vi "Main_Marvin Remake.vi"() -> ()   [LabVIEW 2017]
uses:
  PCAN_Driver/ControlCAN.llb/DevType.ctl
  PCAN_Driver/ControlCAN.llb/CAN Channel.ctl
  PCAN_Driver/ControlCAN.llb/VCI_INIT_CONFIG.ctl
  PCAN_Driver/ControlCAN.llb/InitFlag.ctl
  PCAN_Driver/ControlCAN.llb/Fliter.ctl
  PCAN_Driver/ControlCAN.llb/Mode.ctl
  <vilib>/Utility/miscctls.llb/LVRowAndColumnTypeDef.ctl
  <vilib>/Utility/config.llb/Read Key (String).vi
  <vilib>/Utility/config.llb/Write Key (String).vi
  <vilib>/Utility/cursorutil.llb/Set Cursor (Icon Pict).vi
  PCAN_Driver/ControlCAN.lvlib
  <vilib>/Utility/config.llb/NI_LVConfig.lvlib
panel:
  out "UUT SN Report":string
  out "Automation":bool
  out "Test Failed":bool
  out "AuxiOFFResult":bool
  out "AuxiONResult":bool
  out "SensCalResult":bool
  out "VisualInspectionResult":bool
  out "BurnResult":bool
  out "BurnSpeed":bool
  out "BurnTemp":bool
  out "BurnDC":bool
  out "TempControlResult":bool
  out "MotorTempResult":bool
  out "StopTimeResult":bool
  out "SpeedResult":bool=TRUE
  out "VenableDirectionResult":bool
  out "VenableResult":bool
  out "ComTestResult":bool=TRUE
  out "UUT SoftwareVer":string
  out "Next SN":i32
  in  "SetSN":bool
  out "Current SN":i32
  out "Cal":dbl
  out "AO[1]Meas":dbl
  out "FullSpeed2 Speed":dbl
  out "FullSpeed2 Current":dbl
  out "FullSpeed1 Current":dbl
  out "FullSpeed1 Speed":dbl
  out "MaxBurnInTempVal":dbl
  in  "Stop Burn-in":bool
  out "VISA Tester":refnum<visa-resource-name>
  out "UUT":u8
  out "CAN Status":bool
  in  "Channel 2":T1 caption="Channel" items=["Channel 1", "Channel 2"]
  out "Config_CANAT":T7 {"DevType" items=["USB-CAN"=3, "USB-CAN2"=4]; "CanIndex" items=["通道1", "通道2"]; "VCI_INIT_CONFIG"."Fliter" items=["接收所有类型"=3, "只接收标准帧"=4, "只接收扩展帧"=7]; "VCI_INIT_CONFIG"."Mode" items=["正常工作", "自测模式（环回）", "仅侦听模式"]; "VCI_INIT_CONFIG"."InitFlag" items=["使用Flash参数", "使用界面设置参数"]}
  out "Array":u64[][](array[numeric]) format="%016x"
  out "Motor Phase Current RMS":dbl
  out "Ambient Temperature":dbl
  out "Speed error":bool
  out "Commutation err":bool
  out "Under voltage/Over voltage":bool
  out "Derated drive temp":bool
  out "Motor Over temperature":bool
  out "Motor Sensor temp Fauilre":bool
  out "Drive Over temperature":bool
  out "Drive Sensor temp Failure":bool
  out "Ambient Over temp":bool
  out "Ambient Sensor temp":bool
  out "DC Voltage":dbl
  out "DC Current":dbl
  out "Power transistor Heat sink Temp.":dbl
  out "Motor Stator Temp.":dbl
  out "Motor Speed RPM":dbl
  out "ECS State":u16
  out "UUT":string="EBAY"
  in  "Logger Path":path
  in  "Report":bool
  in  "Start":bool
  in  "ATR":string[][](table)=[["Test Communication", "-", "-", "-", "-", ""], ["Set S/N", "-", "-", "-", "-", ""], ["Set Board Number", "-", "-", "-", "-", ""], [" ", "", "", "", "", ""], ["Test Communication", "-", "-", "-", "-", ""], ["Get S/N", "-", "-", "-", "", ""], ["Get Board Number", "-", "-", "-", "", ""], ["Get FW", "-", "-", "-", "", ""], ["Enable Motor", "", "", "", "", ""], ["Small position command", "", "", "", "", ""], ["Measure delta", "", "", "", "", ""], ["Velocity command", "", "", "", "", ""]]
  in  "Settings":bool
  in  "Refresh Button":bool
  out "Status":bool
  in  "VISA Marvin":refnum<visa-resource-name>="COM6"
  in  "Serial Com":bool
  in  "Help Button":bool
  out "Pannel User Message":string
  in  "Stop Button":bool
  # "Marvin"
  # "REDLER TECHNOLOGIES LTD"
  # "ver 1.2i"
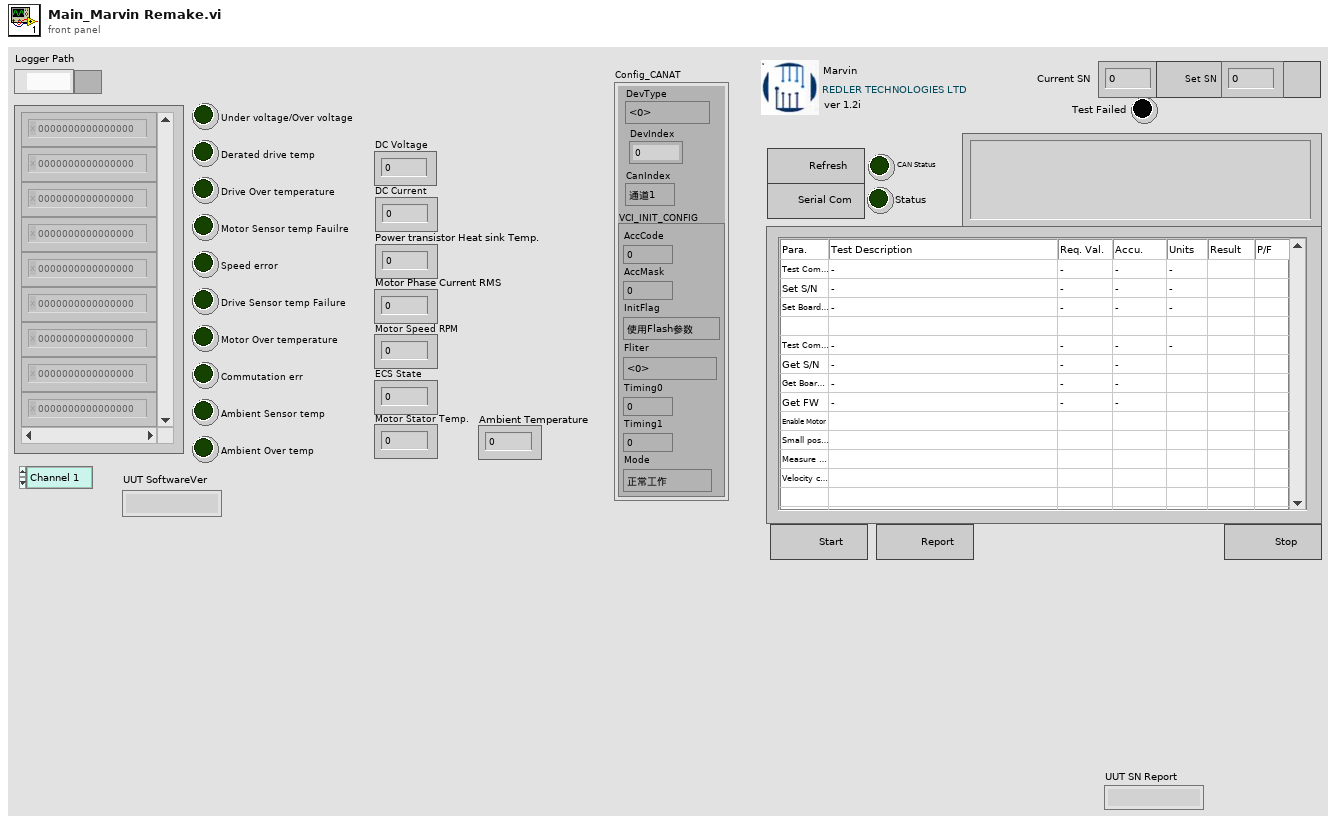
[diagram p1: front panel]
types:
  T1 = typedef "ControlCAN.lvlib/CAN Channel.ctl" = u32
  T2 = typedef "ControlCAN.lvlib/DevType.ctl" = u32
  T3 = typedef "ControlCAN.lvlib/VCI_INIT_CONFIG.ctl" = cluster{"AccCode":u32, "AccMask":u32, "InitFlag":T4, "Fliter":T5, "Timing0":u8, "Timing1":u8, "Mode":T6}
  T4 = typedef "ControlCAN.lvlib/InitFlag.ctl" = u32
  T5 = typedef "ControlCAN.lvlib/Fliter.ctl" = u8
  T6 = typedef "ControlCAN.lvlib/Mode.ctl" = u8
  T7 = cluster{"DevType":T2, "DevIndex":u32, "CanIndex":T1, "VCI_INIT_CONFIG":T3}
  T8 = cluster{"VISA":refnum<visa-resource-name>, "Array Test":enum16{"Auxiliary", "Temp Sens Cal", "Com Test", "Enable Test", "Speed Command", "Stop Time", "Temp Control", "Burn in", "Visual Inspec", "Empty"}[]}
  T9 = cluster{"ID":u32, "MSGTYPE":u8, "LEN":u8, "aDATA":u8[]}[]
  T10 = enum16{"Erase ATR Table", "Stop", "MainProgram", "Initialize"}
  T11 = enum16{"K15", "K16", "K17", "Venable", "Firmeware", "Fan", "Power", "120C", "110C", "100C", "90C", "80C", "70C", "60C", "50C", "40C", "30C", "25C", "20C", "10C", "0C"}
  T12 = enum16{"Stop", "Result", "FullSpeed2", "MD[1]=1", "FullSpeed1", "MD[1]=0"}
  T13 = enum8{"Term1", "Term2", "Current", "Fan", "TempCPU"}
  T14 = enum16{"Stop", "AO[1]=Meas.", "TA[5]", "AO[1]=0", "Start"}
  T15 = enum16{"Stop", "BurnIn", "Ambient Temp", "MotorSpeed", "DC Current Measure", "Start"}
  T16 = enum16{"Auxiliary", "Temp Sens Cal", "Com Test", "Enable Test", "Speed Command", "Stop Time", "Temp Control", "Burn in", "Visual Inspec", "Empty"}[]
  T17 = enum16{"K15", "K16", "K17", "Venable", "Firmeware", "Fan", "Power", "120C", "110C", "100C", "90C", "80C", "70C", "60C", "50C", "40C", "30C", "25C", "20C", "10C", "0C"}[]
  T18 = enum8{"Enabled", "Disabled", "Disabled and Grayed Out"}
  T19 = typedef "LVRowAndColumnTypeDef.ctl" = cluster{"Row":i32, "Column":i32}
  T20 = enum16{"Auxiliary", "Temp Sens Cal", "Com Test", "Enable Test", "Speed Command", "Stop Time", "Temp Control", "Burn in", "Visual Inspec", "Empty"}
  T21 = cluster{"ID":u32, "MSGTYPE":u8, "LEN":u8, "aDATA":u8[]}
  T22 = enum16{"open", "replace", "create", "open or create", "replace or create", "replace or create with confirmation"}
  T23 = enum32{"Invalid", "Standard", "Closed", "Hidden", "Minimized", "Maximized"}
  T24 = typedef "NI_LVConfig.lvlib/Config Data RefNum.ctl" = refnum<k1>
  T25 = typedef "ControlCAN.lvlib/VCI_CAN_OBJ.ctl" = cluster{"ID":u32, "TimeStamp":u32, "TimeFlag":u8, "SendType":u8, "RemoteFlag":u8, "ExternFlag":u8, "DataLen":u8, "Data":u8[], "Reserved":u8[]}
  T26 = cluster{"Type":enum16{"接收", "发送"}, "Channel":T1, "Time":timestamp, "VCI_CAN_OBJ":T25}[]
  T27 = cluster{"Type":enum16{"接收", "发送"}, "Channel":T1, "Time":timestamp, "VCI_CAN_OBJ":T25}
  T28 = typedef "LVPoint32TypeDef.ctl" = cluster{"Horizontal":i32, "Vertical":i32}
  T29 = enum8{"Term1", "Term2", "Current", "Fan", "TempCPU"}[]
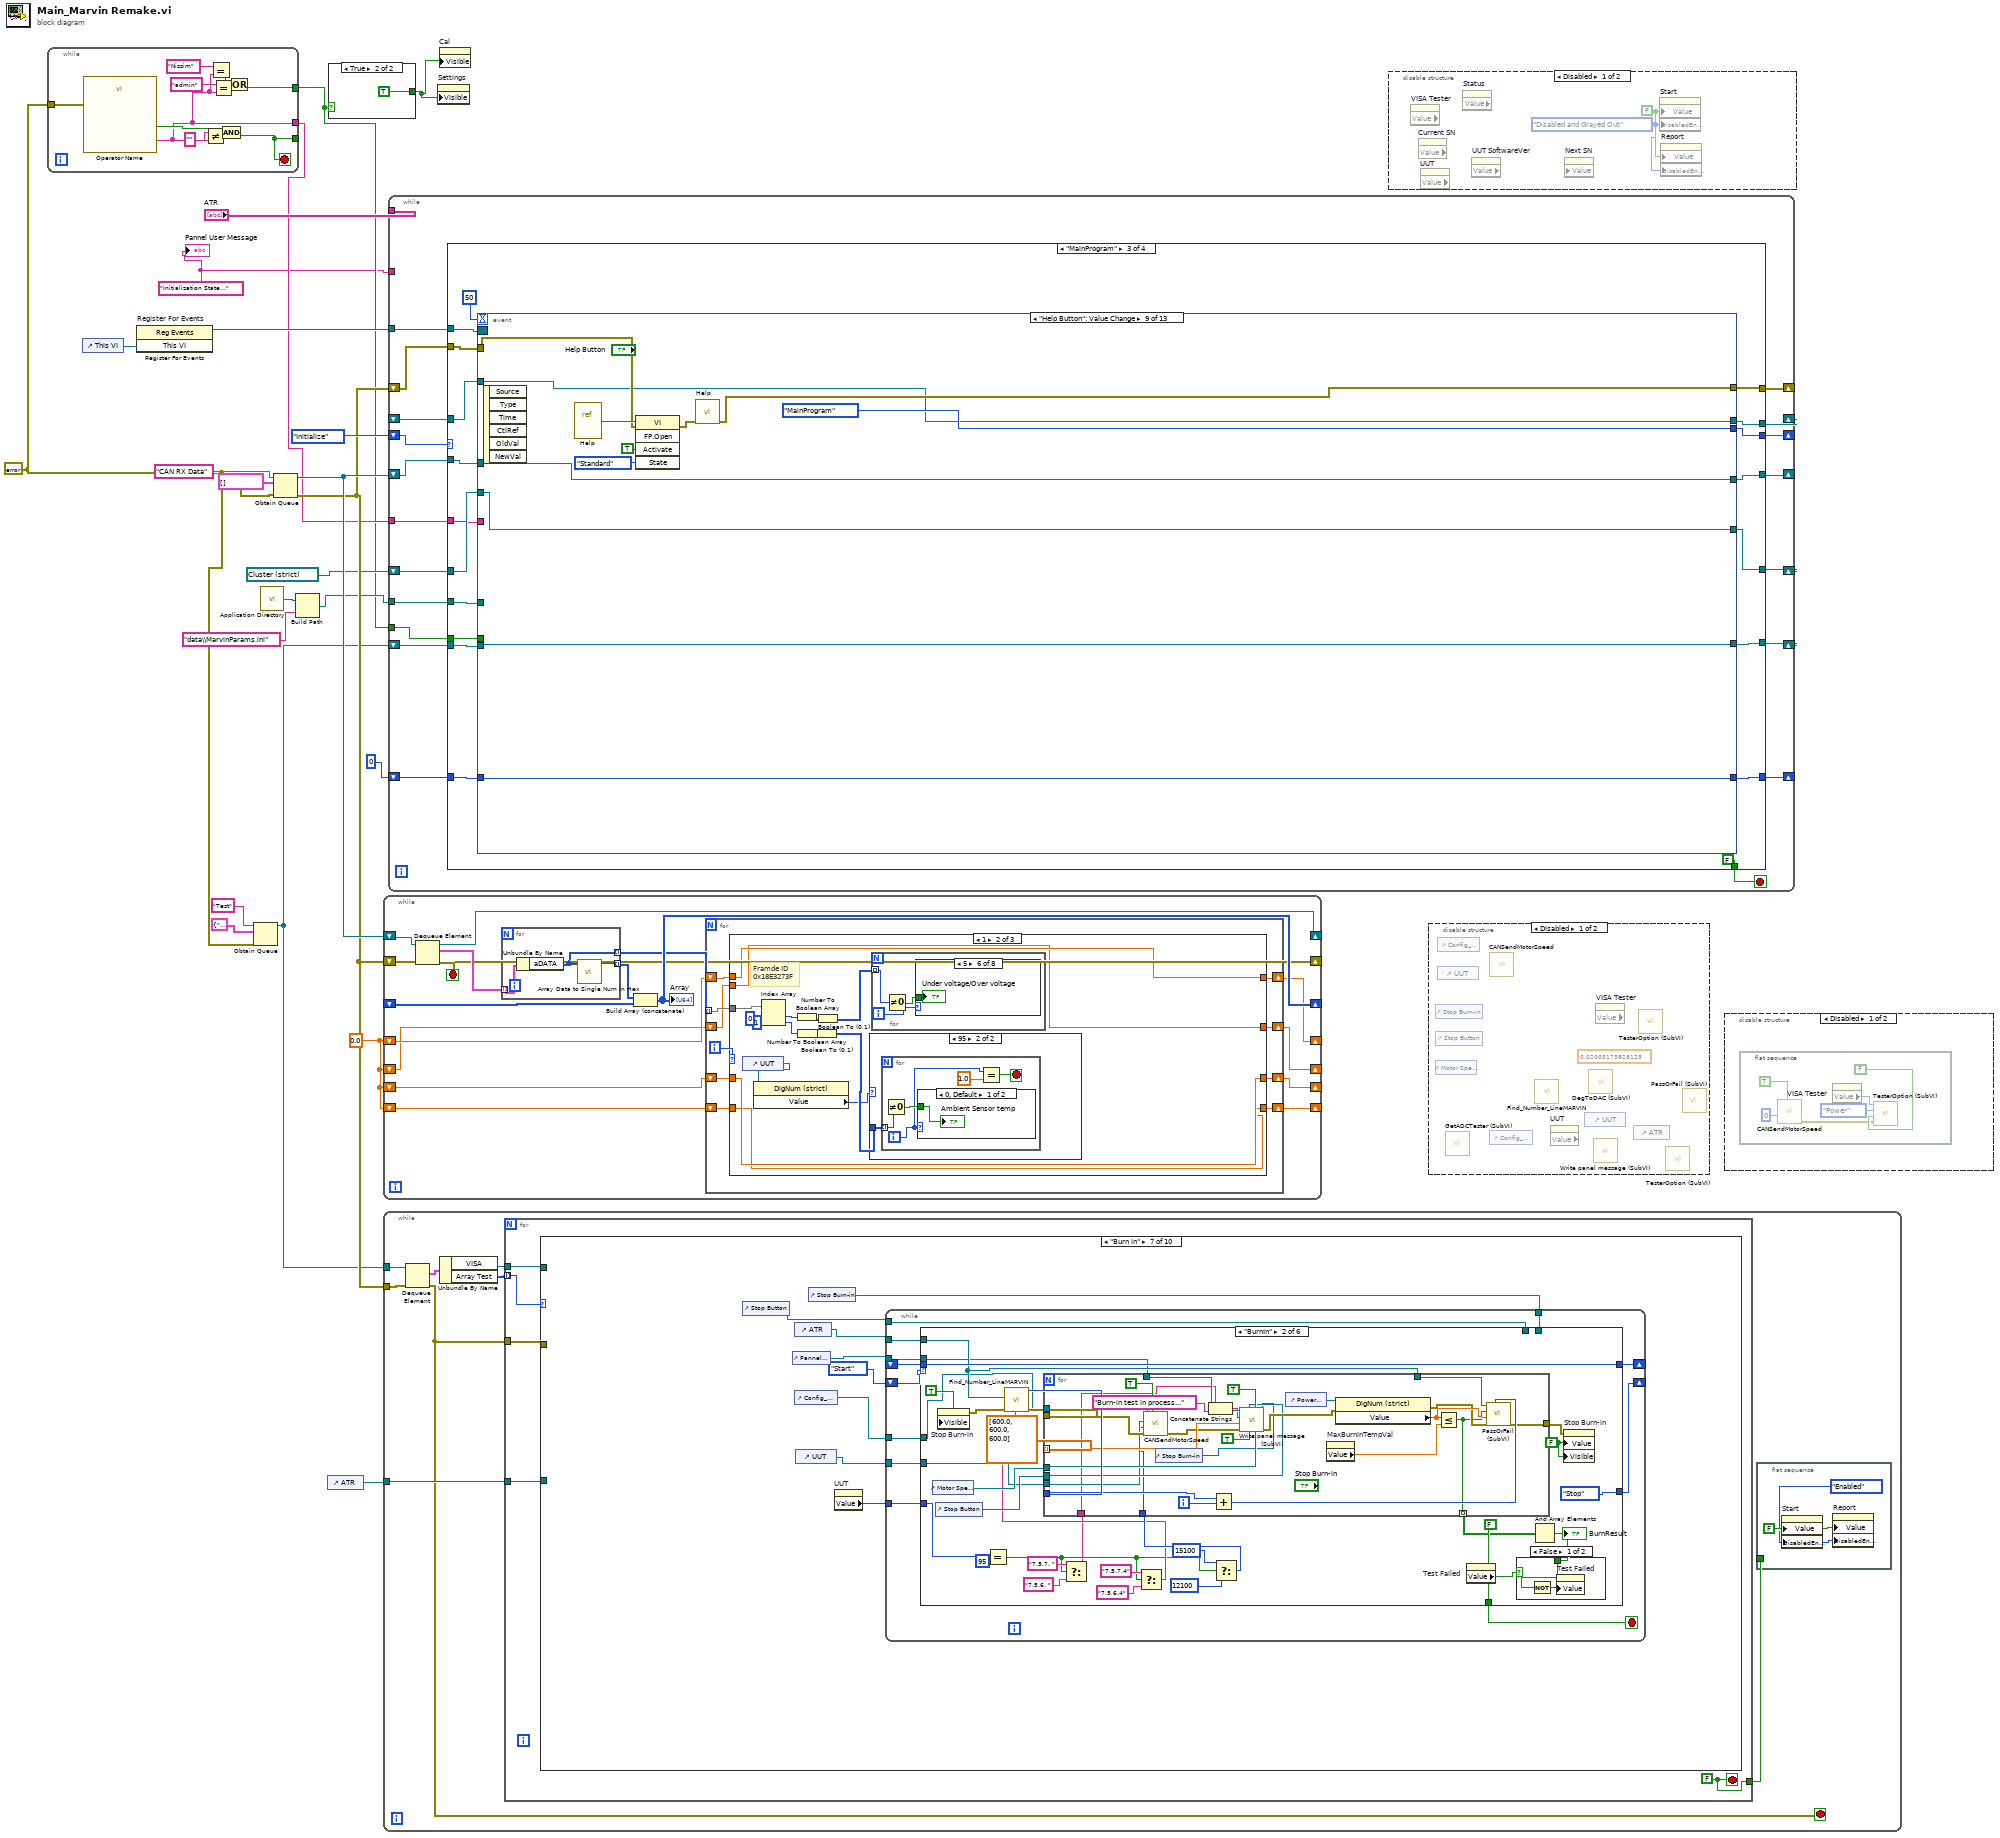
[diagram p0: block diagram]
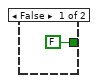
[diagram p2: hidden frame]
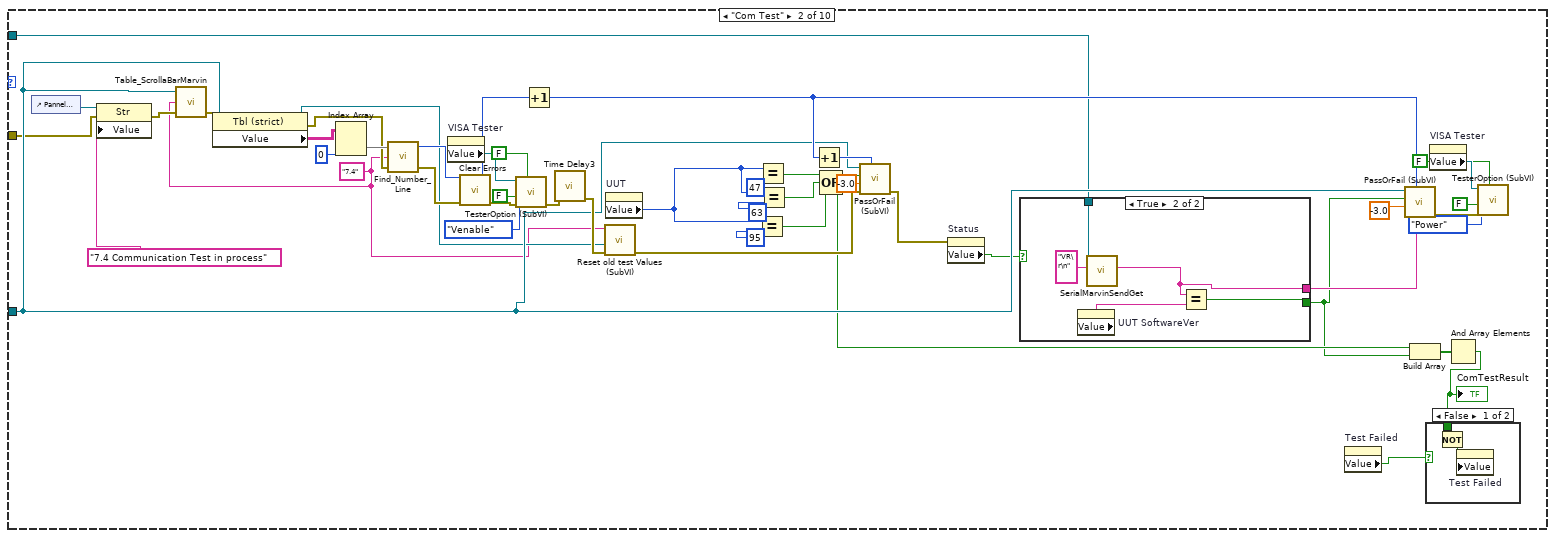
[diagram p7: hidden frame]
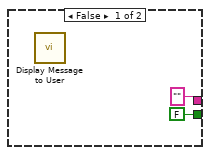
[diagram p9: hidden frame]
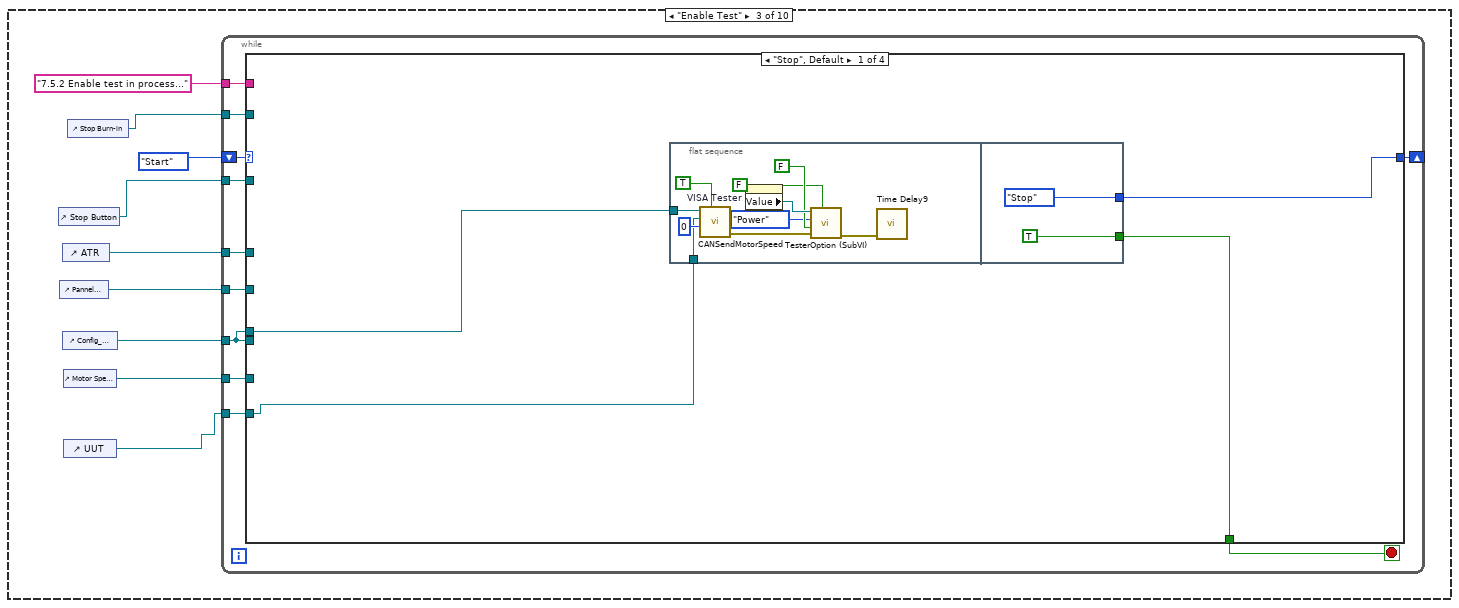
[diagram p10: hidden frame]
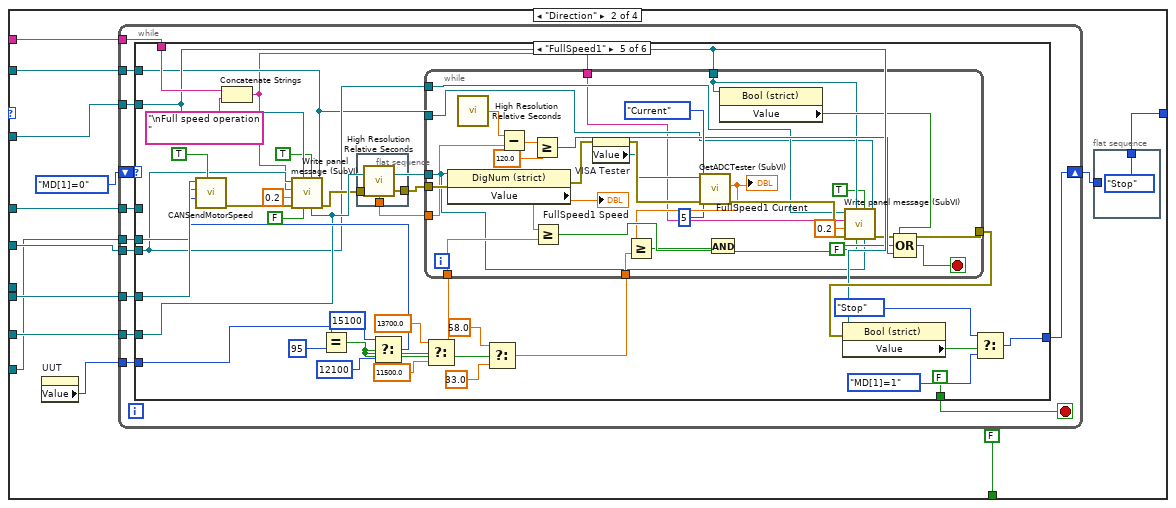
[diagram p11: hidden frame]
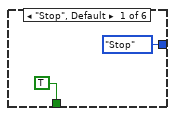
[diagram p12: hidden frame]
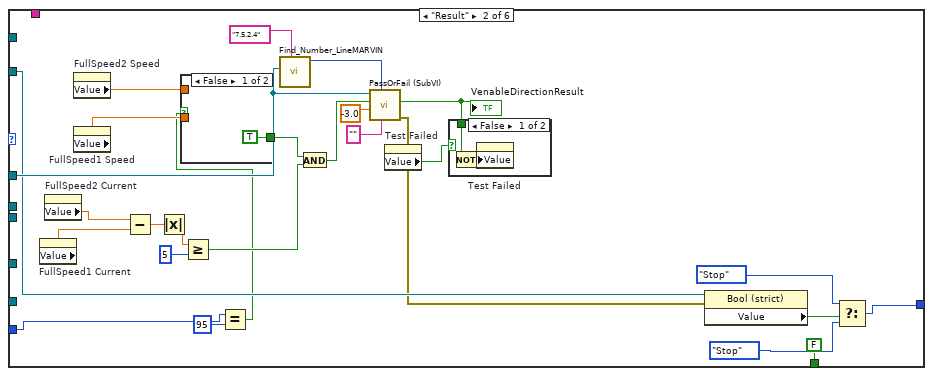
[diagram p13: hidden frame]
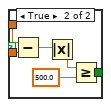
[diagram p15: hidden frame]
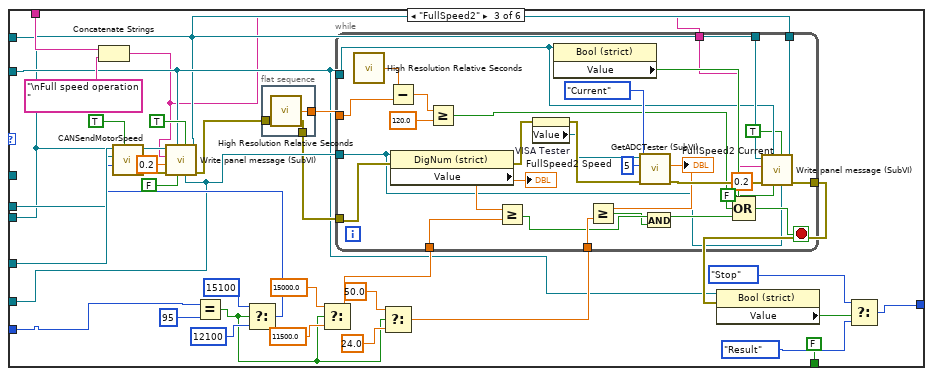
[diagram p16: hidden frame]
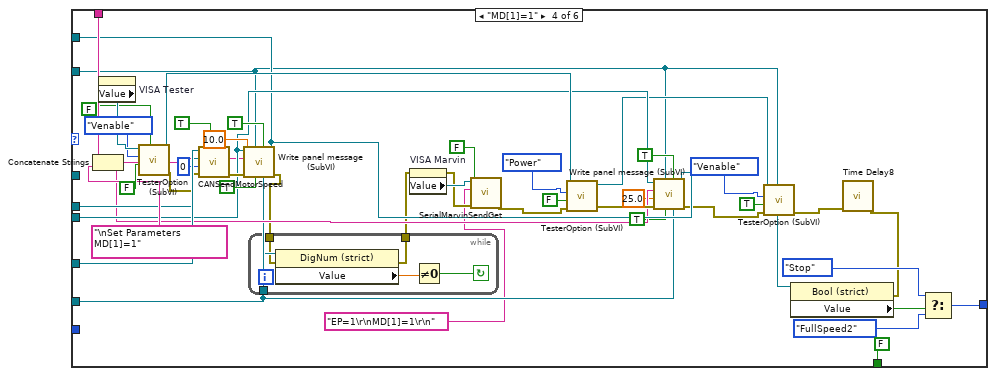
[diagram p17: hidden frame]
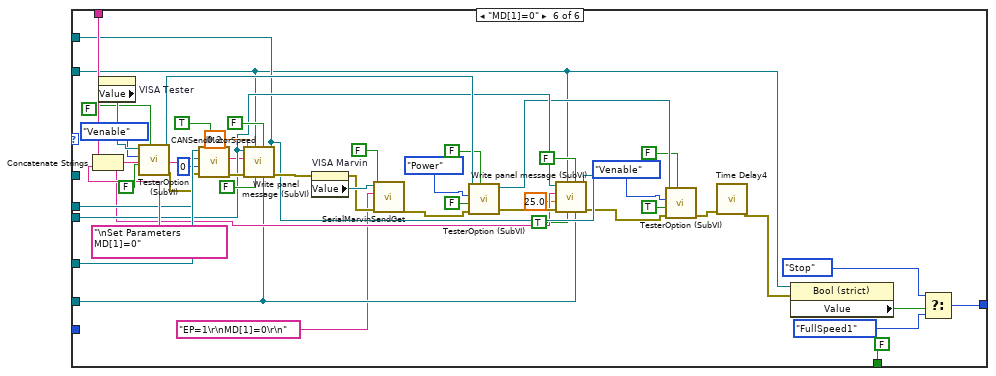
[diagram p18: hidden frame]
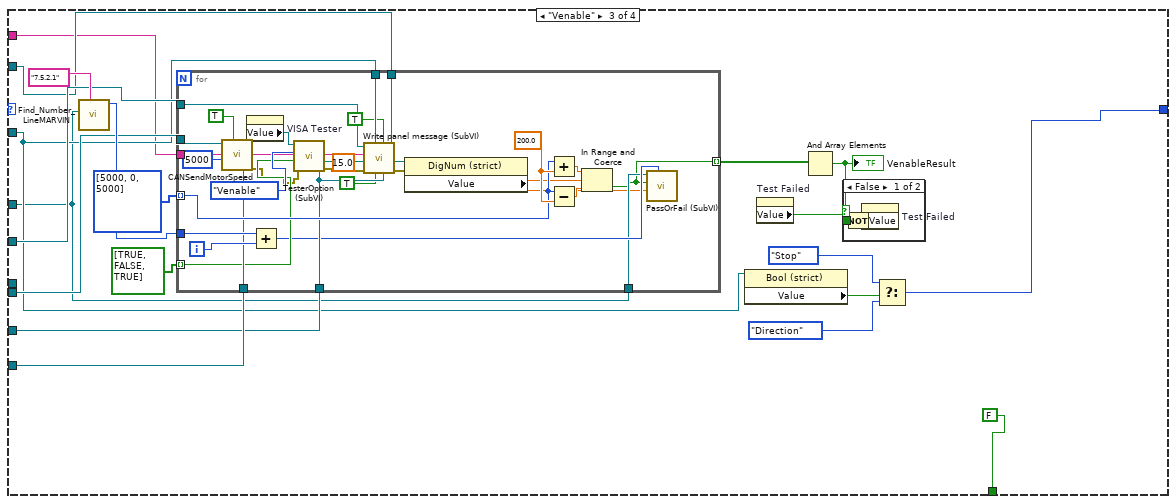
[diagram p19: hidden frame]
diagram:
  w1 = "Initialization State..."
  w12 = 0.0
  w11 = errorcluster {"status"=FALSE, "code"=0, "source"=""} ("error in (no error)")
  n1 = while {
    tunnel: [w31] -> _
    tunnel: [w27] -> w6
    tunnel: [w28] -> w2
    tunnel: w11 -> [w24]
    stop <- w31 stop-if-true
    n2 = call "Operator Name"("error in (no error)"=w24) -> ("Operator Name"=w27:string, "OK"=w32:bool)  [unwired: 16 in, 1 out]
    n3 = Not Equal?(x=w27, y="") -> (x != y?=w33:bool)
    n4 = Equal?(x="Nissim", y=w27) -> (x = y?=w25:bool)
    n5 = Equal?(x="admin", y=w27) -> (x = y?=w29:bool)
    n6 = And(x=w32, y=w33) -> (x .and. y?=w31:bool)
    n7 = Or(x=w25, y=w29) -> (x .or. y?=w28:bool)
  }
  n8 = control-ref of="This VI"() -> (w8:refnum<vi>)
  n9 = register-events "Register For Events"(w8) -> (reference out=w7:refnum<event-registration>)  [unwired: 2 in, 1 out]
  n10 = Obtain Queue(name (unnamed)="Test", element data type=T8 {"VISA"="COM1", "Array Test"=[]}, error in (no error)=w11) -> (queue out=w16:refnum<queue>)  [unwired: 2 in, 2 out]
  n11 = call <vilib>:"Application Directory.vi"() -> ("Application Directory"=w10:path)
  n12 = Obtain Queue(name (unnamed)="CAN RX Data", element data type=T9 [], error in (no error)=w11) -> (queue out=w20:refnum<queue>, error out=w17:errorcluster)  [unwired: 2 in, 1 out]
  n13 = Build Path(base path=w10, name or relative path="data\\MarvinParams.ini") -> (appended path=w4:path)
  n14 = control-ref of="ATR"() -> (w18:refnum<vi>)
  n15 = case shown="True" w2 {
    tunnel: [FALSE TRUE] -> w3
    frame False {
    }
    frame True {
    }
  }
  n16 = while {
    shift-right: [w51] -> _
    shift-left: w20 -> [w53]
    shift-right: [w49] -> _
    shift-left: _ -> [w50]
    shift-right: [w45] -> _
    shift-left: w17 -> [w45]
    shift-right: [w43] -> _
    shift-left: w12 -> [w44]
    shift-right: [w42] -> _
    shift-left: w12 -> [w41]
    shift-right: [w40] -> _
    shift-left: w12 -> [w39]
    shift-right: [w38] -> _
    shift-left: w12 -> [w37]
    stop <- w52 stop-if-true
    n17 = Dequeue Element(queue=w53, error in (no error)=w45) -> (queue out=w51:refnum<queue>, element=w46:T9, error out=w52:errorcluster)  [unwired: 1 in, 1 out]
    n18 = for {
      tunnel: [w182] -> w48 mode=indexing
      tunnel: w46 -> [w181] mode=indexing
      tunnel: [w180] -> w47 mode=indexing
      n19 = Unbundle By Name(w181) -> ("aDATA"=w180:u8[])
      n20 = call "Array Data to Single Num in Hex.vi"("aDATA"=w180) -> ("Numeric"=w182:u64)  [unwired: 10 in]
    }
    n21 = Build Array (concatenate)(w48, w50) -> (w49:u64[][])
    "Array" <- w49
    n22 = for {
      tunnel: w47 -> [w63] mode=indexing
      shift-right: [w60] -> w43
      shift-left: w44 -> [w61]
      shift-right: [w59] -> w42
      shift-left: w41 -> [w58]
      shift-right: [w57] -> w40
      shift-left: w39 -> [w56]
      shift-right: [w55] -> w38
      shift-left: w37 -> [w54]
      i -> [w62]
      n23 = case shown="1" w62 {
        tunnel: w63 -> [w103 w136 w175]
        tunnel: w61 -> [w77 w125 w164]
        tunnel: [w75 w125 w164] -> w60
        tunnel: [w72 w124 w163] -> w59
        tunnel: w58 -> [w71 w124 w163]
        tunnel: [w66 w123 w162] -> w57
        tunnel: w56 -> [w65 w123 w162]
        tunnel: [w64 w122 w157] -> w55
        tunnel: w54 -> [w64 w122 w156]
        frame 0, Default {
          # "Frame ID\n0x18E1273F"
          n24 = Index Array(array=w103, index #1=0 ("index"), index #2=1 ("index"), index #3=2 ("index"), index #4=3 ("index"), index #5=4 ("index"), index #6=5 ("index"), index #7=6 ("index"), index #8=7 ("index")) -> (element #1=w87:u8, element #2=w89:u8, element #3=w90:u8, element #4=w94:u8, element #5=w97:u8, element #6=w101:u8, element #7=w102:u8, element #8=w100:u8)
          n25 = Number To Hexadecimal String(2:w100) -> (0:w114:string)  [unwired: 1 in]
          n26 = Join Numbers(hi=w102, lo=w101) -> ((hi.lo)=w121:u16)
          n27 = Join Numbers(hi=w90, lo=w89) -> ((hi.lo)=w91:u16)
          n28 = Number To Hexadecimal String(2:w97) -> (0:w98:string)  [unwired: 1 in]
          n29 = Number To Hexadecimal String(2:w121) -> (0:w120:string)  [unwired: 1 in]
          n30 = Number To Hexadecimal String(2:w87) -> (0:w88:string)  [unwired: 1 in]
          n31 = Number To Hexadecimal String(2:w91) -> (0:w92:string)  [unwired: 1 in]
          n32 = Number To Hexadecimal String(2:w94) -> (0:w95:string)  [unwired: 1 in]
          n33 = Hexadecimal String To Number(string=w114) -> (number=w113:u32)  [unwired: 2 in, 1 out]
          n34 = To Double Precision Float(number=w113) -> (double precision float=→"DC Current":dbl)
          n35 = Hexadecimal String To Number(string=w98) -> (number=w99:u32)  [unwired: 2 in, 1 out]
          n36 = Hexadecimal String To Number(string=w120) -> (number=w119:u32)  [unwired: 2 in, 1 out]
          n37 = Hexadecimal String To Number(string=w88) -> (number=w85:u32)  [unwired: 2 in, 1 out]
          n38 = Hexadecimal String To Number(string=w92) -> (number=w93:u32)  [unwired: 2 in, 1 out]
          n39 = Hexadecimal String To Number(string=w95) -> (number=w96:u32)  [unwired: 2 in, 1 out]
          n40 = To Double Precision Float(number=u32 10 ("y")) -> (double precision float=w117:dbl)
          n41 = To Double Precision Float(number=w119) -> (double precision float=w116:dbl)
          n42 = To Double Precision Float(number=w99) -> (double precision float=w82:dbl)
          n43 = To Double Precision Float(number=w93) -> (double precision float=w78:dbl)
          n44 = To Double Precision Float(number=w96) -> (double precision float=w84:dbl)
          n45 = Divide(x=w116, y=w117) -> (x/y=→"DC Voltage":dbl)
          n46 = To Unsigned Word Integer(number=w85) -> (unsigned 16bit integer=→"ECS State":u16)
          n47 = Subtract(x=w82, y=50.0 ("x")) -> (x-y=w70:dbl)
          n48 = Subtract(x=w84, y=50.0 ("x")) -> (x-y=w73:dbl)
          n49 = call "Filter (SubVI).vi"("Delta"=5000.0, "NewVal"=w78, "OldVal"=w77) -> ("Val"=w75:dbl)  [unwired: 8 in]
          "Motor Speed RPM" <- w75
          n50 = Less Than 0?(x=w73) -> (x < 0?=w80:bool)
          n51 = Less Than 0?(x=w70) -> (x < 0?=w79:bool)
          n52 = Select(t=w71, s=w80, f=w73) -> (s? t:f=w74:dbl)
          n53 = Select(t=w65, s=w79, f=w70) -> (s? t:f=w69:dbl)
          n54 = call "Filter (SubVI).vi"("Delta"=130.0, "NewVal"=w74, "OldVal"=w71) -> ("Val"=w72:dbl)  [unwired: 8 in]
          "Motor Stator Temp." <- w72
          n55 = call "Filter (SubVI).vi"("Delta"=100.0, "NewVal"=w69, "OldVal"=w65) -> ("Val"=w66:dbl)  [unwired: 8 in]
          "Power transistor Heat sink Temp." <- w66
        }
        frame 1 {
          # "Framde ID\n0x18E3273F"
          n56 = control-ref of="UUT"() -> (w126:refnum<vi>)
          n57 = property on="Property Node" class="DigNum (strict)"(reference=w126) -> ("Value"=w127:u8)  [unwired: 1 in, 2 out]
          n58 = Index Array(array=w136, index #1=0 ("index"), index #2=1 ("index")) -> (element #1=w134:u8, element #2=w129:u8)
          n59 = Number To Boolean Array(number=w134) -> (Boolean array=w133:bool[])
          n60 = Number To Boolean Array(number=w129) -> (Boolean array=w131:bool[])
          n61 = Boolean To (0,1)(Boolean=w131) -> (0, 1=w128:i16[])
          n62 = Boolean To (0,1)(Boolean=w133) -> (0, 1=w132:i16[])
          n63 = case shown="95" w127 {
            tunnel: w128 -> [_ w137]
            frame 0, Default {
            }
            frame 95 {
              n64 = for {
                tunnel: w137 -> [w142] mode=indexing
                i -> [w138]
                stop <- w140 stop-if-true
                n65 = Not Equal To 0?(x=w142) -> (x != 0?=w141:bool)
                n66 = case shown="0, Default" w138 {
                  tunnel: w141 -> [w143 w144]
                  frame 0, Default {
                    "Ambient Sensor temp" <- w143
                  }
                  frame 1 {
                    "Ambient Over temp" <- w144
                  }
                }
                n67 = Equal?(x=w138, y=1.0) -> (x = y?=w140:bool)
              }
            }
          }
          n68 = for {
            tunnel: w132 -> [w146] mode=indexing
            i -> [w147]
            n69 = Not Equal To 0?(x=w146) -> (x != 0?=w145:bool)
            n70 = case shown="5" w147 {
              tunnel: w145 -> [w148 w149 w150 w151 w152 w153 w154 w155]
              frame 0, Default {
                "Drive Sensor temp Failure" <- w148
              }
              frame 1 {
                "Drive Over temperature" <- w149
              }
              frame 2 {
                "Motor Sensor temp Fauilre" <- w150
              }
              frame 3 {
                "Motor Over temperature" <- w151
              }
              frame 4 {
                "Derated drive temp" <- w152
              }
              frame 5 {
                "Under voltage/Over voltage" <- w153
              }
              frame 6 {
                "Commutation err" <- w154
              }
              frame 7 {
                "Speed error" <- w155
              }
            }
          }
        }
        frame 2 {
          # "Frame ID\n0x18E2273F"
          n71 = Index Array(array=w175, index #1=0 ("index"), index #2=1 ("index")) -> (element #1=w172:u8, element #2=w169:u8)
          n72 = disable-structure shown="Enabled" {
            disable-tunnel: [w178 w179] -> w173
            disable-tunnel: w172 -> [w177 w179]
            frame Disabled {
              n73 = Number To Hexadecimal String(2:w177) -> (0:w176:string)  [unwired: 1 in]
              n74 = Hexadecimal String To Number(string=w176) -> (number=w178:u32)  [unwired: 2 in, 1 out]
            }
            frame Enabled {
            }
          }
          n75 = Number To Hexadecimal String(2:w169) -> (0:w167:string)  [unwired: 1 in]
          n76 = Hexadecimal String To Number(string=w167) -> (number=w168:u32)  [unwired: 2 in, 1 out]
          n77 = To Double Precision Float(number=w168) -> (double precision float=w166:dbl)
          n78 = To Double Precision Float(number=w173) -> (double precision float=→"Motor Phase Current RMS":dbl)
          n79 = Subtract(x=w166, y=50.0) -> (x-y=w160:dbl)
          n80 = Less Than 0?(x=w160) -> (x < 0?=w161:bool)
          n81 = Select(t=w156, s=w161, f=w160) -> (s? t:f=w159:dbl)
          n82 = call "Filter (SubVI).vi"("Delta"=65.0, "NewVal"=w159, "OldVal"=w156) -> ("Val"=w157:dbl)  [unwired: 8 in]
          "Ambient Temperature" <- w157
        }
      }
    }
  }
  n83 = while {
    tunnel: w18 -> [w190]
    tunnel: w17 -> [w188]
    tunnel: w16 -> [w189]
    stop <- w184 stop-if-true
    n84 = Dequeue Element(queue=w189, error in (no error)=w188) -> (element=w187:T8, error out=w184:errorcluster)  [unwired: 1 in, 2 out]
    n85 = Unbundle By Name(w187) -> ("VISA"=w186:refnum<visa-resource-name>, "Array Test"=w185:T16)
    n86 = for {
      tunnel: w185 -> [w194] mode=indexing
      tunnel: w186 -> [w197]
      tunnel: w190 -> [w196]
      tunnel: w184 -> [w195]
      tunnel: [w193] -> w183
      stop <- w193 stop-if-true
      w193 = FALSE
      n87 = case shown="\"Burn in\"" w194 {
        tunnel: w197 -> [_ w223 _ _ w828 _ _ _ w1392 _]
        tunnel: w196 -> [_ w230 _ w657 w824 w990 _ w1382 w1399 w1613]
        tunnel: w195 -> [_ w227 _ w672 w834 w988 _ w1381 w1397 w1612]
        frame "Empty", Default {
        }
        frame "Com Test" {
          w203 = "7.4" ("Test Paragraph")
          n88 = control-ref of="Pannel User Message"() -> (w228:refnum<vi>)
          n89 = property class="Str"(reference=w228, error in=w227, "Value"="7.4 Communication Test in process") -> (error out=w226:errorcluster)  [unwired: 1 out]
          n90 = call "Table_ScrollaBarMarvin.vi"("error in"=w226, "Line to focus"=w203, "reference in"=w230) -> ("error out"=w229:errorcluster)  [unwired: 2 out]
          n91 = property class="Tbl (strict)"(reference=w230, error in=w229) -> (reference out=w204:refnum<vi>, error out=w242:errorcluster, "Value"=w243:string[][])
          n92 = Index Array(array=w243, index (col)=0 ("disabled index (col)")) -> (element=w244:string[])  [unwired: 1 in]
          n93 = call "Find_Number_Line.vi"("error in"=w242, "Test Paragraph"=w203, "Row Headers[]"=w244) -> ("error out"=w240:errorcluster, "Line number"=w239:i32)  [unwired: 1 out]
          n94 = property on="VISA Tester" class="VISAName"() -> ("Value"=w216:refnum<visa-resource-name>)  [unwired: 2 in, 2 out]
          n95 = call <vilib>:"Clear Errors.vi"("error in (no error)"=w240) -> ("error out"=w218:errorcluster)  [unwired: 5 in, 1 out]
          n96 = call "TesterOption (SubVI).vi"("2 Options"=FALSE, "error in (no error)"=w218, "On/Off"=FALSE, "Tester Option"=T11."Venable", "VISA Refnum in"=w216) -> ("error out"=w217:errorcluster)  [unwired: 5 in, 1 out]
          n97 = Increment(x=w239) -> (x+1=w233:i32)
          n98 = call "Time Delay3"("error in (no error)"=w217) -> ("error out"=w231:errorcluster)  [unwired: 10 in]
          n99 = call "Reset old test Values (SubVI).vi"("error in"=w231, "Atr in"=w204, "Test Paragraph"=w203) -> ("error out"=w205:errorcluster)  [unwired: 8 in]
          n100 = property on="UUT" class="DigNum (strict)"() -> ("Value"=w206:u8)  [unwired: 2 in, 2 out]
          n101 = Equal?(x=w206, y=u8 95) -> (x = y?=w221:bool)
          n102 = Equal?(x=w206, y=u8 47) -> (x = y?=w235:bool)
          n103 = Equal?(x=w206, y=u8 63) -> (x = y?=w234:bool)
          n104 = Increment(x=w233) -> (x+1=w232:i32)
          n105 = Compound Arithmetic op=OR(w235, w234, w221) -> (w201:bool)
          n106 = call "PassOrFail (SubVI).vi"("index (row)"=w232, "error in (no error)"=w205, "Data in"=-3.0, "Pass?Fail"=w201, "Table in"=w230) -> ("error out"=w222:errorcluster)  [unwired: 6 in]
          n107 = property on="Status" class="Bool (strict)"(error in=w222) -> ("Value"=w224:bool)  [unwired: 1 in, 2 out]
          n108 = case shown="True" w224 {
            tunnel: w223 -> [_ w253]
            tunnel: [FALSE w250] -> w200
            tunnel: ["" ("read buffer") w249] -> w220
            frame False {
              n109 = call "Display Message to User"() -> ()  [unwired: 10 in, 2 out]
            }
            frame True {
              n110 = property on="UUT SoftwareVer" class="Str"() -> ("Value"=w251:string)  [unwired: 2 in, 2 out]
              n111 = call "SerialMarvinSendGet.vi"("write buffer"="VR\r\n", "VISA resource name"=w253) -> ("read buffer"=w249:string)  [unwired: 8 in, 1 out]
              n112 = Equal?(x=w249, y=w251) -> (x = y?=w250:bool)
            }
          }
          n113 = property on="Test Failed" class="Bool (strict)"() -> ("Value"=w198:bool)  [unwired: 2 in, 2 out]
          n114 = call "PassOrFail (SubVI).vi"("String Res"=w220, "index (row)"=w233, "Data in"=-3.0, "Pass?Fail"=w200, "Table in"=w230) -> ("error out"=w212:errorcluster)  [unwired: 6 in]
          n115 = Build Array(w201, w200) -> (w202:bool[])
          n116 = property on="VISA Tester" class="VISAName"() -> ("Value"=w211:refnum<visa-resource-name>)  [unwired: 2 in, 2 out]
          n117 = And Array Elements(Boolean array=w202) -> (logical AND=w199:bool)
          "ComTestResult" <- w199
          n118 = case shown="False" w198 {
            tunnel: w199 -> [w246 _]
            frame False {
              n119 = Not(x=w246) -> (.not. x?=w245:bool)
              n120 = property on="Test Failed" class="Bool (strict)"("Value"=w245) -> ()  [unwired: 2 in, 2 out]
            }
            frame True {
            }
          }
          n121 = call "TesterOption (SubVI).vi"("2 Options"=FALSE, "error in (no error)"=w212, "On/Off"=FALSE, "Tester Option"=T11."Power", "VISA Refnum in"=w211) -> ()  [unwired: 5 in, 2 out]
        }
        frame "Enable Test" {
          n122 = control-ref of="Stop Button"() -> (w256:refnum<vi>)
          n123 = control-ref of="Pannel User Message"() -> (w258:refnum<vi>)
          n124 = control-ref of="ATR"() -> (w257:refnum<vi>)
          n125 = control-ref of="Config_CANAT"() -> (w259:refnum<vi>)
          n126 = control-ref of="Motor Speed RPM"() -> (w260:refnum<vi>)
          n127 = control-ref of="UUT"() -> (w261:refnum<vi>)
          n128 = control-ref of="Stop Burn-in"() -> (w262:refnum<vi>)
          n129 = while {
            shift-right: [w267] -> _
            shift-left: enum16{"Stop", "Direction", "Venable", "Start"}."Start" -> [w273]
            tunnel: w256 -> [w272]
            tunnel: w257 -> [w271]
            tunnel: w258 -> [w270]
            tunnel: w259 -> [w263]
            tunnel: w260 -> [w269]
            tunnel: w261 -> [w264]
            tunnel: w262 -> [w266]
            tunnel: "7.5.2 Enable test in process..." ("Strin") -> [w265]
            stop <- w268 stop-if-true
            n130 = case shown="\"Stop\", Default" w273 {
              tunnel: w272 -> [_ w300 w589 w636]
              tunnel: w271 -> [_ w295 w587 w643]
              tunnel: w270 -> [_ w298 w591 w642]
              tunnel: w263 -> [_ w301 w594 _]
              tunnel: w269 -> [_ w297 w592 w634]
              tunnel: w264 -> [w274 w291 w593 _]
              tunnel: [w277 FALSE FALSE FALSE] -> w268
              tunnel: [w275 w294 w588 w640] -> w267
              tunnel: w266 -> [_ w299 w590 w635]
              tunnel: w265 -> [_ w296 w586 w633]
              tunnel: w263 -> [w276 _ _ _]
              frame "Stop", Default {
                n131 = flat-sequence {
                  tunnel: w274 -> [w283]
                  tunnel: w276 -> [w282]
                  tunnel: [TRUE] -> w277
                  tunnel: [enum16{"Stop", "Direction", "Venable", "Start"}."Stop"] -> w275
                  frame #0 {
                    n132 = call "CANSendMotorSpeed.vi"("Remote"=TRUE, "Motor Speed RPM"=u16 0, "UUT"=w283, "CAN Cluster in"=w282) -> ("error out"=w286:errorcluster)  [unwired: 7 in]
                    n133 = property on="VISA Tester" class="VISAName"() -> ("Value"=w287:refnum<visa-resource-name>)  [unwired: 2 in, 2 out]
                    n134 = call "TesterOption (SubVI).vi"("2 Options"=FALSE, "error in (no error)"=w286, "On/Off"=FALSE, "Tester Option"=T11."Power", "VISA Refnum in"=w287) -> ("error out"=w278:errorcluster)  [unwired: 5 in, 1 out]
                    n135 = call "Time Delay9"("error in (no error)"=w278) -> ()  [unwired: 10 in, 1 out]
                  }
                  frame #1 {
                  }
                }
              }
              frame "Direction" {
                n136 = property on="UUT" class="DigNum (strict)"() -> ("Value"=w290:u8)  [unwired: 2 in, 2 out]
                n137 = while {
                  shift-right: [w314] -> w293
                  shift-left: T12."MD[1]=0" -> [w315]
                  tunnel: w301 -> [w312]
                  tunnel: w291 -> [w311]
                  tunnel: w300 -> [w310]
                  tunnel: w299 -> [w309]
                  tunnel: w298 -> [w308]
                  tunnel: w297 -> [w307]
                  tunnel: w296 -> [w306]
                  tunnel: w295 -> [w305]
                  tunnel: w290 -> [w304]
                  stop <- w313 stop-if-true
                  n138 = case shown="\"FullSpeed1\"" w315 {
                    tunnel: [T12."Stop" w340 w384 w463 w501 w581] -> w314
                    tunnel: [TRUE FALSE FALSE FALSE FALSE FALSE] -> w313
                    tunnel: w312 -> [_ _ w382 w457 w499 w575]
                    tunnel: w311 -> [_ _ w378 w436 w495 w553]
                    tunnel: w310 -> [_ w327 w357 w427 w477 w543]
                    tunnel: w309 -> [_ _ w355 w437 w475 w554]
                    tunnel: w308 -> [_ _ w356 w438 w476 w555]
                    tunnel: w307 -> [_ _ w373 w425 w491 w549]
                    tunnel: w306 -> [_ _ w368 w446 w489 w563]
                    tunnel: w305 -> [_ w331 _ _ _ _]
                    tunnel: w304 -> [_ w318 w353 _ w470 _]
                    frame "Stop", Default {
                    }
                    frame "Result" {
                      n139 = property on="FullSpeed1 Current" class="DigNum (strict)"() -> ("Value"=w335:dbl)  [unwired: 2 in, 2 out]
                      n140 = property on="FullSpeed2 Current" class="DigNum (strict)"() -> ("Value"=w336:dbl)  [unwired: 2 in, 2 out]
                      n141 = property on="FullSpeed2 Speed" class="DigNum (strict)"() -> ("Value"=w338:dbl)  [unwired: 2 in, 2 out]
                      n142 = property on="FullSpeed1 Speed" class="DigNum (strict)"() -> ("Value"=w337:dbl)  [unwired: 2 in, 2 out]
                      n143 = Subtract(x=w336, y=w335) -> (x-y=w334:dbl)
                      n144 = Absolute Value(x=w334) -> (abs(x)=w323:dbl)
                      n145 = Greater Or Equal?(x=w323, y=u32 5) -> (x >= y?=w329:bool)
                      n146 = Equal?(x=w318, y=u8 95) -> (x = y?=w321:bool)
                      n147 = case shown="False" w321 {
                        tunnel: w338 -> [_ w351]
                        tunnel: w337 -> [_ w350]
                        tunnel: [TRUE w347] -> w330
                        frame False {
                        }
                        frame True {
                          n148 = Subtract(x=w351, y=w350) -> (x-y=w352:dbl)
                          n149 = Absolute Value(x=w352) -> (abs(x)=w349:dbl)
                          n150 = Greater Or Equal?(x=w349, y=500.0) -> (x >= y?=w347:bool)
                        }
                      }
                      n151 = call "Find_Number_LineMARVIN.vi"("Test Paragraph"="7.5.2.4", "TableIn"=w331) -> ("Line number"=w328:i32)  [unwired: 3 in, 3 out]
                      n152 = And(x=w330, y=w329) -> (x .and. y?=w320:bool)
                      "VenableDirectionResult" <- w320
                      n153 = call "PassOrFail (SubVI).vi"("String Res"="", "index (row)"=w328, "Data in"=-3.0, "Pass?Fail"=w320, "Table in"=w331) -> ("error out"=w326:errorcluster)  [unwired: 6 in]
                      n154 = property on="Test Failed" class="Bool (strict)"() -> ("Value"=w319:bool)  [unwired: 2 in, 2 out]
                      n155 = case shown="False" w319 {
                        tunnel: w320 -> [w345 _]
                        frame False {
                          n156 = Not(x=w345) -> (.not. x?=w344:bool)
                          n157 = property on="Test Failed" class="Bool (strict)"("Value"=w344) -> ()  [unwired: 2 in, 2 out]
                        }
                        frame True {
                        }
                      }
                      n158 = property class="Bool (strict)"(reference=w327, error in=w326) -> ("Value"=w343:bool)  [unwired: 2 out]
                      n159 = Select(t=T12."Stop", s=w343, f=T12."Stop") -> (s? t:f=w340:T12)
                    }
                    frame "FullSpeed2" {
                      n160 = Concatenate Strings(w368, "\nFull speed operation " ("string")) -> (w354:string)
                      n161 = Equal?(x=w353, y=u8 95) -> (x = y?=w363:bool)
                      n162 = Select(t=u16 15100, s=w363, f=u16 12100 ("y")) -> (s? t:f=w377:u16)
                      n163 = call "CANSendMotorSpeed.vi"("Remote"=TRUE, "Motor Speed RPM"=w377, "UUT"=w378, "CAN Cluster in"=w382) -> ("error out"=w375:errorcluster)  [unwired: 7 in]
                      n164 = call "Write panel message (SubVI).vi"("Stop BurnIn"=w355, 4:"rpm"=w373, 5:"rpm"=TRUE ("rpm"), "PrintTime"=FALSE, "Stop"=w357, "error in (no error)"=w375, "Time to wait"=0.2, "Strin"=w354, "String in"=w356) -> ("error out"=w360:errorcluster)  [unwired: 2 in]
                      n165 = flat-sequence {
                        tunnel: w360 -> [w389]
                        tunnel: [w389] -> w359
                        tunnel: [w388] -> w358
                        frame #0 {
                          n166 = call <vilib>:"High Resolution Relative Seconds.vi"() -> ("relative seconds"=w388:dbl)
                        }
                      }
                      n167 = Select(t=15000.0, s=w363, f=11500.0) -> (s? t:f=w362:dbl)
                      n168 = Select(t=50.0, s=w363, f=24.0) -> (s? t:f=w361:dbl)
                      n169 = while {
                        tunnel: w373 -> [w391]
                        tunnel: w359 -> [w419]
                        tunnel: [w399] -> w370
                        tunnel: w362 -> [w412]
                        tunnel: w361 -> [w411]
                        tunnel: w358 -> [w407]
                        tunnel: w357 -> [w397]
                        tunnel: w356 -> [w398]
                        tunnel: w355 -> [w395]
                        tunnel: w354 -> [w394]
                        stop <- w409 stop-if-true
                        n170 = call <vilib>:"High Resolution Relative Seconds.vi"() -> ("relative seconds"=w408:dbl)
                        n171 = Subtract(x=w408, y=w407) -> (x-y=w406:dbl)
                        n172 = property class="DigNum (strict)"(reference=w391, error in=w419) -> (error out=w418:errorcluster, "Value"=w413:dbl)  [unwired: 1 out]
                        "FullSpeed2 Speed" <- w413
                        n173 = Greater Or Equal?(x=w406, y=120.0) -> (x >= y?=w404:bool)
                        n174 = Greater Or Equal?(x=w413, y=w412) -> (x >= y?=w403:bool)
                        n175 = property on="VISA Tester" class="VISAName"(error in=w418) -> (error out=w417:errorcluster, "Value"=w416:refnum<visa-resource-name>)  [unwired: 1 in, 1 out]
                        n176 = property class="Bool (strict)"(reference=w397) -> ("Value"=w402:bool)  [unwired: 1 in, 2 out]
                        n177 = call "GetADCTester (SubVI).vi"("error in (no error)"=w417, "GetADCTester"=T13."Current", "TimeToGet"=5, "VISA Refnum in"=w416) -> ("error out"=w414:errorcluster, "ADCValOutput Single"=w410:dbl)  [unwired: 5 in, 1 out]
                        "FullSpeed2 Current" <- w410
                        n178 = Greater Or Equal?(x=w410, y=w411) -> (x >= y?=w400:bool)
                        n179 = And(x=w403, y=w400) -> (x .and. y?=w401:bool)
                        n180 = Compound Arithmetic op=OR(w402, w404, w401) -> (w409:bool)
                        n181 = call "Write panel message (SubVI).vi"("Stop BurnIn"=w395, 4:"rpm"=w391, 5:"rpm"=TRUE ("rpm"), "PrintTime"=FALSE, "Stop"=w397, "error in (no error)"=w414, "Time to wait"=0.2, "Strin"=w394, "String in"=w398) -> ("error out"=w399:errorcluster)  [unwired: 2 in]
                      }
                      n182 = property class="Bool (strict)"(reference=w357, error in=w370) -> ("Value"=w387:bool)  [unwired: 2 out]
                      n183 = Select(t=T12."Stop", s=w387, f=T12."Result") -> (s? t:f=w384:T12)
                    }
                    frame "MD[1]=1" {
                      n184 = Concatenate Strings(w446, "\nSet Parameters MD[1]=1" ("Strin")) -> (w435:string)
                      n185 = property on="VISA Tester" class="VISAName"() -> ("Value"=w451:refnum<visa-resource-name>)  [unwired: 2 in, 2 out]
                      n186 = call "TesterOption (SubVI).vi"("2 Options"=FALSE, "On/Off"=FALSE, "Tester Option"=T11."Venable", "VISA Refnum in"=w451) -> ("error out"=w452:errorcluster, "VISA Refnum out"=w442:refnum<visa-resource-name>)  [unwired: 6 in]
                      n187 = call "CANSendMotorSpeed.vi"("Remote"=TRUE, "error in (no error)"=w452, "Motor Speed RPM"=u16 0, "UUT"=w436, "CAN Cluster in"=w457) -> ("error out"=w454:errorcluster)  [unwired: 6 in]
                      n188 = call "Write panel message (SubVI).vi"("Stop BurnIn"=w437, 4:"rpm"=w425, 5:"rpm"=TRUE ("rpm"), "PrintTime"=TRUE, "Stop"=w427, "error in (no error)"=w454, "Time to wait"=10.0, "Strin"=w435, "String in"=w438) -> ("error out"=w424:errorcluster)  [unwired: 2 in]
                      n189 = while {
                        tunnel: w425 -> [w469]
                        tunnel: w424 -> [w466]
                        tunnel: [w465] -> w423
                        stop <- w467 continue-if-true
                        n190 = property class="DigNum (strict)"(reference=w469, error in=w466) -> (error out=w465:errorcluster, "Value"=w468:dbl)  [unwired: 1 out]
                        n191 = Not Equal To 0?(x=w468) -> (x != 0?=w467:bool)
                      }
                      n192 = property on="VISA Marvin" class="VISAName"(error in=w423) -> (error out=w453:errorcluster, "Value"=w459:refnum<visa-resource-name>)  [unwired: 1 in, 1 out]
                      n193 = call "SerialMarvinSendGet.vi"("error in (no error)"=w453, "Clear Log"=FALSE, "write buffer"="EP=1\r\nMD[1]=1\r\n", "VISA resource name"=w459) -> ("error out"=w441:errorcluster)  [unwired: 6 in, 1 out]
                      n194 = call "TesterOption (SubVI).vi"("error in (no error)"=w441, "On/Off"=FALSE, "Tester Option"=T11."Power", "VISA Refnum in"=w442) -> ("error out"=w439:errorcluster, "VISA Refnum out"=w428:refnum<visa-resource-name>)  [unwired: 6 in]
                      n195 = call "Write panel message (SubVI).vi"("Stop BurnIn"=w437, 4:"rpm"=w425, 5:"rpm"=TRUE ("rpm"), "PrintTime"=TRUE, "Stop"=w427, "error in (no error)"=w439, "Time to wait"=25.0, "Strin"=w435, "String in"=w438) -> ("error out"=w429:errorcluster)  [unwired: 2 in]
                      n196 = call "TesterOption (SubVI).vi"("error in (no error)"=w429, "On/Off"=TRUE, "Tester Option"=T11."Venable", "VISA Refnum in"=w428) -> ("error out"=w426:errorcluster)  [unwired: 6 in, 1 out]
                      n197 = call "Time Delay8"("error in (no error)"=w426) -> ("error out"=w421:errorcluster)  [unwired: 10 in]
                      n198 = property class="Bool (strict)"(reference=w427, error in=w421) -> ("Value"=w464:bool)  [unwired: 2 out]
                      n199 = Select(t=T12."Stop", s=w464, f=T12."FullSpeed2") -> (s? t:f=w463:T12)
                    }
                    frame "FullSpeed1" {
                      n200 = Concatenate Strings(w489, "\nFull speed operation " ("string")) -> (w474:string)
                      n201 = Equal?(x=w470, y=u8 95) -> (x = y?=w487:bool)
                      n202 = flat-sequence {
                        tunnel: w480 -> [w506]
                        tunnel: [w506] -> w479
                        tunnel: [w505] -> w478
                        frame #0 {
                          n203 = call <vilib>:"High Resolution Relative Seconds.vi"() -> ("relative seconds"=w505:dbl)
                        }
                      }
                      n204 = Select(t=u16 15100, s=w487, f=u16 12100 ("y")) -> (s? t:f=w494:u16)
                      n205 = call "CANSendMotorSpeed.vi"("Remote"=TRUE, "Motor Speed RPM"=w494, "UUT"=w495, "CAN Cluster in"=w499) -> ("error out"=w492:errorcluster)  [unwired: 7 in]
                      n206 = call "Write panel message (SubVI).vi"("Stop BurnIn"=w475, 4:"rpm"=w491, 5:"rpm"=TRUE ("rpm"), "PrintTime"=FALSE, "Stop"=w477, "error in (no error)"=w492, "Time to wait"=0.2, "Strin"=w474, "String in"=w476) -> ("error out"=w480:errorcluster)  [unwired: 2 in]
                      n207 = Select(t=13700.0, s=w487, f=11500.0) -> (s? t:f=w482:dbl)
                      n208 = Select(t=58.0, s=w487, f=33.0) -> (s? t:f=w481:dbl)
                      n209 = while {
                        tunnel: w491 -> [w508]
                        tunnel: w479 -> [w536]
                        tunnel: [w516] -> w490
                        tunnel: w482 -> [w528]
                        tunnel: w481 -> [w525]
                        tunnel: w478 -> [w523]
                        tunnel: w477 -> [w514]
                        tunnel: w476 -> [w515]
                        tunnel: w475 -> [w512]
                        tunnel: w474 -> [w511]
                        stop <- w530 stop-if-true
                        n210 = property class="DigNum (strict)"(reference=w508, error in=w536) -> (error out=w535:errorcluster, "Value"=w529:dbl)  [unwired: 1 out]
                        "FullSpeed1 Speed" <- w529
                        n211 = call <vilib>:"High Resolution Relative Seconds.vi"() -> ("relative seconds"=w524:dbl)
                        n212 = Subtract(x=w524, y=w523) -> (x-y=w522:dbl)
                        n213 = Greater Or Equal?(x=w522, y=120.0) -> (x >= y?=w520:bool)
                        n214 = Greater Or Equal?(x=w529, y=w528) -> (x >= y?=w527:bool)
                        n215 = property on="VISA Tester" class="VISAName"(error in=w535) -> (error out=w534:errorcluster, "Value"=w533:refnum<visa-resource-name>)  [unwired: 1 in, 1 out]
                        n216 = call "GetADCTester (SubVI).vi"("error in (no error)"=w534, "GetADCTester"=T13."Current", "TimeToGet"=5, "VISA Refnum in"=w533) -> ("error out"=w531:errorcluster, "ADCValOutput Single"=w526:dbl)  [unwired: 5 in, 1 out]
                        "FullSpeed1 Current" <- w526
                        n217 = Greater Or Equal?(x=w526, y=w525) -> (x >= y?=w517:bool)
                        n218 = And(x=w517, y=w527) -> (x .and. y?=w518:bool)
                        n219 = property class="Bool (strict)"(reference=w514) -> ("Value"=w519:bool)  [unwired: 1 in, 2 out]
                        n220 = call "Write panel message (SubVI).vi"("Stop BurnIn"=w512, 4:"rpm"=w508, 5:"rpm"=TRUE ("rpm"), "PrintTime"=FALSE, "Stop"=w514, "error in (no error)"=w531, "Time to wait"=0.2, "Strin"=w511, "String in"=w515) -> ("error out"=w516:errorcluster)  [unwired: 2 in]
                        n221 = Compound Arithmetic op=OR(w519, w518, w520) -> (w530:bool)
                      }
                      n222 = property class="Bool (strict)"(reference=w477, error in=w490) -> ("Value"=w504:bool)  [unwired: 2 out]
                      n223 = Select(t=T12."Stop", s=w504, f=T12."MD[1]=1") -> (s? t:f=w501:T12)
                    }
                    frame "MD[1]=0" {
                      n224 = Concatenate Strings(w563, "\nSet Parameters MD[1]=0" ("Strin")) -> (w552:string)
                      n225 = property on="VISA Tester" class="VISAName"() -> ("Value"=w569:refnum<visa-resource-name>)  [unwired: 2 in, 2 out]
                      n226 = call "TesterOption (SubVI).vi"("2 Options"=FALSE, "On/Off"=FALSE, "Tester Option"=T11."Venable", "VISA Refnum in"=w569) -> ("error out"=w570:errorcluster, "VISA Refnum out"=w559:refnum<visa-resource-name>)  [unwired: 6 in]
                      n227 = call "CANSendMotorSpeed.vi"("Remote"=TRUE, "error in (no error)"=w570, "Motor Speed RPM"=u16 0, "UUT"=w553, "CAN Cluster in"=w575) -> ("error out"=w572:errorcluster)  [unwired: 6 in]
                      n228 = call "Write panel message (SubVI).vi"("Stop BurnIn"=w554, 4:"rpm"=w549, 5:"rpm"=FALSE ("rpm"), "PrintTime"=FALSE, "Stop"=w543, "error in (no error)"=w572, "Time to wait"=0.2, "Strin"=w552, "String in"=w555) -> ("error out"=w566:errorcluster)  [unwired: 2 in]
                      n229 = property on="VISA Marvin" class="VISAName"(error in=w566) -> (error out=w571:errorcluster, "Value"=w577:refnum<visa-resource-name>)  [unwired: 1 in, 1 out]
                      n230 = call "SerialMarvinSendGet.vi"("error in (no error)"=w571, "Clear Log"=FALSE, "write buffer"="EP=1\r\nMD[1]=0\r\n", "VISA resource name"=w577) -> ("error out"=w558:errorcluster)  [unwired: 6 in, 1 out]
                      n231 = call "TesterOption (SubVI).vi"("2 Options"=FALSE, "error in (no error)"=w558, "On/Off"=FALSE, "Tester Option"=T11."Power", "VISA Refnum in"=w559) -> ("error out"=w556:errorcluster, "VISA Refnum out"=w544:refnum<visa-resource-name>)  [unwired: 5 in]
                      n232 = call "Write panel message (SubVI).vi"("Stop BurnIn"=w554, 4:"rpm"=w549, 5:"rpm"=FALSE ("rpm"), "PrintTime"=TRUE, "Stop"=w543, "error in (no error)"=w556, "Time to wait"=25.0, "Strin"=w552, "String in"=w555) -> ("error out"=w545:errorcluster)  [unwired: 2 in]
                      n233 = call "TesterOption (SubVI).vi"("2 Options"=FALSE, "error in (no error)"=w545, "On/Off"=TRUE, "Tester Option"=T11."Venable", "VISA Refnum in"=w544) -> ("error out"=w542:errorcluster)  [unwired: 5 in, 1 out]
                      n234 = call "Time Delay4"("error in (no error)"=w542) -> ("error out"=w538:errorcluster)  [unwired: 10 in]
                      n235 = property class="Bool (strict)"(reference=w543, error in=w538) -> ("Value"=w582:bool)  [unwired: 2 out]
                      n236 = Select(t=T12."Stop", s=w582, f=T12."FullSpeed1") -> (s? t:f=w581:T12)
                    }
                  }
                }
                n237 = flat-sequence {
                  tunnel: [enum16{"Stop", "Direction", "Venable", "Start"}."Stop"] -> w294
                  tunnel: w293 -> [_]
                  frame #0 {
                  }
                }
              }
              frame "Venable" {
                n238 = call "Find_Number_LineMARVIN.vi"("Test Paragraph"="7.5.2.1", "TableIn"=w587) -> ("Line number"=w595:i32)  [unwired: 3 in, 3 out]
                n239 = for {
                  tunnel: u16[] [5000, 0, 5000] -> [w626] mode=indexing
                  tunnel: bool[] [TRUE, FALSE, TRUE] -> [w621] mode=indexing
                  tunnel: w595 -> [w627]
                  tunnel: w594 -> [w625]
                  tunnel: w593 -> [w624]
                  tunnel: w592 -> [w612]
                  tunnel: w591 -> [w616]
                  tunnel: w589 -> [w615]
                  tunnel: w590 -> [w614]
                  tunnel: w587 -> [w608]
                  tunnel: w586 -> [w606]
                  tunnel: [w605] -> w585 mode=indexing
                  i -> [w628]
                  w630 = 200.0 ("y")
                  n240 = call "CANSendMotorSpeed.vi"("Remote"=TRUE, "Motor Speed RPM"=u16 5000, "UUT"=w624, "CAN Cluster in"=w625) -> ("error out"=w620:errorcluster)  [unwired: 7 in]
                  n241 = property on="VISA Tester" class="VISAName"() -> ("Value"=w619:refnum<visa-resource-name>)  [unwired: 2 in, 2 out]
                  n242 = Add(x=w627, y=w628) -> (x+y=w609:i32)
                  n243 = call "TesterOption (SubVI).vi"("error in (no error)"=w620, "On/Off"=w621, "Tester Option"=T11."Venable", "VISA Refnum in"=w619) -> ("error out"=w618:errorcluster)  [unwired: 6 in, 1 out]
                  n244 = call "Write panel message (SubVI).vi"("Stop BurnIn"=w614, 4:"rpm"=w612, 5:"rpm"=TRUE ("rpm"), "PrintTime"=TRUE, "Stop"=w615, "error in (no error)"=w618, "Time to wait"=15.0, "Strin"=w606, "String in"=w616) -> ("error out"=w617:errorcluster)  [unwired: 2 in]
                  n245 = property class="DigNum (strict)"(reference=w612, error in=w617) -> ("Value"=w607:dbl)  [unwired: 2 out]
                  n246 = Add(x=w626, y=w630) -> (x+y=w632:dbl)
                  n247 = Subtract(x=w626, y=w630) -> (x-y=w631:dbl)
                  n248 = In Range and Coerce(upper limit=w632, x=w607, lower limit=w631) -> (In Range?=w605:bool)  [unwired: 1 out]
                  n249 = call "PassOrFail (SubVI).vi"("index (row)"=w609, "Data in"=w607, "Pass?Fail"=w605, "Table in"=w608) -> ()  [unwired: 7 in, 1 out]
                }
                n250 = property class="Bool (strict)"(reference=w589) -> ("Value"=w602:bool)  [unwired: 1 in, 2 out]
                n251 = property on="Test Failed" class="Bool (strict)"() -> ("Value"=w583:bool)  [unwired: 2 in, 2 out]
                n252 = And Array Elements(Boolean array=w585) -> (logical AND=w584:bool)
                "VenableResult" <- w584
                n253 = case shown="False" w583 {
                  tunnel: w584 -> [w604 _]
                  frame False {
                    n254 = Not(x=w604) -> (.not. x?=w603:bool)
                    n255 = property on="Test Failed" class="Bool (strict)"("Value"=w603) -> ()  [unwired: 2 in, 2 out]
                  }
                  frame True {
                  }
                }
                n256 = Select(t=enum16{"Stop", "Direction", "Venable", "Start"}."Stop", s=w602, f=enum16{"Stop", "Direction", "Venable", "Start"}."Direction") -> (s? t:f=w588:enum16{"Stop", "Direction", "Venable", "Start"})
              }
              frame "Start" {
                w651 = "7.5.2" ("Test Paragraph")
                n257 = property class="Str"(reference=w642, "Value"=w633) -> (reference out=w652:refnum<vi>, error out=w639:errorcluster)  [unwired: 1 in]
                n258 = call "Table_ScrollaBarMarvin.vi"("error in"=w639, "Line to focus"=w651, "reference in"=w643) -> ("error out"=w648:errorcluster)  [unwired: 2 out]
                n259 = call "Reset old test Values (SubVI).vi"("error in"=w648, "Atr in"=w643, "Test Paragraph"=w651) -> ("error out"=w647:errorcluster)  [unwired: 8 in]
                n260 = property on="VISA Tester" class="VISAName"(error in=w647) -> (error out=w646:errorcluster, "Value"=w645:refnum<visa-resource-name>)  [unwired: 1 in, 1 out]
                n261 = property class="Bool (strict)"(reference=w636) -> ("Value"=w656:bool)  [unwired: 1 in, 2 out]
                n262 = call "TesterOption (SubVI).vi"("error in (no error)"=w646, "On/Off"=TRUE, "Tester Option"=T11."Venable", "VISA Refnum in"=w645) -> ("error out"=w644:errorcluster)  [unwired: 6 in, 1 out]
                n263 = Select(t=enum16{"Stop", "Direction", "Venable", "Start"}."Stop", s=w656, f=enum16{"Stop", "Direction", "Venable", "Start"}."Venable") -> (s? t:f=w640:enum16{"Stop", "Direction", "Venable", "Start"})
                n264 = call "Write panel message (SubVI).vi"("Stop BurnIn"=w635, 4:"rpm"=w634, 5:"rpm"=FALSE ("rpm"), "PrintTime"=FALSE, "Stop"=w636, "error in (no error)"=w644, "Time to wait"=0.2, "Strin"=w633, "String in"=w652) -> ()  [unwired: 2 in, 1 out]
              }
            }
          }
        }
        frame "Speed Command" {
          w661 = "7.5.4 Speed Command Test in process..." ("Value")
          w658 = "7.5.4" ("Test Paragraph")
          n265 = control-ref of="Pannel User Message"() -> (w673:refnum<vi>)
          n266 = property class="Str"(reference=w673, error in=w672, "Value"=w661) -> (error out=w671:errorcluster)  [unwired: 1 out]
          n267 = call "Table_ScrollaBarMarvin.vi"("error in"=w671, "Line to focus"=w658, "reference in"=w657) -> ("error out"=w674:errorcluster)  [unwired: 2 out]
          n268 = property class="Tbl (strict)"(reference=w657, error in=w674) -> (error out=w676:errorcluster, "Value"=w677:string[][])  [unwired: 1 out]
          n269 = Index Array(array=w677, index (col)=0 ("disabled index (col)")) -> (element=w678:string[])  [unwired: 1 in]
          n270 = call "Find_Number_Line.vi"("error in"=w676, "Test Paragraph"=w658, "Row Headers[]"=w678) -> ("error out"=w659:errorcluster, "Line number"=w662:i32)  [unwired: 1 out]
          n271 = call "Reset old test Values (SubVI).vi"("error in"=w659, "Atr in"=w657, "Test Paragraph"=w658) -> ()  [unwired: 8 in, 1 out]
          n272 = control-ref of="Pannel User Message"() -> (w666:refnum<vi>)
          n273 = control-ref of="Stop Burn-in"() -> (w670:refnum<vi>)
          n274 = control-ref of="Config_CANAT"() -> (w667:refnum<vi>)
          n275 = control-ref of="Motor Speed RPM"() -> (w668:refnum<vi>)
          n276 = control-ref of="UUT"() -> (w669:refnum<vi>)
          n277 = control-ref of="Stop Button"() -> (w664:refnum<vi>)
          n278 = control-ref of="ATR"() -> (w665:refnum<vi>)
          n279 = property on="UUT" class="DigNum (strict)"() -> ("Value"=w660:u8)  [unwired: 2 in, 2 out]
          n280 = while {
            shift-right: [w690] -> _
            shift-left: enum16{"Stop", "StopTime", "Speeds", "Start"}."Start" -> [w691]
            tunnel: w664 -> [w689]
            tunnel: w665 -> [w688]
            tunnel: w666 -> [w687]
            tunnel: w667 -> [w686]
            tunnel: w668 -> [w685]
            tunnel: w669 -> [w684]
            tunnel: w670 -> [w683]
            tunnel: w662 -> [w682]
            tunnel: w661 -> [w681]
            tunnel: w660 -> [w679]
            stop <- w680 stop-if-true
            n281 = case shown="\"StopTime\"" w691 {
              tunnel: [w695 w725 w769 w815] -> w690
              tunnel: w689 -> [_ w720 w773 w813]
              tunnel: w688 -> [_ w710 w777 _]
              tunnel: w687 -> [_ w721 w774 _]
              tunnel: w686 -> [w693 w723 w776 _]
              tunnel: w685 -> [_ w718 w771 _]
              tunnel: w684 -> [w694 w722 w768 _]
              tunnel: w683 -> [_ w719 w772 _]
              tunnel: w682 -> [_ _ w778 _]
              tunnel: w681 -> [_ _ w775 _]
              tunnel: [w692 w724 w770 FALSE ("Value")] -> w680
              tunnel: w679 -> [_ _ w761 _]
              frame "Stop", Default {
                n282 = flat-sequence {
                  tunnel: w694 -> [w698]
                  tunnel: w693 -> [w697]
                  tunnel: [enum16{"Stop", "StopTime", "Speeds", "Start"}."Stop"] -> w695
                  tunnel: [TRUE] -> w692
                  frame #0 {
                    n283 = call "CANSendMotorSpeed.vi"("Remote"=TRUE, "Motor Speed RPM"=u16 0, "UUT"=w698, "CAN Cluster in"=w697) -> ("error out"=w703:errorcluster)  [unwired: 7 in]
                    n284 = property on="VISA Tester" class="VISAName"() -> ("Value"=w704:refnum<visa-resource-name>)  [unwired: 2 in, 2 out]
                    n285 = call "TesterOption (SubVI).vi"("2 Options"=FALSE, "error in (no error)"=w703, "On/Off"=FALSE, "Tester Option"=T11."Power", "VISA Refnum in"=w704) -> ()  [unwired: 5 in, 2 out]
                  }
                  frame #1 {
                  }
                }
              }
              frame "StopTime" {
                n286 = call "Table_ScrollaBarMarvin.vi"("Line to focus"="7.5.3", "reference in"=w710) -> ("error out"=w711:errorcluster)  [unwired: 1 in, 2 out]
                n287 = call "CANSendMotorSpeed.vi"("Remote"=TRUE, "error in (no error)"=w711, "Motor Speed RPM"=u16 0, "UUT"=w722, "CAN Cluster in"=w723) -> ("error out"=w729:errorcluster)  [unwired: 6 in]
                n288 = flat-sequence {
                  tunnel: [w757] -> w728
                  tunnel: w729 -> [w756]
                  tunnel: [w756] -> w730
                  frame #0 {
                    n289 = call <vilib>:"High Resolution Relative Seconds.vi"() -> ("relative seconds"=w757:dbl)
                  }
                }
                n290 = while {
                  tunnel: [w752] -> w724
                  tunnel: w721 -> [w750]
                  tunnel: w720 -> [w749]
                  tunnel: w719 -> [w747]
                  tunnel: w718 -> [w746]
                  tunnel: "7.5.3 Stop Time Test in process...\n" ("Value") -> [w734]
                  tunnel: [w742] -> w708
                  tunnel: w730 -> [w754]
                  tunnel: [w743] -> w716
                  tunnel: w728 -> [w753]
                  tunnel: [w741] -> w712
                  stop <- w733 stop-if-true
                  n291 = call "Write panel message (SubVI).vi"("Stop BurnIn"=w747, 4:"rpm"=w746, 5:"rpm"=TRUE ("rpm"), "PrintTime"=FALSE, "Stop"=w749, "error in (no error)"=w754, "Time to wait"=0.1, "Strin"=w734, "String in"=w750) -> ("error out"=w751:errorcluster)  [unwired: 2 in]
                  n292 = control-ref of="Motor Speed RPM"() -> (w740:refnum<vi>)
                  n293 = property class="DigNum (strict)"(reference=w740, error in=w751) -> (error out=w743:errorcluster, "Value"=w739:dbl)  [unwired: 1 out]
                  n294 = call <vilib>:"High Resolution Relative Seconds.vi"() -> ("relative seconds"=w737:dbl)
                  n295 = property class="Bool (strict)"(reference=w749) -> ("Value"=w752:bool)  [unwired: 1 in, 2 out]
                  n296 = Subtract(x=w737, y=w753) -> (x-y=w741:dbl)
                  n297 = Greater Or Equal?(x=w741, y=50.0) -> (x >= y?=w735:bool)
                  n298 = Less Or Equal?(x=w739, y=0.0) -> (x <= y?=w742:bool)
                  n299 = Compound Arithmetic op=OR(w742, w735, w752) -> (w733:bool)
                }
                "StopTimeResult" <- w708
                n300 = call "Find_Number_LineMARVIN.vi"("Test Paragraph"="7.5.3.1", "TableIn"=w710) -> ("Line number"=w713:i32)  [unwired: 3 in, 3 out]
                n301 = property on="Test Failed" class="Bool (strict)"() -> ("Value"=w707:bool)  [unwired: 2 in, 2 out]
                n302 = call "PassOrFail (SubVI).vi"("index (row)"=w713, "error in (no error)"=w716, "Data in"=w712, "Pass?Fail"=w708, "Table in"=w710) -> ("error out"=w715:errorcluster)  [unwired: 6 in]
                n303 = flat-sequence {
                  tunnel: [enum16{"Stop", "StopTime", "Speeds", "Start"}."Stop"] -> w725
                  tunnel: w715 -> [_]
                  frame #0 {
                  }
                }
                n304 = case shown="False" w707 {
                  tunnel: w708 -> [w732 _]
                  frame False {
                    n305 = Not(x=w732) -> (.not. x?=w731:bool)
                    n306 = property on="Test Failed" class="Bool (strict)"("Value"=w731) -> ()  [unwired: 2 in, 2 out]
                  }
                  frame True {
                  }
                }
              }
              frame "Speeds" {
                n307 = Equal?(x=w761, y=u8 95) -> (x = y?=w766:bool)
                n308 = Select(t=u16[] [6000, 11500, 15100], s=w766, f=u16[] [6000, 9000, 12100]) -> (s? t:f=w763:u16[])
                n309 = for {
                  tunnel: w763 -> [w806] mode=indexing
                  tunnel: w778 -> [w799]
                  tunnel: w777 -> [w798]
                  tunnel: w768 -> [w797]
                  tunnel: w776 -> [w796]
                  tunnel: w775 -> [w795]
                  tunnel: w774 -> [w794]
                  tunnel: w773 -> [w793]
                  tunnel: w772 -> [w791]
                  tunnel: w771 -> [w789]
                  tunnel: [w787] -> w770
                  tunnel: [w786] -> w762
                  tunnel: [w785] -> w760 mode=indexing
                  i -> [w805]
                  stop <- w787 stop-if-true
                  w807 = 200.0 ("y")
                  n310 = Increment(x=w805) -> (x+1=w804:i32)
                  n311 = Add(x=w799, y=w804) -> (x+y=w800:i32)
                  n312 = call "CANSendMotorSpeed.vi"("Remote"=TRUE, "Motor Speed RPM"=w806, "UUT"=w797, "CAN Cluster in"=w796) -> ("error out"=w811:errorcluster)  [unwired: 7 in]
                  n313 = control-ref of="Motor Speed RPM"() -> (w812:refnum<vi>)
                  n314 = call "Write panel message (SubVI).vi"("Stop BurnIn"=w791, 4:"rpm"=w789, 5:"rpm"=TRUE ("rpm"), "PrintTime"=TRUE, "Stop"=w793, "error in (no error)"=w811, "Time to wait"=25.0 ("Delay Time (sec)"), "Strin"=w795, "String in"=w794) -> ("error out"=w803:errorcluster)  [unwired: 2 in]
                  n315 = property class="DigNum (strict)"(reference=w812, error in=w803) -> (error out=w810:errorcluster, "Value"=w788:dbl)  [unwired: 1 out]
                  n316 = property class="Bool (strict)"(reference=w793) -> ("Value"=w787:bool)  [unwired: 1 in, 2 out]
                  n317 = Add(x=w806, y=w807) -> (x+y=w809:dbl)
                  n318 = Subtract(x=w806, y=w807) -> (x-y=w808:dbl)
                  n319 = In Range and Coerce(upper limit=w809, x=w788, lower limit=w808) -> (In Range?=w785:bool)  [unwired: 1 out]
                  n320 = call "PassOrFail (SubVI).vi"("index (row)"=w800, "error in (no error)"=w810, "Data in"=w788, "Pass?Fail"=w785, "Table in"=w798) -> ("error out"=w786:errorcluster)  [unwired: 6 in]
                }
                n321 = flat-sequence {
                  tunnel: w770 -> [w784]
                  tunnel: [w782] -> w769
                  tunnel: w762 -> [_]
                  frame #0 {
                    n322 = Select(t=enum16{"Stop", "StopTime", "Speeds", "Start"}."Stop", s=w784, f=enum16{"Stop", "StopTime", "Speeds", "Start"}."StopTime") -> (s? t:f=w782:enum16{"Stop", "StopTime", "Speeds", "Start"})
                  }
                }
                n323 = property on="Test Failed" class="Bool (strict)"() -> ("Value"=w758:bool)  [unwired: 2 in, 2 out]
                n324 = And Array Elements(Boolean array=w760) -> (logical AND=w759:bool)
                "SpeedResult" <- w759
                n325 = case shown="False" w758 {
                  tunnel: w759 -> [w780 _]
                  frame False {
                    n326 = Not(x=w780) -> (.not. x?=w779:bool)
                    n327 = property on="Test Failed" class="Bool (strict)"("Value"=w779) -> ()  [unwired: 2 in, 2 out]
                  }
                  frame True {
                  }
                }
              }
              frame "Start" {
                n328 = property on="VISA Tester" class="VISAName"() -> ("Value"=w823:refnum<visa-resource-name>)  [unwired: 2 in, 2 out]
                n329 = call "TesterOption (SubVI).vi"("2 Options"=FALSE, "On/Off"=TRUE, "Tester Option"=T11."Venable", "VISA Refnum in"=w823) -> ("error out"=w814:errorcluster)  [unwired: 6 in, 1 out]
                n330 = property class="Bool (strict)"(reference=w813, error in=w814) -> ("Value"=w819:bool)  [unwired: 2 out]
                n331 = Select(t=enum16{"Stop", "StopTime", "Speeds", "Start"}."Stop", s=w819, f=enum16{"Stop", "StopTime", "Speeds", "Start"}."Speeds") -> (s? t:f=w815:enum16{"Stop", "StopTime", "Speeds", "Start"})
              }
            }
          }
        }
        frame "Stop Time" {
          w827 = "9. Motor Temperature test in process..." ("Value")
          w825 = "9" ("Test Paragraph")
          n332 = control-ref of="Pannel User Message"() -> (w835:refnum<vi>)
          n333 = property class="Str"(reference=w835, error in=w834, "Value"=w827) -> (error out=w833:errorcluster)  [unwired: 1 out]
          n334 = call "Table_ScrollaBarMarvin.vi"("error in"=w833, "Line to focus"=w825, "reference in"=w824) -> ("error out"=w837:errorcluster)  [unwired: 2 out]
          n335 = property class="Tbl (strict)"(reference=w824, error in=w837) -> (reference out=w830:refnum<vi>, error out=w839:errorcluster, "Value"=w840:string[][])
          n336 = Index Array(array=w840, index (col)=0 ("disabled index (col)")) -> (element=w841:string[])  [unwired: 1 in]
          n337 = call "Find_Number_LineMARVIN.vi"("Test Paragraph"=w825, "error in"=w839, "TableIn"=w824, "Row Headers[]"=w841) -> ("error out"=w836:errorcluster, "Line number"=w829:i32)  [unwired: 1 in, 2 out]
          n338 = call "Reset old test Values (SubVI).vi"("error in"=w836, "Atr in"=w824, "Test Paragraph"=w825) -> ("error out"=w826:errorcluster)  [unwired: 8 in]
          n339 = property on="Status" class="Bool (strict)"(error in=w826) -> (error out=w831:errorcluster, "Value"=w832:bool)  [unwired: 1 in, 1 out]
          n340 = case shown="True" w832 {
            selector: w832 -> [w845 _]
            tunnel: w831 -> [w847 _]
            tunnel: w830 -> [w844 _]
            tunnel: w829 -> [w843 w850]
            tunnel: w828 -> [_ w855]
            tunnel: w827 -> [_ w851]
            frame False {
              n341 = flat-sequence {
                tunnel: w847 -> [w848]
                tunnel: [w848] -> w846
                frame #0 {
                  n342 = One Button Dialog(message="Please establish RS connection.") -> ()  [unwired: 1 in, 1 out]
                }
              }
              n343 = Increment(x=w843) -> (x+1=w842:i32)
              n344 = call "PassOrFail (SubVI).vi"("index (row)"=w842, "error in (no error)"=w846, "Pass?Fail"=w845, "Table in"=w844) -> ()  [unwired: 7 in, 1 out]
            }
            frame True {
              n345 = control-ref of="Stop Burn-in"() -> (w857:refnum<vi>)
              n346 = control-ref of="Pannel User Message"() -> (w859:refnum<vi>)
              n347 = control-ref of="Config_CANAT"() -> (w853:refnum<vi>)
              n348 = control-ref of="ATR"() -> (w860:refnum<vi>)
              n349 = control-ref of="Motor Speed RPM"() -> (w861:refnum<vi>)
              n350 = control-ref of="UUT"() -> (w852:refnum<vi>)
              n351 = control-ref of="Stop Button"() -> (w858:refnum<vi>)
              n352 = property on="VISA Tester" class="VISAName"() -> ("Value"=w854:refnum<visa-resource-name>)  [unwired: 2 in, 2 out]
              n353 = while {
                shift-right: [w865] -> _
                shift-left: T14."Start" -> [w875]
                tunnel: w857 -> [w874]
                tunnel: w858 -> [w873]
                tunnel: w859 -> [w872]
                tunnel: w860 -> [w871]
                tunnel: w861 -> [w870]
                tunnel: w855 -> [w869]
                tunnel: w854 -> [w868]
                tunnel: w853 -> [w867]
                tunnel: w852 -> [w866]
                tunnel: w851 -> [w863]
                tunnel: w850 -> [w862]
                stop <- w864 stop-if-true
                n354 = case shown="\"TA[5]\"" w875 {
                  tunnel: w874 -> [_ w899 w960]
                  tunnel: w873 -> [_ w891 w962]
                  tunnel: w872 -> [_ w900 w964]
                  tunnel: w871 -> [_ w889 _]
                  tunnel: w870 -> [_ w898 w959]
                  tunnel: w869 -> [_ w903 _]
                  tunnel: w868 -> [w878 w902 w953]
                  tunnel: w867 -> [_ _ w970]
                  tunnel: w866 -> [_ _ w969]
                  tunnel: [w876 w892 w955] -> w865
                  tunnel: [w877 FALSE FALSE] -> w864
                  tunnel: w863 -> [_ w901 _]
                  tunnel: w862 -> [_ w888 _]
                  frame "Stop", Default {
                    n355 = flat-sequence {
                      tunnel: w878 -> [w879]
                      tunnel: [TRUE] -> w877
                      tunnel: [T14."Stop"] -> w876
                      frame #0 {
                        n356 = call "TesterOption (SubVI).vi"("2 Options"=FALSE, "On/Off"=FALSE, "Tester Option"=T11."Power", "VISA Refnum in"=w879) -> ()  [unwired: 6 in, 2 out]
                      }
                      frame #1 {
                      }
                    }
                  }
                  frame "TA[5]" {
                    w904 = T17 [enum."60C", enum."90C", enum."120C"] items=["K15", "K16", "K17", "Venable", "Firmeware", "Fan", "Power", "120C", "110C", "100C", "90C", "80C", "70C", "60C", "50C", "40C", "30C", "25C", "20C", "10C", "0C"]
                    n357 = for {
                      tunnel: w904 -> [w930] mode=indexing
                      tunnel: w903 -> [w929]
                      tunnel: w902 -> [w928]
                      tunnel: w901 -> [w927]
                      tunnel: w900 -> [w926]
                      tunnel: w891 -> [w925]
                      tunnel: w899 -> [w924]
                      tunnel: w898 -> [w923]
                      tunnel: dbl[] [60.0, 90.0, 120.0] -> [w913] mode=indexing
                      tunnel: [w912] -> w890
                      tunnel: w889 -> [w919]
                      tunnel: w888 -> [w918]
                      tunnel: [w907] -> w887 mode=indexing
                      i -> [w916]
                      w911 = 3.0 ("y")
                      n358 = for {
                        N: 5 -> [_]
                        tunnel: w930 -> [w932]
                        tunnel: w929 -> [w948]
                        tunnel: w928 -> [w944]
                        tunnel: w927 -> [w942]
                        tunnel: w926 -> [w941]
                        tunnel: w925 -> [w940]
                        tunnel: w924 -> [w938]
                        tunnel: w923 -> [w935]
                        tunnel: [w934] -> w922 mode=indexing
                        tunnel: [w933] -> w920
                        n359 = call "TesterOption (SubVI).vi"("2 Options"=FALSE, "On/Off"=TRUE, "Tester Option"=w932, "VISA Refnum in"=w944) -> ("error out"=w945:errorcluster)  [unwired: 6 in, 1 out]
                        n360 = call "Write panel message (SubVI).vi"("Stop BurnIn"=w938, 4:"rpm"=w935, 5:"rpm"=FALSE ("rpm"), "PrintTime"=FALSE, "Stop"=w940, "error in (no error)"=w945, "Time to wait"=1.0, "Strin"=w942, "String in"=w941) -> ("error out"=w943:errorcluster)  [unwired: 2 in]
                        n361 = call "SerialMarvinSendGet.vi"("error in (no error)"=w943, "write buffer"="TA[2]\r\n", "VISA resource name"=w948) -> ("error out"=w933:errorcluster, "read buffer"=w946:string)  [unwired: 7 in]
                        n362 = Fract/Exp String To Number(string=w946) -> (number=w934:dbl)  [unwired: 3 in, 1 out]
                      }
                      n363 = Increment(x=w916) -> (x+1=w915:i32)
                      n364 = Add Array Elements(numeric array=w922) -> (sum=w921:dbl)
                      n365 = Add(x=w913, y=w911) -> (x+y=w910:dbl)
                      n366 = Subtract(x=w913, y=w911) -> (x-y=w909:dbl)
                      n367 = Divide(x=w921, y=5.0) -> (x/y=w908:dbl)
                      n368 = In Range and Coerce(upper limit=w910, x=w908, lower limit=w909) -> (In Range?=w907:bool)  [unwired: 1 out]
                      n369 = Add(x=w918, y=w915) -> (x+y=w917:i32)
                      n370 = call "PassOrFail (SubVI).vi"("index (row)"=w917, "error in (no error)"=w920, "Data in"=w908, "Pass?Fail"=w907, "Table in"=w919) -> ("error out"=w912:errorcluster)  [unwired: 6 in]
                    }
                    n371 = property class="Bool (strict)"(reference=w891, error in=w890) -> ("Value"=w896:bool)  [unwired: 2 out]
                    n372 = Select(t=T14."Stop", s=w896, f=T14."Stop") -> (s? t:f=w892:T14)
                    n373 = property on="Test Failed" class="Bool (strict)"() -> ("Value"=w885:bool)  [unwired: 2 in, 2 out]
                    n374 = And Array Elements(Boolean array=w887) -> (logical AND=w886:bool)
                    "MotorTempResult" <- w886
                    n375 = case shown="False" w885 {
                      tunnel: w886 -> [w905 _]
                      frame False {
                        n376 = Not(x=w905) -> (.not. x?=w906:bool)
                        n377 = property on="Test Failed" class="Bool (strict)"("Value"=w906) -> ()  [unwired: 2 in, 2 out]
                      }
                      frame True {
                      }
                    }
                  }
                  frame "Start" {
                    n378 = call "Write panel message (SubVI).vi"("Stop BurnIn"=w960, 4:"rpm"=w959, 5:"rpm"=FALSE ("rpm"), "PrintTime"=FALSE, "Stop"=w962, "Time to wait"=0.1, "Strin"="9. Motor Temperature test in process...\nInitialization state...", "String in"=w964) -> ("error out"=w965:errorcluster)  [unwired: 3 in]
                    n379 = call "TesterOption (SubVI).vi"("2 Options"=FALSE, "error in (no error)"=w965, "On/Off"=FALSE, "Tester Option"=T11."Venable", "VISA Refnum in"=w953) -> ("error out"=w967:errorcluster)  [unwired: 5 in, 1 out]
                    n380 = call "CANSendMotorSpeed.vi"("Remote"=TRUE, "error in (no error)"=w967, "Motor Speed RPM"=u16 0, "UUT"=w969, "CAN Cluster in"=w970) -> ("error out"=w952:errorcluster)  [unwired: 6 in]
                    n381 = property class="Bool (strict)"(reference=w962, error in=w952) -> ("Value"=w974:bool)  [unwired: 2 out]
                    n382 = Select(t=T14."Stop", s=w974, f=T14."TA[5]") -> (s? t:f=w955:T14)
                  }
                }
              }
            }
          }
        }
        frame "Temp Control" {
          w977 = "7.5.6 Temperature controle test in process..." ("Value")
          w975 = "7.5.6" ("Test Paragraph")
          n383 = control-ref of="Pannel User Message"() -> (w989:refnum<vi>)
          n384 = property class="Str"(reference=w989, error in=w988, "Value"=w977) -> (error out=w987:errorcluster)  [unwired: 1 out]
          n385 = control-ref of="Pannel User Message"() -> (w982:refnum<vi>)
          n386 = control-ref of="Motor Speed RPM"() -> (w980:refnum<vi>)
          n387 = control-ref of="Stop Button"() -> (w984:refnum<vi>)
          n388 = control-ref of="ATR"() -> (w983:refnum<vi>)
          n389 = control-ref of="Config_CANAT"() -> (w981:refnum<vi>)
          n390 = control-ref of="UUT"() -> (w979:refnum<vi>)
          n391 = control-ref of="Stop Burn-in"() -> (w978:refnum<vi>)
          n392 = call "Table_ScrollaBarMarvin.vi"("error in"=w987, "Line to focus"=w975, "reference in"=w990) -> ("error out"=w986:errorcluster)  [unwired: 2 out]
          n393 = call "Reset old test Values (SubVI).vi"("error in"=w986, "Atr in"=w990, "Test Paragraph"=w975) -> ("error out"=w976:errorcluster)  [unwired: 8 in]
          n394 = while {
            tunnel: w976 -> [w1002]
            shift-right: [w1000] -> _
            shift-left: enum16{"Stop", "Algorithm", "Start"}."Start" -> [w1001]
            tunnel: w984 -> [w999]
            tunnel: w983 -> [w998]
            tunnel: w982 -> [w997]
            tunnel: w981 -> [w996]
            tunnel: w980 -> [w995]
            tunnel: w979 -> [w994]
            tunnel: w978 -> [w992]
            tunnel: w977 -> [w991]
            stop <- w993 stop-if-true
            n395 = case shown="\"Algorithm\"" w1001 {
              tunnel: w1002 -> [_ _ w1123]
              tunnel: [w1003 w1023 w1112] -> w1000
              tunnel: w999 -> [_ w1034 w1116]
              tunnel: w998 -> [_ w1030 _]
              tunnel: w997 -> [_ w1035 _]
              tunnel: w996 -> [w1006 _ w1108]
              tunnel: w995 -> [_ w1031 _]
              tunnel: w994 -> [w1005 _ w1107]
              tunnel: [w1004 FALSE FALSE] -> w993
              tunnel: w992 -> [_ w1033 _]
              tunnel: w991 -> [_ w1032 _]
              frame "Stop", Default {
                n396 = flat-sequence {
                  tunnel: w1006 -> [w1011]
                  tunnel: w1005 -> [w1008]
                  tunnel: [TRUE] -> w1004
                  tunnel: [enum16{"Stop", "Algorithm", "Start"}."Stop"] -> w1003
                  frame #0 {
                    n397 = property on="VISA Tester" class="VISAName"() -> ("Value"=w1015:refnum<visa-resource-name>)  [unwired: 2 in, 2 out]
                    n398 = call "TesterOption (SubVI).vi"("2 Options"=FALSE, "On/Off"=FALSE, "Tester Option"=T11."Power", "VISA Refnum in"=w1015) -> ("error out"=w1009:errorcluster)  [unwired: 6 in, 1 out]
                    n399 = call "CANSendMotorSpeed.vi"("Remote"=TRUE, "error in (no error)"=w1009, "Motor Speed RPM"=u16 0, "UUT"=w1008, "CAN Cluster in"=w1011) -> ()  [unwired: 6 in, 1 out]
                  }
                  frame #1 {
                  }
                  frame #2 {
                  }
                }
              }
              frame "Algorithm" {
                # "Speed Goal"
                # "Speed Ind"
                # "Temp Goal"
                # "50 Deg"
                n400 = for {
                  tunnel: w1035 -> [w1064]
                  tunnel: w1034 -> [w1063]
                  tunnel: w1033 -> [w1062]
                  tunnel: w1032 -> [w1061]
                  tunnel: w1031 -> [w1060]
                  tunnel: w1030 -> [w1047]
                  tunnel: string[] ["7.5.6.1", "7.5.6.3", "7.5.6.5", "7.5.6.7", "7.5.6.9"] -> [w1045] mode=indexing
                  shift-right: [w1057] -> _
                  shift-left: 1202.0 ("Rt") -> [w1058]
                  tunnel: dbl[] [68.0, 68.0, 88.0, 80.0, 60.0] -> [w1056] mode=indexing
                  tunnel: dbl[] [6000.0, 11500.0, 15100.0, 11500.0, 6000.0] -> [w1055] mode=indexing
                  tunnel: dbl[] [6000.0, 6400.0, 11700.0, 14600.0, 11000.0] -> [w1054] mode=indexing
                  tunnel: [w1042] -> w1024
                  tunnel: [w1041] -> w1020 mode=indexing
                  tunnel: [w1040] -> w1021 mode=indexing
                  i -> [w1043]
                  stop <- w1059 stop-if-true
                  n401 = call <vilib>:"High Resolution Relative Seconds.vi"() -> ("relative seconds"=w1053:dbl)
                  n402 = while {
                    tunnel: w1064 -> [w1092]
                    tunnel: w1063 -> [w1084]
                    tunnel: w1062 -> [w1091]
                    tunnel: w1061 -> [w1070]
                    tunnel: w1060 -> [w1093]
                    shift-right: [w1089] -> w1057
                    shift-left: w1058 -> [w1088]
                    tunnel: w1043 -> [w1090]
                    tunnel: w1056 -> [w1087]
                    tunnel: w1055 -> [w1086]
                    tunnel: w1054 -> [w1085]
                    tunnel: w1053 -> [w1081]
                    tunnel: [w1076] -> w1048
                    tunnel: [w1075] -> w1040
                    tunnel: [w1074] -> w1046
                    tunnel: [w1073] -> w1041
                    tunnel: [w1072] -> w1044
                    stop <- w1082 stop-if-true
                    n403 = call "DegToDAC (SubVI).vi"("R2"=0.0, "Rt"=w1088) -> ("error out"=w1100:errorcluster, "output array"=w1101:u8[])  [unwired: 8 in]
                    n404 = call <vilib>:"High Resolution Relative Seconds.vi"() -> ("relative seconds"=w1080:dbl)
                    n405 = property on="VISA Tester" class="VISAName"() -> ("Value"=w1103:refnum<visa-resource-name>)  [unwired: 2 in, 2 out]
                    n406 = Byte Array To String(unsigned byte array=w1101) -> (string=w1102:string)
                    n407 = Subtract(x=w1081, y=w1080) -> (x-y=w1079:dbl)
                    n408 = VISA Write(VISA resource name=w1103, write buffer=w1102, error in (no error)=w1100) -> (error out=w1099:errorcluster)  [unwired: 2 out]
                    n409 = Greater Or Equal?(x=w1079, y=120.0) -> (x >= y?=w1077:bool)
                    n410 = call <vilib>:"Clear Errors.vi"("error in (no error)"=w1099) -> ("error out"=w1098:errorcluster)  [unwired: 5 in, 1 out]
                    n411 = control-ref of="Ambient Temperature"() -> (w1071:refnum<vi>)
                    n412 = property class="DigNum (strict)"(reference=w1071) -> ("Value"=w1069:dbl)  [unwired: 1 in, 2 out]
                    n413 = property class="Bool (strict)"(reference=w1084) -> ("Value"=w1083:bool)  [unwired: 1 in, 2 out]
                    n414 = Number To Fractional String(number=w1069, precision (6)=i16 2) -> (F-format string=w1066:string)  [unwired: 2 in]
                    n415 = Concatenate Strings(w1070, "\nAmbient  Temp. [C]: " ("string"), w1066) -> (w1065:string)
                    n416 = call "Write panel message (SubVI).vi"("Stop BurnIn"=w1091, 4:"rpm"=w1093, 5:"rpm"=TRUE ("rpm"), "PrintTime"=TRUE, "Stop"=w1084, "error in (no error)"=w1098, "Time to wait"=3.0, "Strin"=w1065, "String in"=w1092) -> ("error out"=w1097:errorcluster)  [unwired: 2 in]
                    n417 = call "TempAlgoTest (SubVI).vi"("Temp"=w1071, "Speed Ind"=w1085, "Motor Speed RPM"=w1093, "Round"=w1090, "Temp Up In"=w1088, "error in (no error)"=w1097, "String in"=w1092, "Temp Goal"=w1087, "Stop"=w1084, "Speed Goal"=w1086, "Stop BurnIn"=w1091, "Strin"=w1065) -> (14:"Speed Pass/Fail"=w1075:bool, "Temp  Pass/Fail"=w1074:dbl, "Temp Up Out"=w1089:dbl, 17:"Speed Pass/Fail"=w1076:dbl, "Temp Pass/Fail"=w1073:bool, "error out"=w1072:errorcluster)  [unwired: 2 in]
                    n418 = Compound Arithmetic op=OR(w1077, w1075, w1083) -> (w1082:bool)
                  }
                  n419 = property class="Bool (strict)"(reference=w1063) -> ("Value"=w1059:bool)  [unwired: 1 in, 2 out]
                  n420 = call "Find_Number_LineMARVIN.vi"("Test Paragraph"=w1045, "error in"=w1044, "TableIn"=w1047) -> ("error out"=w1049:errorcluster, "Line number"=w1052:i32)  [unwired: 2 in, 2 out]
                  n421 = Increment(x=w1052) -> (x+1=w1051:i32)
                  n422 = call "PassOrFail (SubVI).vi"("index (row)"=w1051, "error in (no error)"=w1049, "Data in"=w1046, "Pass?Fail"=w1041, "Table in"=w1047) -> ("error out"=w1050:errorcluster)  [unwired: 6 in]
                  n423 = call "PassOrFail (SubVI).vi"("index (row)"=w1052, "error in (no error)"=w1050, "Data in"=w1048, "Pass?Fail"=w1040, "Table in"=w1047) -> ("error out"=w1042:errorcluster)  [unwired: 6 in]
                }
                n424 = property on="Test Failed" class="Bool (strict)"() -> ("Value"=w1018:bool)  [unwired: 2 in, 2 out]
                n425 = Build Array (concatenate)(w1021, w1020) -> (w1022:bool[])
                n426 = flat-sequence {
                  tunnel: w1024 -> [_]
                  tunnel: [enum16{"Stop", "Algorithm", "Start"}."Stop"] -> w1023
                  frame #0 {
                  }
                }
                n427 = And Array Elements(Boolean array=w1022) -> (logical AND=w1019:bool)
                "TempControlResult" <- w1019
                n428 = case shown="False" w1018 {
                  tunnel: w1019 -> [w1037 _]
                  frame False {
                    n429 = Not(x=w1037) -> (.not. x?=w1038:bool)
                    n430 = property on="Test Failed" class="Bool (strict)"("Value"=w1038) -> ()  [unwired: 2 in, 2 out]
                  }
                  frame True {
                  }
                }
              }
              frame "Start" {
                n431 = property on="VISA Tester" class="VISAName"() -> ("Value"=w1122:refnum<visa-resource-name>)  [unwired: 2 in, 2 out]
                n432 = call "TesterOption (SubVI).vi"("On/Off 2"=TRUE, "Tester Option 2"=T11."Venable", "2 Options"=TRUE, "error in (no error)"=w1123, "On/Off"=TRUE, "Tester Option"=T11."K16", "VISA Refnum in"=w1122) -> ("error out"=w1110:errorcluster)  [unwired: 3 in, 1 out]
                n433 = call "CANSendMotorSpeed.vi"("Remote"=FALSE, "error in (no error)"=w1110, "Motor Speed RPM"=u16 0, "UUT"=w1107, "CAN Cluster in"=w1108) -> ("error out"=w1109:errorcluster)  [unwired: 6 in]
                n434 = property class="Bool (strict)"(reference=w1116, error in=w1109) -> ("Value"=w1115:bool)  [unwired: 2 out]
                n435 = Select(t=enum16{"Stop", "Algorithm", "Start"}."Stop", s=w1115, f=enum16{"Stop", "Algorithm", "Start"}."Algorithm") -> (s? t:f=w1112:enum16{"Stop", "Algorithm", "Start"})
              }
            }
          }
        }
        frame "Burn in" {
          n436 = control-ref of="Stop Button"() -> (w1127:refnum<vi>)
          n437 = control-ref of="Pannel User Message"() -> (w1130:refnum<vi>)
          n438 = control-ref of="ATR"() -> (w1126:refnum<vi>)
          n439 = control-ref of="Config_CANAT"() -> (w1129:refnum<vi>)
          n440 = control-ref of="UUT"() -> (w1128:refnum<vi>)
          n441 = control-ref of="Stop Burn-in"() -> (w1125:refnum<vi>)
          n442 = property on="UUT" class="DigNum (strict)"() -> ("Value"=w1124:u8)  [unwired: 2 in, 2 out]
          n443 = while {
            tunnel: w1130 -> [w1141]
            tunnel: w1126 -> [w1140]
            tunnel: w1129 -> [w1139]
            tunnel: w1128 -> [w1138]
            tunnel: w1127 -> [w1137]
            shift-right: [w1136] -> _
            shift-left: T15."Start" -> [w1143]
            shift-right: [w1142] -> _
            shift-left: _ -> [w1134]
            tunnel: w1125 -> [w1133]
            tunnel: w1124 -> [w1132]
            stop <- w1135 stop-if-true
            n444 = case shown="\"BurnIn\"" w1143 {
              tunnel: [w1146 w1181 w1252 w1284 w1317 w1356] -> w1142
              tunnel: w1141 -> [_ w1173 _ _ _ w1355]
              tunnel: w1140 -> [_ w1176 w1225 w1271 w1303 w1342]
              tunnel: w1139 -> [_ w1172 _ _ _ w1354]
              tunnel: w1138 -> [_ w1169 _ _ _ w1333]
              tunnel: w1137 -> [_ _ w1254 w1286 w1321 w1348]
              tunnel: [w1144 T15."Stop" w1255 w1287 w1322 w1344] -> w1136
              tunnel: [w1145 FALSE FALSE FALSE FALSE FALSE] -> w1135
              tunnel: w1134 -> [w1146 w1181 w1252 w1284 w1317 _]
              tunnel: w1133 -> [_ _ _ _ _ w1338]
              tunnel: w1132 -> [_ w1161 w1216 w1263 w1295 w1332]
              frame "Stop", Default {
                n445 = flat-sequence {
                  tunnel: [TRUE] -> w1145
                  tunnel: [T15."Stop"] -> w1144
                  frame #0 {
                    n446 = property on="VISA Tester" class="VISAName"() -> ("Value"=w1150:refnum<visa-resource-name>)  [unwired: 2 in, 2 out]
                    n447 = call "TesterOption (SubVI).vi"("On/Off"=FALSE, "Tester Option"=T11."Power", "VISA Refnum in"=w1150) -> ("error out"=w1147:errorcluster)  [unwired: 7 in, 1 out]
                    n448 = property on="Stop Burn-in" class="Bool (strict)"(error in=w1147, "Visible"=FALSE) -> ()  [unwired: 1 in, 2 out]
                  }
                  frame #1 {
                  }
                }
              }
              frame "BurnIn" {
                w1165 = FALSE ("Stop Burn-in")
                n449 = control-ref of="Motor Speed RPM"() -> (w1175:refnum<vi>)
                n450 = control-ref of="Stop Button"() -> (w1174:refnum<vi>)
                n451 = property on="Stop Burn-in" class="Bool (strict)"("Visible"=TRUE) -> (error out=w1177:errorcluster)  [unwired: 2 in, 1 out]
                n452 = Equal?(x=w1161, y=u8 95) -> (x = y?=w1158:bool)
                n453 = Select(t="7.5.7. " ("Test Paragraph"), s=w1158, f="7.5.6. " ("Test Paragraph")) -> (s? t:f=w1157:string)
                n454 = Select(t="7.5.7.4" ("Test Paragraph"), s=w1158, f="7.5.6.4" ("Test Paragraph")) -> (s? t:f=w1162:string)
                n455 = call "Find_Number_LineMARVIN.vi"("Test Paragraph"=w1162, "error in"=w1177, "TableIn"=w1176) -> ("error out"=w1179:errorcluster, "Line number"=w1180:i32)  [unwired: 2 in, 2 out]
                n456 = Select(t=u16 15100, s=w1158, f=u16 12100 ("y")) -> (s? t:f=w1167:u16)
                n457 = for {
                  tunnel: w1179 -> [w1203]
                  tunnel: dbl[] [600.0, 600.0, 600.0] -> [w1207] mode=indexing
                  tunnel: w1180 -> [w1212]
                  tunnel: w1176 -> [w1202]
                  tunnel: w1175 -> [w1201]
                  tunnel: w1174 -> [w1200]
                  tunnel: w1173 -> [w1199]
                  tunnel: w1172 -> [w1195]
                  tunnel: w1169 -> [w1194]
                  tunnel: w1167 -> [w1193]
                  tunnel: [w1191] -> w1166
                  tunnel: w1157 -> [w1188]
                  tunnel: [w1187] -> w1156 mode=indexing
                  i -> [w1209]
                  n458 = call "CANSendMotorSpeed.vi"("Remote"=TRUE, "error in (no error)"=w1203, "Motor Speed RPM"=w1193, "UUT"=w1194, "CAN Cluster in"=w1195) -> ("error out"=w1197:errorcluster)  [unwired: 6 in]
                  n459 = control-ref of="Stop Burn-in"() -> (w1198:refnum<vi>)
                  n460 = Concatenate Strings(w1188, "Burn-in test in process..." ("Strin")) -> (w1189:string)
                  n461 = Add(x=w1212, y=w1209) -> (x+y=w1208:i32)
                  n462 = call "Write panel message (SubVI).vi"("Stop BurnIn"=w1198, 4:"rpm"=w1201, 5:"rpm"=TRUE ("rpm"), "PrintTime"=TRUE, "Stop"=w1200, "error in (no error)"=w1197, "Time to wait"=w1207, "Strin"=w1189, "String in"=w1199) -> ("error out"=w1204:errorcluster)  [unwired: 2 in]
                  n463 = control-ref of="Power transistor Heat sink Temp."() -> (w1213:refnum<vi>)
                  n464 = property on="MaxBurnInTempVal" class="DigNum (strict)"() -> ("Value"=w1211:dbl)  [unwired: 2 in, 2 out]
                  n465 = property class="DigNum (strict)"(reference=w1213, error in=w1204) -> (error out=w1192:errorcluster, "Value"=w1210:dbl)  [unwired: 1 out]
                  n466 = Less Or Equal?(x=w1210, y=w1211) -> (x <= y?=w1187:bool)
                  n467 = call "PassOrFail (SubVI).vi"("index (row)"=w1208, "error in (no error)"=w1192, "Data in"=w1210, "Pass?Fail"=w1187, "Table in"=w1202) -> ("error out"=w1191:errorcluster)  [unwired: 6 in]
                }
                n468 = property on="Test Failed" class="Bool (strict)"() -> ("Value"=w1154:bool)  [unwired: 2 in, 2 out]
                n469 = And Array Elements(Boolean array=w1156) -> (logical AND=w1155:bool)
                "BurnResult" <- w1155
                n470 = case shown="False" w1154 {
                  tunnel: w1155 -> [w1185 _]
                  frame False {
                    n471 = Not(x=w1185) -> (.not. x?=w1186:bool)
                    n472 = property on="Test Failed" class="Bool (strict)"("Value"=w1186) -> ()  [unwired: 2 in, 2 out]
                  }
                  frame True {
                  }
                }
                n473 = property on="Stop Burn-in" class="Bool (strict)"(error in=w1166, "Value"=w1165, "Visible"=w1165) -> ()  [unwired: 1 in, 2 out]
              }
              frame "Ambient Temp" {
                w1230 = 2 ("disabled index (col)")
                n474 = control-ref of="Power transistor Heat sink Temp."() -> (w1240:refnum<vi>)
                n475 = Equal?(x=w1216, y=u8 95) -> (x = y?=w1219:bool)
                n476 = Select(t="7.5.7.3" ("Test Paragraph"), s=w1219, f="7.5.6.3" ("Test Paragraph")) -> (s? t:f=w1217:string)
                n477 = call "Find_Number_LineMARVIN.vi"("Test Paragraph"=w1217, "TableIn"=w1225) -> ("error out"=w1251:errorcluster, "Line number"=w1231:i32)  [unwired: 3 in, 2 out]
                n478 = property class="DigNum (strict)"(reference=w1240, error in=w1251) -> (error out=w1242:errorcluster, "Value"=w1232:dbl)  [unwired: 1 out]
                n479 = Select(t=25.0 ("y"), s=w1219, f=25.0 ("y")) -> (s? t:f=w1241:dbl)
                n480 = Select(t=13.0 ("y"), s=w1219, f=13.0) -> (s? t:f=w1243:dbl)
                n481 = Add(x=w1241, y=w1243) -> (x+y=w1250:dbl)
                n482 = Subtract(x=w1241, y=w1243) -> (x-y=w1249:dbl)
                n483 = In Range and Coerce(upper limit=w1250, x=w1232, lower limit=w1249) -> (In Range?=w1215:bool)  [unwired: 1 out]
                "BurnTemp" <- w1215
                n484 = call "PassOrFail (SubVI).vi"("index (row)"=w1231, "error in (no error)"=w1242, "Data in"=w1232, "Pass?Fail"=w1215, "Table in"=w1225) -> ("error out"=w1222:errorcluster)  [unwired: 6 in]
                n485 = property class="Tbl (strict)"(reference=w1225, error in=w1222) -> (reference out=w1224:refnum<vi>, error out=w1239:errorcluster, "Value"=w1238:string[][])
                n486 = Add(x=w1232, y=25.0) -> (x+y=w1223:dbl)
                "MaxBurnInTempVal" <- w1223
                n487 = Number To Fractional String(number=w1223, precision (6)=i16 0) -> (F-format string=w1237:string)  [unwired: 2 in]
                n488 = Concatenate Strings("< " ("string"), w1237) -> (w1226:string)
                n489 = Increment(x=w1231) -> (x+1=w1229:i32)
                n490 = Increment(x=w1229) -> (x+1=w1228:i32)
                n491 = Increment(x=w1228) -> (x+1=w1227:i32)
                n492 = property on="Test Failed" class="Bool (strict)"() -> ("Value"=w1214:bool)  [unwired: 2 in, 2 out]
                n493 = Replace Array Subset(array=w1238, new element #1=w1226, index (row) #1=w1229, index (col) #1=w1230, new element #2=w1226, index (row) #2=w1228, index (col) #2=w1230, new element #3=w1226, index (row) #3=w1227, index (col) #3=w1230) -> (w1236:string[][])
                n494 = case shown="False" w1214 {
                  tunnel: w1215 -> [w1259 _]
                  frame False {
                    n495 = Not(x=w1259) -> (.not. x?=w1260:bool)
                    n496 = property on="Test Failed" class="Bool (strict)"("Value"=w1260) -> ()  [unwired: 2 in, 2 out]
                  }
                  frame True {
                  }
                }
                n497 = property class="Tbl (strict)"(reference=w1224, error in=w1239, "Value"=w1236) -> (error out=w1221:errorcluster)  [unwired: 1 out]
                n498 = property class="Bool (strict)"(reference=w1254, error in=w1221) -> ("Value"=w1258:bool)  [unwired: 2 out]
                n499 = Select(t=T15."Stop", s=w1258, f=T15."BurnIn") -> (s? t:f=w1255:T15)
              }
              frame "MotorSpeed" {
                n500 = control-ref of="Motor Speed RPM"() -> (w1269:refnum<vi>)
                n501 = Equal?(x=w1263, y=u8 95) -> (x = y?=w1266:bool)
                n502 = Select(t="7.5.7.2" ("Test Paragraph"), s=w1266, f="7.5.6.2" ("Test Paragraph")) -> (s? t:f=w1264:string)
                n503 = call "Find_Number_LineMARVIN.vi"("Test Paragraph"=w1264, "TableIn"=w1271) -> ("error out"=w1283:errorcluster, "Line number"=w1274:i32)  [unwired: 3 in, 2 out]
                n504 = property class="DigNum (strict)"(reference=w1269, error in=w1283) -> (error out=w1272:errorcluster, "Value"=w1273:dbl)  [unwired: 1 out]
                n505 = Select(t=15100.0 ("y"), s=w1266, f=12100.0 ("y")) -> (s? t:f=w1270:dbl)
                n506 = Select(t=200.0 ("y"), s=w1266, f=200.0) -> (s? t:f=w1275:dbl)
                n507 = Add(x=w1270, y=w1275) -> (x+y=w1282:dbl)
                n508 = Subtract(x=w1270, y=w1275) -> (x-y=w1281:dbl)
                n509 = In Range and Coerce(upper limit=w1282, x=w1273, lower limit=w1281) -> (In Range?=w1262:bool)  [unwired: 1 out]
                "BurnSpeed" <- w1262
                n510 = call "PassOrFail (SubVI).vi"("index (row)"=w1274, "error in (no error)"=w1272, "Data in"=w1273, "Pass?Fail"=w1262, "Table in"=w1271) -> ("error out"=w1268:errorcluster)  [unwired: 6 in]
                n511 = property class="Bool (strict)"(reference=w1286, error in=w1268) -> ("Value"=w1290:bool)  [unwired: 2 out]
                n512 = property on="Test Failed" class="Bool (strict)"() -> ("Value"=w1261:bool)  [unwired: 2 in, 2 out]
                n513 = Select(t=T15."Stop", s=w1290, f=T15."Ambient Temp") -> (s? t:f=w1287:T15)
                n514 = case shown="False" w1261 {
                  tunnel: w1262 -> [w1291 _]
                  frame False {
                    n515 = Not(x=w1291) -> (.not. x?=w1292:bool)
                    n516 = property on="Test Failed" class="Bool (strict)"("Value"=w1292) -> ()  [unwired: 2 in, 2 out]
                  }
                  frame True {
                  }
                }
              }
              frame "DC Current Measure" {
                n517 = property on="VISA Tester" class="VISAName"() -> (error out=w1315:errorcluster, "Value"=w1319:refnum<visa-resource-name>)  [unwired: 2 in, 1 out]
                n518 = call "GetADCTester (SubVI).vi"("error in (no error)"=w1315, "GetADCTester"=T13."Current", "TimeToGet"=10, "VISA Refnum in"=w1319) -> ("error out"=w1316:errorcluster, "ADCValOutput Single"=w1302:dbl)  [unwired: 5 in, 1 out]
                n519 = Equal?(x=w1295, y=u8 95) -> (x = y?=w1299:bool)
                n520 = Select(t="7.5.7.1" ("Test Paragraph"), s=w1299, f="7.5.6.1" ("Test Paragraph")) -> (s? t:f=w1297:string)
                n521 = call "Find_Number_LineMARVIN.vi"("Test Paragraph"=w1297, "error in"=w1316, "TableIn"=w1303) -> ("error out"=w1314:errorcluster, "Line number"=w1304:i32)  [unwired: 2 in, 2 out]
                n522 = Select(t=50.0 ("y"), s=w1299, f=28.0 ("y")) -> (s? t:f=w1306:dbl)
                n523 = Select(t=5.0 ("y"), s=w1299, f=3.0) -> (s? t:f=w1305:dbl)
                n524 = Add(x=w1306, y=w1305) -> (x+y=w1313:dbl)
                n525 = Subtract(x=w1306, y=w1305) -> (x-y=w1312:dbl)
                n526 = In Range and Coerce(upper limit=w1313, x=w1302, lower limit=w1312) -> (In Range?=w1294:bool)  [unwired: 1 out]
                "BurnDC" <- w1294
                n527 = property on="Test Failed" class="Bool (strict)"() -> ("Value"=w1293:bool)  [unwired: 2 in, 2 out]
                n528 = call "PassOrFail (SubVI).vi"("index (row)"=w1304, "error in (no error)"=w1314, "Data in"=w1302, "Pass?Fail"=w1294, "Table in"=w1303) -> ("error out"=w1301:errorcluster)  [unwired: 6 in]
                n529 = property class="Bool (strict)"(reference=w1321, error in=w1301) -> ("Value"=w1325:bool)  [unwired: 2 out]
                n530 = Select(t=T15."Stop", s=w1325, f=T15."MotorSpeed") -> (s? t:f=w1322:T15)
                n531 = case shown="False" w1293 {
                  tunnel: w1294 -> [w1326 _]
                  frame False {
                    n532 = Not(x=w1326) -> (.not. x?=w1327:bool)
                    n533 = property on="Test Failed" class="Bool (strict)"("Value"=w1327) -> ()  [unwired: 2 in, 2 out]
                  }
                  frame True {
                  }
                }
              }
              frame "Start" {
                w1329 = " Burn-in test in process...\nFull Speed Operation" ("Value")
                n534 = Equal?(x=w1332, y=u8 95) -> (x = y?=w1334:bool)
                n535 = Select(t="7.5.7" ("Test Paragraph"), s=w1334, f="7.5.6" ("Test Paragraph")) -> (s? t:f=w1328:string)
                n536 = Concatenate Strings(w1328, w1329) -> (w1330:string)
                n537 = property class="Str"(reference=w1355, "Value"=w1330) -> (reference out=w1352:refnum<vi>, error out=w1337:errorcluster)  [unwired: 1 in]
                n538 = call "Find_Number_LineMARVIN.vi"("Test Paragraph"=w1328, "error in"=w1337, "TableIn"=w1342) -> ("error out"=w1362:errorcluster, "Line number"=w1363:i32)  [unwired: 2 in, 2 out]
                n539 = call "Table_ScrollaBarMarvin.vi"("error in"=w1362, "Line to focus"=w1328, "reference in"=w1342) -> ("error out"=w1364:errorcluster)  [unwired: 2 out]
                n540 = Select(t=u16 15100 ("y"), s=w1334, f=u16 12100 ("y")) -> (s? t:f=w1369:u16)
                n541 = call "Reset old test Values (SubVI).vi"("error in"=w1364, "Atr in"=w1342, "Test Paragraph"=w1328) -> ("error out"=w1365:errorcluster)  [unwired: 8 in]
                n542 = Increment(x=w1363) -> (x+1=w1356:i32)
                n543 = property on="VISA Tester" class="VISAName"(error in=w1365) -> (error out=w1366:errorcluster, "Value"=w1367:refnum<visa-resource-name>)  [unwired: 1 in, 1 out]
                n544 = call "TesterOption (SubVI).vi"("2 Options"=FALSE, "error in (no error)"=w1366, "On/Off"=TRUE, "Tester Option"=T11."Venable", "VISA Refnum in"=w1367) -> ("error out"=w1368:errorcluster)  [unwired: 5 in, 1 out]
                n545 = call "CANSendMotorSpeed.vi"("Remote"=TRUE, "error in (no error)"=w1368, "Motor Speed RPM"=w1369, "UUT"=w1333, "CAN Cluster in"=w1354) -> ("error out"=w1353:errorcluster)  [unwired: 6 in]
                n546 = control-ref of="Motor Speed RPM"() -> (w1341:refnum<vi>)
                n547 = call "Write panel message (SubVI).vi"("Stop BurnIn"=w1338, 4:"rpm"=w1341, 5:"rpm"=TRUE ("rpm"), "PrintTime"=TRUE, "Stop"=w1348, "error in (no error)"=w1353, "Time to wait"=50.0, "Strin"=w1329, "String in"=w1352) -> ("error out"=w1340:errorcluster)  [unwired: 2 in]
                n548 = property class="Bool (strict)"(reference=w1348, error in=w1340) -> ("Value"=w1347:bool)  [unwired: 2 out]
                n549 = Select(t=T15."Stop", s=w1347, f=T15."DC Current Measure") -> (s? t:f=w1344:T15)
              }
            }
          }
        }
        frame "Visual Inspec" {
          n550 = property on="VISA Tester" class="VISAName"() -> ("Value"=w1380:refnum<visa-resource-name>)  [unwired: 2 in, 2 out]
          n551 = call "TesterOption (SubVI).vi"("2 Options"=FALSE, "error in (no error)"=w1381, "On/Off"=FALSE, "Tester Option"=T11."Power", "VISA Refnum in"=w1380) -> ("error out"=w1376:errorcluster)  [unwired: 5 in, 1 out]
          n552 = call "VisualInspection.vi"("error in (no error)"=w1376, "TableRef"=w1382) -> ("error out"=w1372:errorcluster, "VisualInspectionResult"=w1374:bool)  [unwired: 8 in]
          "VisualInspectionResult" <- w1374
          n553 = property on="Test Failed" class="Bool (strict)"(error in=w1372) -> (error out=w1371:errorcluster, "Value"=w1373:bool)  [unwired: 1 in, 1 out]
          n554 = case shown="False" w1373 {
            tunnel: w1374 -> [w1385 _]
            tunnel: w1371 -> [w1383 w1386]
            tunnel: [w1383 w1386] -> w1370
            frame False {
              n555 = Not(x=w1385) -> (.not. x?=w1384:bool)
              n556 = property on="Test Failed" class="Bool (strict)"("Value"=w1384) -> ()  [unwired: 2 in, 2 out]
            }
            frame True {
            }
          }
          n557 = property on="Automation" class="Bool (strict)"(error in=w1370) -> ("Value"=w1375:bool)  [unwired: 1 in, 2 out]
          n558 = case shown="True" w1375 {
            frame False {
            }
            frame True {
              w1387 = TRUE ("Value (Signaling)")
              n559 = property on="SetSN" class="Bool (strict)"("Val(Sgnl)"=w1387, "Value"=w1387) -> ()  [unwired: 2 in, 2 out]
            }
          }
        }
        frame "Temp Sens Cal" {
          w1391 = "7.5.5 Temperature sensor calibration test in process..." ("Value")
          w1389 = "7.5.5" ("Test Paragraph")
          n560 = control-ref of="Pannel User Message"() -> (w1398:refnum<vi>)
          n561 = property class="Str"(reference=w1398, error in=w1397, "Value"=w1391) -> (error out=w1396:errorcluster)  [unwired: 1 out]
          n562 = call "Table_ScrollaBarMarvin.vi"("error in"=w1396, "Line to focus"=w1389, "reference in"=w1399) -> ("error out"=w1401:errorcluster)  [unwired: 2 out]
          n563 = property class="Tbl (strict)"(reference=w1399, error in=w1401) -> (reference out=w1388:refnum<vi>, error out=w1403:errorcluster, "Value"=w1404:string[][])
          n564 = Index Array(array=w1404, index (col)=0 ("disabled index (col)")) -> (element=w1405:string[])  [unwired: 1 in]
          n565 = call "Find_Number_Line.vi"("error in"=w1403, "Test Paragraph"=w1389, "Row Headers[]"=w1405) -> ("error out"=w1400:errorcluster, "Line number"=w1393:i32)  [unwired: 1 out]
          n566 = property on="Status" class="Bool (strict)"(error in=w1400) -> (error out=w1394:errorcluster, "Value"=w1395:bool)  [unwired: 1 in, 1 out]
          n567 = call "Reset old test Values (SubVI).vi"("error in"=w1394, "Atr in"=w1388, "Test Paragraph"=w1389) -> ("error out"=w1390:errorcluster)  [unwired: 8 in]
          n568 = case shown="True" w1395 {
            selector: w1395 -> [w1409 _]
            tunnel: w1390 -> [w1411 _]
            tunnel: w1388 -> [w1408 _]
            tunnel: w1393 -> [w1407 _]
            tunnel: w1392 -> [_ w1418]
            tunnel: w1391 -> [_ w1414]
            frame False {
              n569 = flat-sequence {
                tunnel: w1411 -> [w1412]
                tunnel: [w1412] -> w1410
                frame #0 {
                  n570 = One Button Dialog(message="Please establish RS connection.") -> ()  [unwired: 1 in, 1 out]
                }
              }
              n571 = Increment(x=w1407) -> (x+1=w1406:i32)
              n572 = call "PassOrFail (SubVI).vi"("index (row)"=w1406, "error in (no error)"=w1410, "Pass?Fail"=w1409, "Table in"=w1408) -> ()  [unwired: 7 in, 1 out]
            }
            frame True {
              n573 = control-ref of="Stop Burn-in"() -> (w1420:refnum<vi>)
              n574 = control-ref of="Pannel User Message"() -> (w1422:refnum<vi>)
              n575 = control-ref of="Config_CANAT"() -> (w1416:refnum<vi>)
              n576 = control-ref of="ATR"() -> (w1423:refnum<vi>)
              n577 = control-ref of="Motor Speed RPM"() -> (w1424:refnum<vi>)
              n578 = control-ref of="UUT"() -> (w1415:refnum<vi>)
              n579 = control-ref of="Stop Button"() -> (w1421:refnum<vi>)
              n580 = property on="VISA Tester" class="VISAName"() -> ("Value"=w1417:refnum<visa-resource-name>)  [unwired: 2 in, 2 out]
              n581 = while {
                shift-right: [w1427] -> _
                shift-left: T14."Start" -> [w1437]
                tunnel: w1420 -> [w1436]
                tunnel: w1421 -> [w1435]
                tunnel: w1422 -> [w1434]
                tunnel: w1423 -> [w1433]
                tunnel: w1424 -> [w1432]
                tunnel: w1418 -> [w1431]
                tunnel: w1417 -> [w1430]
                tunnel: w1416 -> [w1429]
                tunnel: w1415 -> [w1428]
                tunnel: w1414 -> [w1425]
                stop <- w1426 stop-if-true
                n582 = case shown="\"AO[1]=Meas.\"" w1437 {
                  tunnel: w1436 -> [_ w1472 w1501 w1556 w1586]
                  tunnel: w1435 -> [_ w1473 w1493 w1542 w1588]
                  tunnel: w1434 -> [_ w1470 w1502 w1554 w1590]
                  tunnel: w1433 -> [_ w1450 _ _ _]
                  tunnel: w1432 -> [_ w1474 w1500 w1557 w1585]
                  tunnel: w1431 -> [_ w1483 w1505 w1566 w1582]
                  tunnel: w1430 -> [w1440 w1479 w1504 w1562 w1570]
                  tunnel: w1429 -> [_ _ _ _ w1596]
                  tunnel: w1428 -> [_ _ _ _ w1595]
                  tunnel: [w1438 w1459 w1494 w1545 w1573] -> w1427
                  tunnel: [w1439 FALSE FALSE FALSE FALSE] -> w1426
                  tunnel: w1425 -> [_ _ w1503 _ _]
                  frame "Stop", Default {
                    n583 = flat-sequence {
                      tunnel: w1440 -> [w1441]
                      tunnel: [TRUE] -> w1439
                      tunnel: [T14."Stop"] -> w1438
                      frame #0 {
                        n584 = call "TesterOption (SubVI).vi"("2 Options"=FALSE, "On/Off"=FALSE, "Tester Option"=T11."Power", "VISA Refnum in"=w1441) -> ()  [unwired: 6 in, 2 out]
                      }
                      frame #1 {
                      }
                    }
                  }
                  frame "AO[1]=Meas." {
                    n585 = property on="AO[1]Meas" class="DigNum (strict)"() -> ("Value"=w1453:dbl)  [unwired: 2 in, 2 out]
                    n586 = Number To Fractional String(number=w1453) -> (F-format string=w1461:string)  [unwired: 3 in]
                    n587 = Search and Replace String(input string="EP=1\r\nAO[1]=0\r\n" ("write buffer"), search string="0", replace string=w1461) -> (result string=w1460:string)  [unwired: 5 in, 3 out]
                    n588 = call "SerialMarvinSendGet.vi"("Clear Log"=FALSE, "write buffer"=w1460, "VISA resource name"=w1483) -> ("error out"=w1478:errorcluster)  [unwired: 7 in, 1 out]
                    n589 = call "TesterOption (SubVI).vi"("2 Options"=FALSE, "error in (no error)"=w1478, "On/Off"=FALSE, "Tester Option"=T11."Power", "VISA Refnum in"=w1479) -> ("error out"=w1477:errorcluster, "VISA Refnum out"=w1464:refnum<visa-resource-name>)  [unwired: 5 in]
                    n590 = call "Write panel message (SubVI).vi"("Stop BurnIn"=w1472, 4:"rpm"=w1474, 5:"rpm"=FALSE ("rpm"), "PrintTime"=TRUE, "Stop"=w1473, "error in (no error)"=w1477, "Time to wait"=20.0, "Strin"="7.5.5 Temperature sensor calibration test in process...\nSet Parameters...", "String in"=w1470) -> ("error out"=w1465:errorcluster)  [unwired: 2 in]
                    n591 = call "TesterOption (SubVI).vi"("2 Options"=FALSE, "error in (no error)"=w1465, "On/Off"=FALSE, "Tester Option"=T11."Venable", "VISA Refnum in"=w1464) -> ("error out"=w1458:errorcluster)  [unwired: 5 in, 1 out]
                    n592 = flat-sequence {
                      tunnel: [T14."Stop"] -> w1459
                      tunnel: w1451 -> [_]
                      frame #0 {
                      }
                    }
                    n593 = In Range and Coerce(upper limit=0.1, x=w1453, lower limit=-0.1) -> (In Range?=w1448:bool)  [unwired: 1 out]
                    "SensCalResult" <- w1448
                    n594 = property on="Test Failed" class="Bool (strict)"() -> ("Value"=w1447:bool)  [unwired: 2 in, 2 out]
                    n595 = call "Find_Number_LineMARVIN.vi"("Test Paragraph"="7.5.5.1", "error in"=w1458, "TableIn"=w1450) -> ("error out"=w1452:errorcluster, "Line number"=w1456:i32)  [unwired: 2 in, 2 out]
                    n596 = case shown="False" w1447 {
                      tunnel: w1448 -> [w1485 _]
                      frame False {
                        n597 = Not(x=w1485) -> (.not. x?=w1486:bool)
                        n598 = property on="Test Failed" class="Bool (strict)"("Value"=w1486) -> ()  [unwired: 2 in, 2 out]
                      }
                      frame True {
                      }
                    }
                    n599 = call "PassOrFail (SubVI).vi"("index (row)"=w1456, "error in (no error)"=w1452, "Data in"=w1453, "Pass?Fail"=w1448, "Table in"=w1450) -> ("error out"=w1451:errorcluster)  [unwired: 6 in]
                  }
                  frame "TA[5]" {
                    w1506 = T17 [enum."50C", enum."80C", enum."100C", enum."120C"] items=["K15", "K16", "K17", "Venable", "Firmeware", "Fan", "Power", "120C", "110C", "100C", "90C", "80C", "70C", "60C", "50C", "40C", "30C", "25C", "20C", "10C", "0C"]
                    n600 = for {
                      tunnel: w1506 -> [w1521] mode=indexing
                      tunnel: w1505 -> [w1520]
                      tunnel: w1504 -> [w1519]
                      tunnel: w1503 -> [w1518]
                      tunnel: w1502 -> [w1517]
                      tunnel: w1493 -> [w1516]
                      tunnel: w1501 -> [w1515]
                      tunnel: w1500 -> [w1514]
                      tunnel: dbl[] [0.59774, 0.65238, 0.68545, 0.71584] -> [w1509] mode=indexing
                      tunnel: [w1508] -> w1489 mode=indexing
                      tunnel: [w1507] -> w1492
                      n601 = for {
                        N: 5 -> [_]
                        tunnel: w1521 -> [w1539]
                        tunnel: w1520 -> [w1538]
                        tunnel: w1519 -> [w1534]
                        tunnel: w1518 -> [w1532]
                        tunnel: w1517 -> [w1531]
                        tunnel: w1516 -> [w1530]
                        tunnel: w1515 -> [w1528]
                        tunnel: w1514 -> [w1525]
                        tunnel: [w1524] -> w1513 mode=indexing
                        tunnel: [w1523] -> w1507
                        n602 = call "TesterOption (SubVI).vi"("2 Options"=FALSE, "On/Off"=TRUE, "Tester Option"=w1539, "VISA Refnum in"=w1534) -> ("error out"=w1535:errorcluster)  [unwired: 6 in, 1 out]
                        n603 = call "Write panel message (SubVI).vi"("Stop BurnIn"=w1528, 4:"rpm"=w1525, 5:"rpm"=FALSE ("rpm"), "PrintTime"=FALSE, "Stop"=w1530, "error in (no error)"=w1535, "Time to wait"=1.0, "Strin"=w1532, "String in"=w1531) -> ("error out"=w1533:errorcluster)  [unwired: 2 in]
                        n604 = call "SerialMarvinSendGet.vi"("error in (no error)"=w1533, "write buffer"="TA[5]\r\n", "VISA resource name"=w1538) -> ("error out"=w1523:errorcluster, "read buffer"=w1536:string)  [unwired: 7 in]
                        n605 = Fract/Exp String To Number(string=w1536) -> (number=w1524:dbl)  [unwired: 3 in, 1 out]
                      }
                      n606 = Add Array Elements(numeric array=w1513) -> (sum=w1512:dbl)
                      n607 = Divide(x=w1512, y=5.0) -> (x/y=w1510:dbl)
                      n608 = Subtract(x=w1510, y=w1509) -> (x-y=w1508:dbl)
                    }
                    n609 = property class="Bool (strict)"(reference=w1493, error in=w1492) -> ("Value"=w1498:bool)  [unwired: 2 out]
                    n610 = Select(t=T14."Stop", s=w1498, f=T14."AO[1]=Meas.") -> (s? t:f=w1494:T14)
                    n611 = Array Size(array=w1489) -> (size(s)=w1488:i32)
                    n612 = Add Array Elements(numeric array=w1489) -> (sum=w1491:dbl)
                    n613 = Divide(x=w1491, y=w1488) -> (x/y=→"AO[1]Meas":dbl)
                  }
                  frame "AO[1]=0" {
                    n614 = call "SerialMarvinSendGet.vi"("write buffer"="EP=1\r\nAO[1]=0\r\n", "VISA resource name"=w1566) -> ("error out"=w1561:errorcluster)  [unwired: 8 in, 1 out]
                    n615 = call "TesterOption (SubVI).vi"("2 Options"=FALSE, "error in (no error)"=w1561, "On/Off"=FALSE, "Tester Option"=T11."Power", "VISA Refnum in"=w1562) -> ("error out"=w1560:errorcluster, "VISA Refnum out"=w1548:refnum<visa-resource-name>)  [unwired: 5 in]
                    n616 = call "Write panel message (SubVI).vi"("Stop BurnIn"=w1556, 4:"rpm"=w1557, 5:"rpm"=FALSE ("rpm"), "PrintTime"=TRUE, "Stop"=w1542, "error in (no error)"=w1560, "Time to wait"=20.0, "Strin"="7.5.5 Temperature sensor calibration test in process...\nSet Parameters...", "String in"=w1554) -> ("error out"=w1549:errorcluster)  [unwired: 2 in]
                    n617 = call "TesterOption (SubVI).vi"("2 Options"=FALSE, "error in (no error)"=w1549, "On/Off"=FALSE, "Tester Option"=T11."Venable", "VISA Refnum in"=w1548) -> ("error out"=w1543:errorcluster)  [unwired: 5 in, 1 out]
                    n618 = property class="Bool (strict)"(reference=w1542, error in=w1543) -> ("Value"=w1547:bool)  [unwired: 2 out]
                    n619 = Select(t=T14."Stop", s=w1547, f=T14."TA[5]") -> (s? t:f=w1545:T14)
                  }
                  frame "Start" {
                    n620 = call "Write panel message (SubVI).vi"("Stop BurnIn"=w1586, 4:"rpm"=w1585, 5:"rpm"=FALSE ("rpm"), "PrintTime"=FALSE, "Stop"=w1588, "Time to wait"=0.1, "Strin"="7.5.5 Temperature sensor calibration test in process...\nInitialization state...", "String in"=w1590) -> ("error out"=w1591:errorcluster)  [unwired: 3 in]
                    n621 = call "TesterOption (SubVI).vi"("2 Options"=FALSE, "error in (no error)"=w1591, "On/Off"=FALSE, "Tester Option"=T11."Venable", "VISA Refnum in"=w1570) -> ("error out"=w1593:errorcluster)  [unwired: 5 in, 1 out]
                    n622 = call "CANSendMotorSpeed.vi"("Remote"=TRUE, "error in (no error)"=w1593, "Motor Speed RPM"=u16 0, "UUT"=w1595, "CAN Cluster in"=w1596) -> ("error out"=w1580:errorcluster)  [unwired: 6 in]
                    n623 = call "SerialMarvinSendGet.vi"("error in (no error)"=w1580, "write buffer"="AO[1]\r\n", "VISA resource name"=w1582) -> ("error out"=w1569:errorcluster, "read buffer"=w1579:string)  [unwired: 7 in]
                    n624 = Equal?(x=w1579, y="0.0") -> (x = y?=w1571:bool)
                    n625 = property class="Bool (strict)"(reference=w1588, error in=w1569) -> ("Value"=w1600:bool)  [unwired: 2 out]
                    n626 = Select(t=T14."TA[5]", s=w1571, f=T14."AO[1]=0") -> (s? t:f=w1575:T14)
                    n627 = Select(t=T14."Stop", s=w1600, f=w1575) -> (s? t:f=w1573:T14)
                  }
                }
              }
            }
          }
        }
        frame "Auxiliary" {
          w1604 = "8. Auxiliary test in process..." ("Value")
          w1616 = "8" ("Test Paragraph")
          n628 = control-ref of="Pannel User Message"() -> (w1615:refnum<vi>)
          n629 = property class="Str"(reference=w1615, error in=w1612, "Value"=w1604) -> (error out=w1614:errorcluster)  [unwired: 1 out]
          n630 = call "Table_ScrollaBarMarvin.vi"("error in"=w1614, "Line to focus"=w1616, "reference in"=w1613) -> ("error out"=w1622:errorcluster)  [unwired: 2 out]
          n631 = property class="Tbl (strict)"(reference=w1613, error in=w1622) -> (reference out=w1611:refnum<vi>, error out=w1621:errorcluster, "Value"=w1620:string[][])
          n632 = Index Array(array=w1620, index (col)=0 ("disabled index (col)")) -> (element=w1619:string[])  [unwired: 1 in]
          n633 = call "Find_Number_Line.vi"("error in"=w1621, "Test Paragraph"=w1616, "Row Headers[]"=w1619) -> ("error out"=w1617:errorcluster, "Line number"=w1602:i32)  [unwired: 1 out]
          n634 = call "Reset old test Values (SubVI).vi"("error in"=w1617, "Atr in"=w1611, "Test Paragraph"=w1616) -> ("error out"=w1609:errorcluster)  [unwired: 8 in]
          n635 = property on="VISA Tester" class="VISAName"() -> ("Value"=w1603:refnum<visa-resource-name>)  [unwired: 2 in, 2 out]
          n636 = control-ref of="Stop Burn-in"() -> (w1606:refnum<vi>)
          n637 = control-ref of="Stop Button"() -> (w1607:refnum<vi>)
          n638 = control-ref of="Pannel User Message"() -> (w1608:refnum<vi>)
          n639 = control-ref of="ATR"() -> (w1601:refnum<vi>)
          n640 = control-ref of="Config_CANAT"() -> ()  [unwired: 1 out]
          n641 = control-ref of="Motor Speed RPM"() -> (w1605:refnum<vi>)
          n642 = while {
            shift-right: [w1627] -> _
            shift-left: enum16{"Stop", "CoolingON", "HotGunON", "Start"}."Start" -> [w1634]
            tunnel: w1609 -> [w1625]
            tunnel: w1608 -> [w1633]
            tunnel: w1607 -> [w1632]
            tunnel: w1606 -> [w1631]
            tunnel: w1605 -> [w1630]
            tunnel: w1604 -> [w1629]
            tunnel: w1603 -> [w1628]
            tunnel: w1602 -> [w1624]
            tunnel: w1601 -> [w1623]
            stop <- w1626 stop-if-true
            n643 = case shown="\"CoolingON\"" w1634 {
              tunnel: w1633 -> [_ w1681 w1763 w1825]
              tunnel: w1632 -> [_ w1673 w1755 w1811]
              tunnel: w1631 -> [_ w1680 w1762 w1824]
              tunnel: w1630 -> [_ w1679 w1761 w1820]
              tunnel: w1629 -> [_ w1666 w1748 w1819]
              tunnel: w1628 -> [_ w1667 w1749 w1812]
              tunnel: [w1636 w1669 w1751 w1807] -> w1627
              tunnel: [w1635 FALSE FALSE FALSE] -> w1626
              tunnel: w1625 -> [_ w1665 w1747 _]
              tunnel: w1624 -> [_ w1659 w1742 _]
              tunnel: w1623 -> [_ w1655 w1739 _]
              frame "Stop", Default {
                n644 = flat-sequence {
                  tunnel: [enum16{"Stop", "CoolingON", "HotGunON", "Start"}."Stop"] -> w1636
                  tunnel: [TRUE] -> w1635
                  frame #0 {
                    n645 = property on="VISA Tester" class="VISAName"() -> ("Value"=w1640:refnum<visa-resource-name>)  [unwired: 2 in, 2 out]
                    n646 = call "TesterOption (SubVI).vi"("2 Options"=FALSE, "On/Off"=FALSE, "Tester Option"=T11."Power", "VISA Refnum in"=w1640) -> ()  [unwired: 6 in, 2 out]
                  }
                  frame #1 {
                  }
                }
              }
              frame "CoolingON" {
                n647 = while {
                  tunnel: w1681 -> [w1716]
                  tunnel: w1680 -> [w1715]
                  tunnel: w1679 -> [w1711]
                  tunnel: [w1707] -> w1662
                  tunnel: w1673 -> [w1698]
                  tunnel: w1667 -> [w1708]
                  tunnel: w1666 -> [w1702]
                  tunnel: w1665 -> [w1699]
                  shift-right: [w1691] -> _
                  shift-left: 0.0 -> [w1692]
                  shift-right: [w1685] -> w1650
                  shift-left: 0.0 ("Value") -> [w1689]
                  tunnel: [w1686] -> w1646
                  stop <- w1696 stop-if-true
                  n648 = control-ref of="Power transistor Heat sink Temp."() -> (w1709:refnum<vi>)
                  n649 = property class="DigNum (strict)"(reference=w1709, error in=w1699) -> (error out=w1705:errorcluster, "Value"=w1685:dbl)  [unwired: 1 out]
                  n650 = Equal?(x=w1685, y=w1689) -> (x = y?=w1688:bool)
                  n651 = Number To Fractional String(number=w1685, precision (6)=i16 2) -> (F-format string=w1701:string)  [unwired: 2 in]
                  n652 = case shown="True" w1688 {
                    tunnel: w1692 -> [_ w1722]
                    tunnel: [0.0 w1720] -> w1691
                    tunnel: [FALSE w1719] -> w1690
                    frame False {
                    }
                    frame True {
                      n653 = Increment(x=w1722) -> (x+1=w1720:dbl)
                      n654 = Greater Or Equal?(x=w1720, y=300.0) -> (x >= y?=w1719:bool)
                    }
                  }
                  n655 = Concatenate Strings(w1702, "\nPCB Temperature [C]: " ("string"), w1701) -> (w1700:string)
                  n656 = call "Write panel message (SubVI).vi"("Stop BurnIn"=w1715, 4:"rpm"=w1711, 5:"rpm"=FALSE ("rpm"), "PrintTime"=FALSE, "Stop"=w1698, "error in (no error)"=w1705, "Time to wait"=0.2, "Strin"=w1700, "String in"=w1716) -> ("error out"=w1704:errorcluster)  [unwired: 2 in]
                  n657 = property class="Bool (strict)"(reference=w1698) -> ("Value"=w1697:bool)  [unwired: 1 in, 2 out]
                  n658 = Less Or Equal?(x=w1685, y=53.0) -> (x <= y?=w1687:bool)
                  n659 = call "GetADCTester (SubVI).vi"("error in (no error)"=w1704, "GetADCTester"=T13."Fan", "VISA Refnum in"=w1708) -> ("error out"=w1707:errorcluster, "ADCValOutput Single"=w1694:dbl)  [unwired: 6 in, 1 out]
                  n660 = Greater?(x=w1694, y=u32 2400) -> (0:w1686:bool)
                  n661 = Compound Arithmetic op=OR(w1686, w1697, w1687, w1690) -> (w1696:bool)
                }
                n662 = In Range and Coerce(upper limit=57.0, x=w1650, lower limit=53.0) -> (In Range?=w1645:bool)  [unwired: 1 out]
                n663 = Build Array(w1646, w1645) -> (w1647:bool[])
                n664 = And Array Elements(Boolean array=w1647) -> (logical AND=w1644:bool)
                "AuxiOFFResult" <- w1644
                n665 = Add(x=w1659, y=3) -> (x+y=w1657:i32)
                n666 = call "PassOrFail (SubVI).vi"("index (row)"=w1657, "error in (no error)"=w1662, "Data in"=w1650, "Pass?Fail"=w1645, "Table in"=w1655) -> ("error out"=w1661:errorcluster)  [unwired: 6 in]
                n667 = Select(t="OFF", s=w1646, f="ON") -> (s? t:f=w1651:string)
                n668 = Increment(x=w1657) -> (x+1=w1656:i32)
                n669 = property on="Test Failed" class="Bool (strict)"() -> ("Value"=w1643:bool)  [unwired: 2 in, 2 out]
                n670 = call "PassOrFail (SubVI).vi"("String Res"=w1651, "index (row)"=w1656, "error in (no error)"=w1661, "Data in"=-3.0, "Pass?Fail"=w1646, "Table in"=w1655) -> ("error out"=w1660:errorcluster)  [unwired: 5 in]
                n671 = case shown="False" w1643 {
                  tunnel: w1644 -> [w1683 _]
                  frame False {
                    n672 = Not(x=w1683) -> (.not. x?=w1684:bool)
                    n673 = property on="Test Failed" class="Bool (strict)"("Value"=w1684) -> ()  [unwired: 2 in, 2 out]
                  }
                  frame True {
                  }
                }
                n674 = call "TesterOption (SubVI).vi"("On/Off 2"=TRUE, "Tester Option 2"=T11."Power", "2 Options"=FALSE, "error in (no error)"=w1660, "On/Off"=FALSE, "Tester Option"=T11."Venable", "VISA Refnum in"=w1667) -> ("error out"=w1672:errorcluster)  [unwired: 3 in, 1 out]
                n675 = property class="Bool (strict)"(reference=w1673, error in=w1672) -> ("Value"=w1682:bool)  [unwired: 2 out]
                n676 = Select(t=enum16{"Stop", "CoolingON", "HotGunON", "Start"}."Stop", s=w1682, f=enum16{"Stop", "CoolingON", "HotGunON", "Start"}."Stop") -> (s? t:f=w1669:enum16{"Stop", "CoolingON", "HotGunON", "Start"})
              }
              frame "HotGunON" {
                n677 = while {
                  tunnel: w1763 -> [w1798]
                  tunnel: w1762 -> [w1797]
                  tunnel: w1761 -> [w1793]
                  tunnel: [w1789] -> w1731
                  tunnel: w1755 -> [w1780]
                  tunnel: w1749 -> [w1790]
                  tunnel: w1748 -> [w1784]
                  tunnel: w1747 -> [w1781]
                  shift-right: [w1773] -> _
                  shift-left: 0.0 -> [w1774]
                  shift-right: [w1770] -> _
                  shift-left: 0.0 ("Value") -> [w1771]
                  tunnel: [w1768] -> w1726
                  stop <- w1778 stop-if-true
                  n678 = control-ref of="Power transistor Heat sink Temp."() -> (w1791:refnum<vi>)
                  n679 = property class="DigNum (strict)"(reference=w1791, error in=w1781) -> (error out=w1787:errorcluster, "Value"=w1770:dbl)  [unwired: 1 out]
                  n680 = Equal?(x=w1770, y=w1771) -> (x = y?=w1769:bool)
                  n681 = Number To Fractional String(number=w1770, precision (6)=i16 2) -> (F-format string=w1783:string)  [unwired: 2 in]
                  n682 = case shown="True" w1769 {
                    tunnel: w1774 -> [_ w1804]
                    tunnel: [0.0 w1802] -> w1773
                    tunnel: [FALSE w1801] -> w1772
                    frame False {
                    }
                    frame True {
                      n683 = Increment(x=w1804) -> (x+1=w1802:dbl)
                      n684 = Greater Or Equal?(x=w1802, y=300.0) -> (x >= y?=w1801:bool)
                    }
                  }
                  n685 = Concatenate Strings(w1784, "\nPCB Temperature [C]: " ("string"), w1783) -> (w1782:string)
                  n686 = call "Write panel message (SubVI).vi"("Stop BurnIn"=w1797, 4:"rpm"=w1793, 5:"rpm"=FALSE ("rpm"), "PrintTime"=FALSE, "Stop"=w1780, "error in (no error)"=w1787, "Time to wait"=0.2, "Strin"=w1782, "String in"=w1798) -> ("error out"=w1786:errorcluster)  [unwired: 2 in]
                  n687 = property class="Bool (strict)"(reference=w1780) -> ("Value"=w1779:bool)  [unwired: 1 in, 2 out]
                  n688 = call "GetADCTester (SubVI).vi"("error in (no error)"=w1786, "GetADCTester"=T13."Fan", "VISA Refnum in"=w1790) -> ("error out"=w1789:errorcluster, "ADCValOutput Single"=w1776:dbl)  [unwired: 6 in, 1 out]
                  n689 = Greater Or Equal?(x=w1770, y=61.0) -> (x >= y?=w1767:bool)
                  n690 = Less?(x=w1776, y=u32 100) -> (x < y?=w1768:bool)
                  n691 = Compound Arithmetic op=OR(w1768, w1779, w1767, w1772) -> (w1778:bool)
                }
                n692 = control-ref of="Power transistor Heat sink Temp."() -> (w1732:refnum<vi>)
                n693 = call "Time Delay2"("error in (no error)"=w1731) -> ("error out"=w1728:errorcluster)  [unwired: 10 in]
                n694 = property class="DigNum (strict)"(reference=w1732, error in=w1728) -> (error out=w1730:errorcluster, "Value"=w1729:dbl)  [unwired: 1 out]
                n695 = In Range and Coerce(upper limit=62.0, x=w1729, lower limit=58.0) -> (In Range?=w1725:bool)  [unwired: 1 out]
                n696 = Build Array(w1726, w1725) -> (w1727:bool[])
                n697 = property on="Test Failed" class="Bool (strict)"() -> ("Value"=w1723:bool)  [unwired: 2 in, 2 out]
                n698 = Increment(x=w1742) -> (x+1=w1741:i32)
                n699 = call "PassOrFail (SubVI).vi"("index (row)"=w1741, "error in (no error)"=w1730, "Data in"=w1729, "Pass?Fail"=w1725, "Table in"=w1739) -> ("error out"=w1744:errorcluster)  [unwired: 6 in]
                n700 = And Array Elements(Boolean array=w1727) -> (logical AND=w1724:bool)
                "AuxiONResult" <- w1724
                n701 = Increment(x=w1741) -> (x+1=w1740:i32)
                n702 = Select(t="ON", s=w1726, f="OFF") -> (s? t:f=w1737:string)
                n703 = call "PassOrFail (SubVI).vi"("String Res"=w1737, "index (row)"=w1740, "error in (no error)"=w1744, "Data in"=-3.0, "Pass?Fail"=w1726, "Table in"=w1739) -> ("error out"=w1743:errorcluster)  [unwired: 5 in]
                n704 = case shown="False" w1723 {
                  tunnel: w1724 -> [w1765 _]
                  frame False {
                    n705 = Not(x=w1765) -> (.not. x?=w1766:bool)
                    n706 = property on="Test Failed" class="Bool (strict)"("Value"=w1766) -> ()  [unwired: 2 in, 2 out]
                  }
                  frame True {
                  }
                }
                n707 = call "TesterOption (SubVI).vi"("On/Off 2"=TRUE, "Tester Option 2"=T11."Fan", "2 Options"=FALSE, "error in (no error)"=w1743, "On/Off"=FALSE, "Tester Option"=T11."Venable", "VISA Refnum in"=w1749) -> ("error out"=w1754:errorcluster)  [unwired: 3 in, 1 out]
                n708 = property class="Bool (strict)"(reference=w1755, error in=w1754) -> ("Value"=w1764:bool)  [unwired: 2 out]
                n709 = Select(t=enum16{"Stop", "CoolingON", "HotGunON", "Start"}."Stop", s=w1764, f=enum16{"Stop", "CoolingON", "HotGunON", "Start"}."CoolingON") -> (s? t:f=w1751:enum16{"Stop", "CoolingON", "HotGunON", "Start"})
              }
              frame "Start" {
                n710 = call "Write panel message (SubVI).vi"("Stop BurnIn"=w1824, 4:"rpm"=w1820, 5:"rpm"=FALSE ("rpm"), "PrintTime"=FALSE, "Stop"=w1811, "Time to wait"=0.1, "Strin"=w1819, "String in"=w1825) -> ("error out"=w1818:errorcluster)  [unwired: 3 in]
                n711 = call "TesterOption (SubVI).vi"("On/Off 2"=TRUE, "Tester Option 2"=T11."Fan", "2 Options"=TRUE, "error in (no error)"=w1818, "On/Off"=FALSE, "Tester Option"=T11."Venable", "VISA Refnum in"=w1812) -> ("error out"=w1810:errorcluster)  [unwired: 3 in, 1 out]
                n712 = call "Time Delay"("error in (no error)"=w1810) -> ("error out"=w1805:errorcluster)  [unwired: 10 in]
                n713 = property class="Bool (strict)"(reference=w1811, error in=w1805) -> ("Value"=w1826:bool)  [unwired: 2 out]
                n714 = Select(t=enum16{"Stop", "CoolingON", "HotGunON", "Start"}."Stop", s=w1826, f=enum16{"Stop", "CoolingON", "HotGunON", "Start"}."HotGunON") -> (s? t:f=w1807:enum16{"Stop", "CoolingON", "HotGunON", "Start"})
              }
            }
          }
        }
      }
    }
    n715 = flat-sequence {
      tunnel: w183 -> [_]
      frame #0 {
        w191 = T18."Enabled" ("Disabled")
        w192 = FALSE ("Start")
        n716 = property on="Start" class="Bool (strict)"("Value"=w192, "DisabledEnum"=w191) -> ()  [unwired: 2 in, 2 out]
        n717 = property on="Report" class="Bool (strict)"("Value"=w192, "DisabledEnum"=w191) -> ()  [unwired: 2 in, 2 out]
      }
    }
  }
  n718 = while {
    shift-right: [w1845] -> _
    shift-left: T10."Initialize" -> [w1844]
    shift-right: [w1841] -> _
    shift-left: w17 -> [w1842]
    shift-right: [w1840] -> _
    shift-left: _ -> [w1839]
    shift-right: [w1838] -> _
    shift-left: w20 -> [w1836]
    shift-right: [w1837] -> _
    shift-left: refnum<vi> refnum ("Config_CANAT") -> [w1835]
    shift-right: [w1833] -> _
    shift-left: w16 -> [w1834]
    tunnel: "ATR" -> [_]
    tunnel: w7 -> [w1832]
    tunnel: w6 -> [w1831]
    shift-right: [w1829] -> _
    shift-left: 0 -> [w1830]
    tunnel: w4 -> [w1828]
    tunnel: w2 -> [w1827]
    tunnel: w1 -> [_]
    stop <- w1843 stop-if-true
    n719 = case shown="\"MainProgram\"" w1844 {
      tunnel: [T10."MainProgram" w1938 w1988 T10."Erase ATR Table"] -> w1845
      tunnel: [FALSE TRUE FALSE FALSE] -> w1843
      tunnel: [w1849 w1932 w1982 w2784] -> w1841
      tunnel: w1842 -> [_ w1951 w1986 _]
      tunnel: [w1889 refnum<visa-resource-name> refnum ("VISA resource name") w1983 w2789] -> w1840
      tunnel: w1839 -> [w1889 w1961 w1984 _]
      tunnel: [w1876 refnum<queue> refnum ("queue out") w1978 w2782] -> w1838
      tunnel: [w1875 refnum<vi> refnum ("Config_CANAT") w1979 w2785] -> w1837
      tunnel: w1836 -> [w1876 w1963 w1981 w2782]
      tunnel: w1835 -> [w1875 w1942 w1980 _]
      tunnel: w1834 -> [w1874 w1955 w1977 w2781]
      tunnel: [w1874 refnum<queue> refnum ("queue out") w1976 w2781] -> w1833
      tunnel: w1832 -> [_ _ w1975 _]
      tunnel: w1831 -> [_ _ w1974 _]
      tunnel: w1830 -> [w1863 w1945 w1973 w2778]
      tunnel: [w1863 w1945 w1972 w2778] -> w1829
      tunnel: w1828 -> [w1853 _ w1971 _]
      tunnel: w1827 -> [_ _ w1970 _]
      frame "Erase ATR Table", Default {
        w1857 = "Marvin" ("section")
        w1870 = refnum<visa-resource-name> "COM4" ("VISA resource name")
        w1884 = FALSE ("Visible")
        n720 = property on="Serial Com" class="Bool"(error in=errorcluster {"status"=FALSE, "code"=0, "source"=""} ("error out"), "Visible"=TRUE) -> (error out=w1871:errorcluster)  [unwired: 1 in, 1 out]
        n721 = property on="VISA Marvin" class="VISAName"(error in=w1871, "Visible"=w1884, "Value"=w1870) -> (error out=w1886:errorcluster)  [unwired: 1 in, 1 out]
        n722 = property on="VISA Marvin" class="VISAName"(error in=w1871, "Value"=w1870) -> ()  [unwired: 1 in, 2 out]
        n723 = case shown="False" w1881 {
          tunnel: [string[][] [["6.1", "Visual Inspection", "", "", "", "", ""], ["6.1.1", "Verification of Components Not Installed", "N/A", "-", "", "", ""], ["", "", "", "", "", "", ""], ["6.1.2", "Manufacturing Defects", "N/A", "-", "", "", ""], ["", "", "", "", "", "", ""], ["6.2", "Power Supply Testing", "", "", "", "", ""], ["6.2.1", "Input Current Drawn", "", "", "", "", ""], ["6.2.1.1", "DC Input Current", "< 150", "-", "mA", "", ""], ["", "", "", "", "", "", ""], ["6.2.2", "Power Supply Voltages", "", "", "", "", ""], ["6.2.2.1", "12V", "12.0", "+/-0.500", "V", "", ""], ["6.2.2.2", "5V", "5.0", "+/-0.200", "V", "", ""], ["6.2.2.3", "3.3V", "3.3", "+/-0.100", "V", "", ""], ["6.2.2.4", "1.8V", "1.8", "+/-0.100", "V", "", ""], ["", "", "", "", "", "", ""], ["7", "Functional Test Procedure", "", "", "", "", ""], ["7.1", "Weight Check", "3800", "+/-100.0", "gr", "", ""], ["", "", "", "", "", "", ""], ["7.2", "Insulation Resistance Test", "", "", "", "", ""], ["7.2.1", "J3.B to Chassis", "> 1M", "-", "W", "", ""], ["7.2.2", "J1.16 to Chassis", "> 100K", "-", "W", "", ""], ["", "", "", "", "", "", ""], ["7.2", "Bonding Resistance", "", "", "", "", ""], ["7.2.3", "J1 Body to Chassis", "< 2m", "-", "W", "", ""], ["7.2.4", "J2  Body to Chassis", "< 2m", "-", "W", "", ""], ["7.2.5", "J3  Body to Chassis", "< 2m", "-", "W", "", ""], ["", "", "", "", "", "", ""], ["7.2.1", "CANbus Resistance Test", "", "", "", "", ""], ["7.2.1.1", "J1.17 to J1.18", "> 10K", "-", "W", "", ""], ["", "", "", "", "", "", ""], ["7.3", "Sealing Test", "N/A", "-", "", "", ""], ["", "", "", "", "", "", ""], ["7.4", "Communication Test", "", "", "", "", ""], ["7.4.1", "Serial RS-232", "N/A", "-", "", "", ""], ["7.4.2", "CAN Bus", "N/A", "-", "", "", ""], ["", "", "", "", "", "", ""], ["7.5", "Performances Tests", "", "", "", "", ""], ["7.5.1", "Reverse Polarity Test", "", "", "", "", ""], ["7.5.1.1", "DC Input Current", "< 1", "-", "mA", "", ""], ["", "", "", "", "", "", ""], ["7.5.2", "Enable Test", "", "", "", "", ""], ["7.5.2.1", "Fan Speed at Opened Enable ", "5000", "+/-200.0", "rpm", "", ""], ["7.5.2.2", "Fan Speed at Opened Enable ", "0", "+/-200.0", "rpm", "", ""], ["7.5.2.3", "Fan Speed at Closed Enable ", "5000", "+/-200.0", "rpm", "", ""], ["7.5.2.4", "Motor Rotation Direction", "Counter-clockwise (Inlet)", "-", "", "", ""], ["", "", "", "", "", "", ""], ["7.5.3", "Stop Time Test ", "", "", "", "", ""], ["7.5.3.1", "Motor Stop time", "< 50", "-", "sec", "", ""], ["", "", "", "", "", "", ""], ["7.5.4", "Speed Command Test", "", "", "", "", ""], ["7.5.4.1", "Fan Speed", "6000", "+/-200.0", "rpm", "", ""], ["7.5.4.2", "Fan Speed", "9000", "+/-200.0", "rpm", "", ""], ["7.5.4.3", "Fan Speed", "12100", "+/-200.0", "rpm", "", ""], ["", "", "", "", "", "", ""], ["7.5.5", "Temperature Sensor Calibration Test", "", "", "", "", ""], ["7.5.5.1", "Sensor Reading Analog Offset", "0", "+/-0.100", ".", "", ""], ["", "", "", "", "", "", ""], ["7.5.6", "Burn-in Test", "", "", "", "", ""], ["7.5.6.1", "DC Input Current", "28", "+/-3.000", "A", "", ""], ["7.5.6.2", "Fan Speed", "12100", "+/-200.000", "rpm", "", ""], ["7.5.6.3", "Ambient Temperature", "25", "+/-13.00", "C", "", ""], ["7.5.6.4", "After 10 min of operation", "", "", "C", "", ""], ["7.5.6.5", "After 20 min of operation", "", "", "C", "", ""], ["7.5.6.6", "After 30 min of operation", "", "", "C", "", ""], ["", "", "", "", "", "", ""], ["9", "Motor Temp Test", "", "", "", "", ""], ["9.1", "60 C", "60", "+/-3.000", "C", "", ""], ["9.2", "90 C", "90", "+/-3.000", "C", "", ""], ["9.3", "120 C", "120", "+/-3.000", "C", "", ""]] ("data") string[][] [["6.1", "Visual Inspection", "", "", "", "", ""], ["6.1.1", "Verification of Components Not Installed", "N/A", "-", "", "", ""], ["", "", "", "", "", "", ""], ["6.1.2", "Manufacturing Defects", "N/A", "-", "", "", ""], ["", "", "", "", "", "", ""], ["6.2", "Power Supply Testing", "", "", "", "", ""], ["6.2.1", "Input Current Drawn", "", "", "", "", ""], ["6.2.1.1", "DC Input Current", "< 150", "-", "mA", "", ""], ["", "", "", "", "", "", ""], ["6.2.2", "Power Supply Voltages", "", "", "", "", ""], ["6.2.2.1", "12V", "12.0", "+/-0.500", "V", "", ""], ["6.2.2.2", "5V", "5.0", "+/-0.200", "V", "", ""], ["6.2.2.3", "3.3V", "3.3", "+/-0.100", "V", "", ""], ["6.2.2.4", "1.8V", "1.8", "+/-0.100", "V", "", ""], ["", "", "", "", "", "", ""], ["7", "Functional Test Procedure", "", "", "", "", ""], ["7.1", "Weight Check", "4180", "+/-10.00", "gr", "", ""], ["", "", "", "", "", "", ""], ["7.2", "Insulation Resistance Test", "", "", "", "", ""], ["7.2.1", "J3.B to Chassis", "> 1M", "-", "W", "", ""], ["7.2.2", "J1.16 to Chassis", "> 100K", "-", "W", "", ""], ["", "", "", "", "", "", ""], ["7.2", "Bonding Resistance", "", "", "", "", ""], ["7.2.3", "J1 Body to Chassis", "< 2m", "-", "W", "", ""], ["7.2.4", "J2  Body to Chassis", "< 2m", "-", "W", "", ""], ["7.2.5", "J3  Body to Chassis", "< 2m", "-", "W", "", ""], ["", "", "", "", "", "", ""], ["7.2.1", "CANbus Resistance Test", "", "", "", "", ""], ["7.2.1.1", "J1.17 to J1.18", "> 10K", "-", "W", "", ""], ["", "", "", "", "", "", ""], ["7.3", "Sealing Test", "N/A", "-", "", "", ""], ["", "", "", "", "", "", ""], ["7.4", "Communication Test", "", "", "", "", ""], ["7.4.1", "Serial RS-232", "N/A", "-", "", "", ""], ["7.4.2", "CAN Bus", "N/A", "-", "", "", ""], ["", "", "", "", "", "", ""], ["7.5", "Performances Tests", "", "", "", "", ""], ["7.5.1", "Reverse Polarity Test", "", "", "", "", ""], ["7.5.1.1", "DC Input Current", "< 1", "-", "mA", "", ""], ["", "", "", "", "", "", ""], ["7.5.2", "Enable Test", "", "", "", "", ""], ["7.5.2.1", "Fan Speed at Opened Enable ", "5000", "+/-200.0", "rpm", "", ""], ["7.5.2.2", "Fan Speed at Opened Enable ", "0", "+/-200.0", "rpm", "", ""], ["7.5.2.3", "Fan Speed at Closed Enable ", "5000", "+/-200.0", "rpm", "", ""], ["7.5.2.4", "Motor Rotation Direction", "Counter-clockwise (Inlet)", "-", "", "", ""], ["", "", "", "", "", "", ""], ["7.5.3", "Stop Time Test ", "", "", "", "", ""], ["7.5.3.1", "Motor Stop time", "< 50", "-", "sec", "", ""], ["", "", "", "", "", "", ""], ["7.5.4", "Speed Command Test", "", "", "", "", ""], ["7.5.4.1", "Fan Speed", "6000", "+/-200.0", "rpm", "", ""], ["7.5.4.2", "Fan Speed", "11500", "+/-200.0", "rpm", "", ""], ["7.5.4.3", "Fan Speed", "15100", "+/-200.0", "rpm", "", ""], ["", "", "", "", "", "", ""], ["7.5.5", "Temperature Sensor Calibration Test", "", "", "", "", ""], ["7.5.5.1", "Sensor Reading Analog Offset", "0", "+/-0.100", ".", "", ""], ["", "", "", "", "", "", ""], ["7.5.6", "Temperature Control Algorithm Test", "", "", "", "", ""], ["7.5.6.1", "Tair <   68 ± 2 oC", "6000", "+/-200.0", "rpm", "", ""], ["7.5.6.2", "Measured Temp.", "", "", "C", "", ""], ["7.5.6.3", "Tair >= 68 ± 2 oC", "11500", "+/-200.0", "rpm", "", ""], ["7.5.6.4", "Transition Temp.", "", "", "C", "", ""], ["7.5.6.5", "Tair >= 88 ± 2 oC", "15100", "+/-400.0", "rpm", "", ""], ["7.5.6.6", "Transition Temp.", "", "", "C", "", ""], ["7.5.6.7", "Tair <= 80 ± 2 oC", "11500", "+/-200.0", "rpm", "", ""], ["7.5.6.8", "Transition Temp.", "", "", "C", "", ""], ["7.5.6.9", "Tair <= 60 ± 2 oC", "6000", "+/-200.0", "rpm", "", ""], ["7.5.6.10", "Transition Temp.", "", "", "C", "", ""], ["", "", "", "", "", "", ""], ["7.5.7", "Burn-in Test", "", "", "", "", ""], ["7.5.7.1", "DC Input Current", "50", "+/-5.000", "A", "", ""], ["7.5.7.2", "Fan Speed", "15100", "+/-200.0", "rpm", "", ""], ["7.5.7.3", "Ambient Temperature", "25", "+/-13.00", "C", "", ""], ["7.5.7.4", "After 10 min of operation", "", "-", "C", "", ""], ["7.5.7.5", "After 20 min of operation", "", "-", "C", "", ""], ["7.5.7.6", "After 30 min of operation", "", "-", "C", "", ""], ["", "", "", "", "", "", ""], ["8", "Auxiliary", "", "", "", "", ""], ["8.1", "Auxiliary Cooling Fan ON", "60", "+/-2.00", "C", "", ""], ["8.2", "Fan status", "ON", "-", "-", "", ""], ["8.3", "Auxiliary Cooling Fan OFF", "55", "+/-2.00", "C", "", ""], ["8.4", "Fan status", "OFF", "-", "-", "", ""], ["", "", "", "", "", "", ""], ["9", "Motor Temp. Test", "", "", "", "", ""], ["9.1", "60 Degree", "60", "+/-3.00", "C", "", ""], ["9.2", "90 Degree", "90", "+/-3.00", "C", "", ""], ["9.3", "120 Degree", "120", "+/-3.00", "C", "", ""]] ("data")] -> w1882
          tunnel: ["AHU" "EBAY"] -> w1880
          tunnel: [w1903 w1915] -> w1877
          tunnel: w1878 -> [w1904 w1915]
          tunnel: [w1899 u8 95] -> w1850
          frame False {
            n724 = while {
              shift-right: [w1912] -> w1903
              shift-left: w1904 -> [w1913]
              tunnel: [w1907] -> w1902
              stop <- w1911 stop-if-true
              n725 = call "AHU UUT (subVI).vi"("error in (no error)"=w1913) -> ("AHU 47"=w1908:bool, "AHU 63"=w1907:bool, "OK"=w1910:bool, "error out"=w1912:errorcluster)  [unwired: 15 in]
              n726 = Exclusive Or(1:w1908, 2:w1907) -> (0:w1909:bool)
              n727 = And(x=w1910, y=w1909) -> (x .and. y?=w1911:bool)
            }
            n728 = Select(t=u8 63, s=w1902, f=u8 47) -> (s? t:f=w1899:u8)
          }
          frame True {
          }
        }
        "UUT" <- w1880
        "UUT" <- w1850
        n729 = property on="Status" class="Bool (strict)"(error in=w1886, "Value"=w1884) -> (error out=w1879:errorcluster)  [unwired: 1 in, 1 out]
        n730 = flat-sequence {
          tunnel: [w1896] -> w1881
          tunnel: w1879 -> [w1894]
          tunnel: [w1894] -> w1878
          frame #0 {
            n731 = Two Button Dialog(message="Please seect the Unit Under Test.", 1:"AHU" ("F button name (\"Cancel\")"), 2:"EBAY" ("T button name (\"OK\")")) -> (T button?=w1896:bool)
          }
        }
        n732 = for {
          tunnel: w1882 -> [w1922] mode=indexing
          tunnel: w1877 -> [w1920]
          tunnel: [w1919] -> w1873
          tunnel: w1882 -> [w1918]
          i -> [w1921]
          n733 = for {
            tunnel: w1922 -> [_] mode=indexing
            tunnel: w1921 -> [w1928]
            tunnel: w1920 -> [w1925]
            tunnel: [w1924] -> w1919
            tunnel: w1918 -> [w1923]
            i -> [w1929]
            n734 = Bundle By Name(cluster=T19 {"Row"=0, "Column"=0} ("Active Cell:Active Cell"), "Row"=w1928, "Column"=w1929) -> (w1927:T19)
            n735 = control-ref of="ATR"() -> (w1926:refnum<vi>)
            n736 = property class="Tbl (strict)"(reference=w1926, error in=w1925, "Active Cell"=w1927, "Cell BG Color"=u32 16777226, "Value"=w1923) -> (error out=w1924:errorcluster)  [unwired: 1 out]
          }
        }
        n737 = call "COM EvolutionBoard.vi"("error in (no error)"=w1873, "VISA resource name 2"=refnum<visa-resource-name> "COM1" ("VISA resource name")) -> ("error out"=w1869:errorcluster, "VISA resource name out"=w1868:refnum<visa-resource-name>)  [unwired: 8 in]
        n738 = call "TesterOption (SubVI).vi"("2 Options"=FALSE, "error in (no error)"=w1869, "On/Off"=FALSE, "Tester Option"=T11."Venable", "VISA Refnum in"=w1868) -> ("error out"=w1849:errorcluster, "VISA Refnum out"=→"VISA Tester":refnum<visa-resource-name>)  [unwired: 5 in]
        n739 = case shown="95" w1850 {
          tunnel: ["AHU Software Version" ("key") "EBAY Software Version" ("key")] -> w1859
          tunnel: ["AHU Serial Number" ("key") "EBAY Serial Number" ("key")] -> w1860
          frame 47, 63, Default {
          }
          frame 95 {
          }
        }
        n740 = call <vilib>:"Open Config Data.vi"("create file if necessary (T)"=FALSE, "configuration file path"=w1853) -> ("error out"=w1854:errorcluster, "refnum"=w1855:T24)  [unwired: 1 in, 7 out]
        n741 = call-poly <vilib>:"Read Key.vi"("section"=w1857, "error in (no error)"=w1854, "key"=w1859, "refnum"=w1855) -> ("error out"=w1861:errorcluster, "value"=→"UUT SoftwareVer":string, "refnum out"=w1858:T24)  [unwired: 2 in, 3 out]
        n742 = call-poly <vilib>:"Read Key.vi"("section"=w1857, "error in (no error)"=w1861, "key"=w1860, "refnum"=w1858) -> ("error out"=w1848:errorcluster, "value"=w1846:string, "refnum out"=w1847:T24)  [unwired: 2 in, 3 out]
        n743 = call <vilib>:"Close Config Data.vi"("error in (no error)"=w1848, "refnum"=w1847) -> ()  [unwired: 8 in, 2 out]
        n744 = Decimal String To Number(string=w1846) -> (number=w1851:i32)  [unwired: 2 in, 1 out]
        n745 = Increment(x=w1851) -> (x+1=→"Next SN":i32)
      }
      frame "Stop" {
        n746 = flat-sequence {
          tunnel: w1951 -> [w1967]
          tunnel: [w1966] -> w1944
          frame #0 {
            n747 = control-ref of="Pannel User Message"() -> (w1969:refnum<vi>)
            n748 = property class="Str"(reference=w1969, error in=w1967, "Value"="Program Stopped...\r\nPlease turn OFF All Power sinks") -> (error out=w1966:errorcluster)  [unwired: 1 out]
          }
        }
        n749 = control-ref of="VISA Tester"() -> (w1953:refnum<vi>)
        n750 = property class="VISAName"(reference=w1953, error in=w1944) -> ("Value"=w1950:refnum<visa-resource-name>)  [unwired: 2 out]
        n751 = call "Clear CAN Buffer.vi"("error in (no error)"=w1944, "Cluster in"=w1942) -> ("error out"=w1943:errorcluster)  [unwired: 8 in, 1 out]
        n752 = call "Close CAN Device.vi"("error in (no error)"=w1943, "Cluster in"=w1942) -> ()  [unwired: 8 in, 2 out]
        n753 = VISA Close(VISA resource name=w1961, error in (no error)=w1944) -> (error out=w1954:errorcluster)
        n754 = call "TesterOption (SubVI).vi"("2 Options"=FALSE, "On/Off"=FALSE, "Tester Option"=T11."Power", "VISA Refnum in"=w1950) -> ("error out"=w1937:errorcluster, "VISA Refnum out"=w1949:refnum<visa-resource-name>)  [unwired: 6 in]
        n755 = VISA Close(VISA resource name=w1949, error in (no error)=w1937) -> (error out=w1934:errorcluster)
        n756 = Flush Queue(queue=w1955, error in (no error)=w1954) -> (queue out=w1957:refnum<queue>, error out=w1956:errorcluster)  [unwired: 1 out]
        n757 = Flush Queue(queue=w1963, error in (no error)=w1954) -> (queue out=w1962:refnum<queue>, error out=w1964:errorcluster)  [unwired: 1 out]
        n758 = property on="Refresh Button" class="Bool (strict)"() -> ("Value"=w1941:bool)  [unwired: 2 in, 2 out]
        n759 = Release Queue(queue=w1957, error in (no error)=w1956) -> (error out=w1935:errorcluster)  [unwired: 1 in, 2 out]
        n760 = Release Queue(queue=w1962, error in (no error)=w1964) -> (error out=w1936:errorcluster)  [unwired: 1 in, 2 out]
        n761 = Select(t=T10."Initialize", s=w1941, f=T10."Stop") -> (s? t:f=w1938:T10)
        n762 = Merge Errors(w1936, w1935, w1934) -> (w1933:errorcluster)
        n763 = call <vilib>:"Clear Errors.vi"("error in (no error)"=w1933) -> ("error out"=w1932:errorcluster)  [unwired: 5 in, 1 out]
      }
      frame "MainProgram" {
        n764 = event shown="[8] \"Help Button\": Value Change" {
          selector: w1975 -> [_ _ _ _ _ _ _ _ _ _ _ _ _]
          dyn-events: _ -> [_ _ _ _ _ _ _ _ _ _ _ _ _]
          timeout: 50 -> [_ _ _ _ _ _ _ _ _ _ _ _ _]
          tunnel: [T10."MainProgram" T10."MainProgram" T10."MainProgram" T10."MainProgram" T10."MainProgram" T10."MainProgram" T10."MainProgram" w2531 T10."MainProgram" T10."MainProgram" T10."MainProgram" T10."Stop" T10."MainProgram"] -> w1988
          tunnel: [w1994 w2109 w2163 w2170 w2179 w2197 w2204 w2591 w2646 w2659 w2667 w2747 w2753] -> w1982
          tunnel: w1986 -> [w1998 w2109 w2162 w2172 w2179 w2197 w2212 w2591 w2647 w2658 w2666 w2747 w2758]
          tunnel: [w2007 w2083 w2164 w2171 w2180 w2195 w2200 w2539 w2644 w2656 w2668 w2745 w2751] -> w1983
          tunnel: w1984 -> [w2007 w2083 w2164 w2171 w2180 w2195 w2200 w2539 w2644 w2656 _ w2745 w2751]
          tunnel: w1981 -> [w2000 w2115 w2158 w2167 w2176 w2194 w2209 w2571 w2643 w2655 w2671 w2744 w2756]
          tunnel: w1980 -> [w1995 w2114 w2159 w2168 w2177 w2193 w2210 w2570 w2642 w2654 w2670 w2743 w2749]
          tunnel: [w1997 w2114 w2159 w2168 w2177 w2193 w2210 w2570 w2642 w2654 w2670 w2743 w2749] -> w1979
          tunnel: [w1999 w2115 w2158 w2167 w2176 w2194 w2209 w2571 w2643 w2655 w2671 w2744 w2756] -> w1978
          tunnel: w1977 -> [w1992 w2113 w2157 w2166 w2175 w2192 w2208 w2569 w2641 w2653 w2669 w2742 w2755]
          tunnel: [w1992 w2113 w2157 w2166 w2175 w2192 w2203 w2569 w2641 w2653 w2669 w2742 w2755] -> w1976
          tunnel: w1974 -> [_ _ _ _ _ _ _ w2537 _ _ _ _ _]
          tunnel: w1973 -> [w1993 w2112 w2156 w2165 w2174 w2190 w2198 w2544 w2640 w2652 w2664 w2741 w2754]
          tunnel: [w1993 w2112 w2156 w2165 w2174 w2190 w2198 w2543 w2640 w2652 w2664 w2741 w2754] -> w1972
          tunnel: w1971 -> [_ w2110 _ _ _ _ _ w2542 _ _ _ _ _]
          tunnel: w1970 -> [_ w2081 _ _ _ _ _ _ _ _ _ _ _]
          event Timeout {
            n765 = event-data() -> ()  [unwired: 1 in, 3 out]
            n766 = property class="Clust (strict)"(reference=w1995, error in=w1998) -> (reference out=w1997:refnum<vi>, error out=w1996:errorcluster, "Value"=w2004:T7)
            n767 = Unbundle By Name(w2004) -> ("DevType"=w2005:T2, "CanIndex"=w2002:T1)
            n768 = call "VCI_Receive.vi"("CANIndex"=w2002, "DevIndex"=u32 0, "DevType"=w2005) -> ("Recieve"=w2001:T25[])  [unwired: 3 in, 5 out]
            n769 = Empty Array?(array=w2001) -> (empty?=w2003:bool)
            n770 = case shown="False" w2003 {
              tunnel: w2002 -> [w2045 _]
              tunnel: w1997 -> [w2043 _]
              tunnel: w2000 -> [w2042 w2078]
              tunnel: w1996 -> [w2041 w2077]
              tunnel: w2001 -> [w2046 _]
              tunnel: [w2036 w2077] -> w1994
              tunnel: [w2035 w2078] -> w1999
              tunnel: [w2034 0] -> _
              frame False {
                n771 = call "Demo_MakeDispBuff.vi"("Channel"=w2045, "Type"=enum16{"接收", "发送"}."接收", "OBJs"=w2046) -> ("Buffer"=w2044:T26)
                n772 = for {
                  N: 3 -> [_]
                  tunnel: w2044 -> [w2060]
                  tunnel: w2043 -> [w2059]
                  tunnel: w2042 -> [w2050]
                  tunnel: w2041 -> [w2049]
                  tunnel: [w2052] -> w2039 mode=indexing
                  tunnel: [w2050] -> w2038
                  tunnel: [w2049] -> w2037
                  tunnel: [w2048] -> w2034
                  i -> [w2048]
                  n773 = property class="Clust (strict)"(reference=w2059) -> ("Value"=w2057:T7)  [unwired: 1 in, 2 out]
                  n774 = Index Array(array=w2060, index=w2048) -> (element=w2053:T27)
                  n775 = Unbundle By Name(w2053) -> ("Channel"=w2055:T1, "VCI_CAN_OBJ"=w2058:T25)  [unwired: 2 out]
                  n776 = Unbundle By Name(w2057) -> ("CanIndex"=w2056:T1)
                  n777 = Equal?(x=w2056, y=w2055) -> (x = y?=w2054:bool)
                  n778 = case shown="True" w2054 {
                    tunnel: w2058 -> [_ w2071]
                    tunnel: [w2061 w2067] -> w2052
                    tunnel: T21 {"ID"=0, "MSGTYPE"=0, "LEN"=0, "aDATA"=[]} ("Msg") -> [w2061 w2066]
                    frame False {
                    }
                    frame True {
                      n779 = Unbundle By Name(w2071) -> ("ID"=w2065:u32, "DataLen"=w2070:u8, "Data"=w2068:u8[])
                      n780 = Bundle By Name(cluster=w2066, "ID"=w2065, "MSGTYPE"=u8 0, "LEN"=w2070, "aDATA"=w2068) -> (w2067:T21)
                      n781 = Unbundle By Name(w2067) -> ("ID"=w2063:u32)
                      n782 = Split Number(x=w2063) -> (lo(x)=w2064:u16)  [unwired: 1 out]
                      n783 = Split Number(x=w2064) -> (lo(x)=w2062:u8)  [unwired: 1 out]
                      n784 = case shown="63" w2062 {
                        tunnel: ["EBAY 5F" "" "AHU 3F" "AHU 2F"] -> _
                        frame 95 {
                        }
                        frame Default {
                        }
                        frame 63 {
                        }
                        frame 47 {
                        }
                      }
                    }
                  }
                }
                n785 = Enqueue Element(queue=w2038, element=w2039, error in (no error)=w2037) -> (queue out=w2035:refnum<queue>, error out=w2036:errorcluster)  [unwired: 2 out]
              }
              frame True {
              }
            }
            n786 = disable-structure shown="Disabled" {
              frame Disabled {
                n787 = property on="SpeedResult" class="Bool (strict)"() -> ("Value"=w2021:bool)  [unwired: 2 in, 2 out]
                n788 = property on="VenableResult" class="Bool (strict)"() -> ("Value"=w2019:bool)  [unwired: 2 in, 2 out]
                n789 = property on="VenableDirectionResult" class="Bool (strict)"() -> ("Value"=w2020:bool)  [unwired: 2 in, 2 out]
                n790 = property on="ComTestResult" class="Bool (strict)"() -> ("Value"=w2018:bool)  [unwired: 2 in, 2 out]
                n791 = property on="AuxiOFFResult" class="Bool (strict)"() -> ("Value"=w2022:bool)  [unwired: 2 in, 2 out]
                n792 = property on="AuxiONResult" class="Bool (strict)"() -> ("Value"=w2023:bool)  [unwired: 2 in, 2 out]
                n793 = property on="VisualInspectionResult" class="Bool (strict)"() -> ("Value"=w2025:bool)  [unwired: 2 in, 2 out]
                n794 = property on="SensCalResult" class="Bool (strict)"() -> ("Value"=w2024:bool)  [unwired: 2 in, 2 out]
                n795 = property on="BurnDC" class="Bool (strict)"() -> ("Value"=w2026:bool)  [unwired: 2 in, 2 out]
                n796 = property on="BurnTemp" class="Bool (strict)"() -> ("Value"=w2027:bool)  [unwired: 2 in, 2 out]
                n797 = property on="BurnSpeed" class="Bool (strict)"() -> ("Value"=w2028:bool)  [unwired: 2 in, 2 out]
                n798 = property on="BurnResult" class="Bool (strict)"() -> ("Value"=w2029:bool)  [unwired: 2 in, 2 out]
                n799 = property on="StopTimeResult" class="Bool (strict)"() -> ("Value"=w2030:bool)  [unwired: 2 in, 2 out]
                n800 = property on="MotorTempResult" class="Bool (strict)"() -> ("Value"=w2031:bool)  [unwired: 2 in, 2 out]
                n801 = property on="TempControlResult" class="Bool (strict)"() -> ("Value"=w2032:bool)  [unwired: 2 in, 2 out]
                n802 = Build Array(w2018, w2019, w2020, w2021, w2022, w2023, w2024, w2025, w2026, w2027, w2028, w2029, w2030, w2031, w2032) -> (w2017:bool[])
                n803 = And Array Elements(Boolean array=w2017) -> (logical AND=w2033:bool)
                n804 = Not(x=w2033) -> ()  [unwired: 1 out]
              }
              frame Enabled {
              }
            }
            n805 = disable-structure shown="Disabled" {
              disable-tunnel: w1992 -> [w2012 _]
              frame Disabled {
                n806 = Preview Queue Element(queue=w2012) -> (element=w2011:T8)  [unwired: 2 in, 3 out]
                n807 = Unbundle By Name(w2011) -> ("Array Test"=w2010:T16)
                n808 = for {
                  tunnel: w2010 -> [w2015] mode=indexing
                  tunnel: [w2013] -> w2009 mode=indexing
                  n809 = Equal?(x=w2015, y=T20."Empty") -> (x = y?=w2013:bool)
                }
                n810 = And Array Elements(Boolean array=w2009) -> ()  [unwired: 1 out]
              }
              frame Enabled {
              }
            }
            n811 = property on="Automation" class="Bool (strict)"() -> ("Value"=w1989:bool)  [unwired: 2 in, 2 out]
            n812 = property on="Start" class="Bool (strict)"() -> ("Value"=w1991:bool)  [unwired: 2 in, 2 out]
            n813 = Or(x=w1989, y=w1991) -> (x .or. y?=w1990:bool)
            n814 = case shown="False" w1990 {
              frame False {
                n815 = property on="Pannel User Message" class="Str"("Value"="You can press start to execute(s) test(s).") -> ()  [unwired: 2 in, 2 out]
              }
              frame True {
              }
            }
          }
          event "SetSN": Value Change {
            n816 = event-data() -> ()  [unwired: 1 in, 6 out]
            n817 = property on="SpeedResult" class="Bool (strict)"() -> ("Value"=w2092:bool)  [unwired: 2 in, 2 out]
            n818 = property on="VenableResult" class="Bool (strict)"() -> ("Value"=w2090:bool)  [unwired: 2 in, 2 out]
            n819 = property on="VenableDirectionResult" class="Bool (strict)"() -> ("Value"=w2091:bool)  [unwired: 2 in, 2 out]
            n820 = property on="ComTestResult" class="Bool (strict)"() -> ("Value"=w2089:bool)  [unwired: 2 in, 2 out]
            n821 = property on="UUT" class="DigNum (strict)"() -> ("Value"=w2087:u8)  [unwired: 2 in, 2 out]
            n822 = property on="Current SN" class="DigNum (strict)"(error in=w2109) -> ("Value"=w2108:i32)  [unwired: 1 in, 2 out]
            n823 = case shown="95" w2087 {
              tunnel: [w2152 w2155] -> w2103
              tunnel: [w2152 w2154] -> w2094
              tunnel: [w2152 w2153] -> w2093
              frame 47, 63, Default {
                w2152 = TRUE ("Value")
              }
              frame 95 {
                n824 = property on="AuxiOFFResult" class="Bool (strict)"() -> ("Value"=w2153:bool)  [unwired: 2 in, 2 out]
                n825 = property on="AuxiONResult" class="Bool (strict)"() -> ("Value"=w2154:bool)  [unwired: 2 in, 2 out]
                n826 = property on="TempControlResult" class="Bool (strict)"() -> ("Value"=w2155:bool)  [unwired: 2 in, 2 out]
              }
            }
            n827 = property on="VisualInspectionResult" class="Bool (strict)"() -> ("Value"=w2096:bool)  [unwired: 2 in, 2 out]
            n828 = property on="SensCalResult" class="Bool (strict)"() -> ("Value"=w2095:bool)  [unwired: 2 in, 2 out]
            n829 = Equal To 0?(x=w2108) -> (x = 0?=w2105:bool)
            n830 = Equal?(x=w2108, y=-1) -> (x = y?=w2106:bool)
            n831 = Or(x=w2106, y=w2105) -> (x .or. y?=w2086:bool)
            n832 = property on="BurnDC" class="Bool (strict)"() -> ("Value"=w2097:bool)  [unwired: 2 in, 2 out]
            n833 = property on="BurnTemp" class="Bool (strict)"() -> ("Value"=w2098:bool)  [unwired: 2 in, 2 out]
            n834 = property on="BurnSpeed" class="Bool (strict)"() -> ("Value"=w2099:bool)  [unwired: 2 in, 2 out]
            n835 = property on="BurnResult" class="Bool (strict)"() -> ("Value"=w2100:bool)  [unwired: 2 in, 2 out]
            n836 = property on="StopTimeResult" class="Bool (strict)"() -> ("Value"=w2101:bool)  [unwired: 2 in, 2 out]
            n837 = property on="MotorTempResult" class="Bool (strict)"() -> ("Value"=w2102:bool)  [unwired: 2 in, 2 out]
            n838 = property on="Automation" class="Bool (strict)"() -> ("Value"=w2079:bool)  [unwired: 2 in, 2 out]
            n839 = Build Array(w2089, w2090, w2091, w2092, w2093, w2094, w2095, w2096, w2097, w2098, w2099, w2100, w2101, w2102, w2103) -> (w2088:bool[])
            n840 = And Array Elements(Boolean array=w2088) -> (logical AND=w2104:bool)
            n841 = Not(x=w2104) -> (.not. x?=w2085:bool)
            n842 = Select(t=w2085, s=w2079, f=w2081) -> (s? t:f=w2084:bool)
            n843 = And(x=w2086, y=w2084) -> (x .and. y?=w2082:bool)
            n844 = case shown="True" w2082 {
              tunnel: w2110 -> [_ w2145]
              tunnel: w2083 -> [_ w2138]
              tunnel: w2079 -> [w2118 _]
              tunnel: [w2117 w2129] -> w2080
              frame False {
                n845 = case shown="True" w2118 {
                  tunnel: [w2119 w2120] -> w2117
                  frame False {
                    n846 = call "Display Message to User9"() -> ("error out"=w2119:errorcluster)  [unwired: 10 in, 1 out]
                  }
                  frame True {
                    n847 = call "Display Message to User3"() -> ("error out"=w2120:errorcluster)  [unwired: 10 in, 1 out]
                  }
                }
              }
              frame True {
                w2137 = FALSE ("SetSN")
                n848 = property on="Next SN" class="DigNum (strict)"() -> ("Value"=w2134:i32)  [unwired: 2 in, 2 out]
                n849 = property on="VISA Tester" class="VISAName"() -> ("Value"=w2127:refnum<visa-resource-name>)  [unwired: 2 in, 2 out]
                n850 = call "TesterOption (SubVI).vi"("2 Options"=FALSE, "On/Off"=FALSE, "Tester Option"=T11."Venable", "VISA Refnum in"=w2127) -> ("error out"=w2122:errorcluster)  [unwired: 6 in, 1 out]
                n851 = call <vilib>:"Clear Errors.vi"("error in (no error)"=w2122) -> ("error out"=w2123:errorcluster)  [unwired: 5 in, 1 out]
                n852 = Number To Decimal String(number=w2134) -> (decimal integer string=w2121:string)  [unwired: 1 in]
                "UUT SN Report" <- w2121
                n853 = Search and Replace String(input string="EP=1\r\nSN=0\r\n" ("write buffer"), search string="0", replace string=w2121) -> (result string=w2140:string)  [unwired: 5 in, 3 out]
                n854 = call "SerialMarvinSendGet.vi"("error in (no error)"=w2123, "Clear Log"=FALSE, "write buffer"=w2140, "VISA resource name"=w2138) -> ("error out"=w2128:errorcluster)  [unwired: 6 in, 1 out]
                n855 = property on="UUT" class="DigNum (strict)"(error in=w2128) -> ("Value"=w2146:u8)  [unwired: 1 in, 2 out]
                n856 = case shown="47, 63, Default" w2146 {
                  tunnel: ["AHU Serial Number" ("key") "EBAY Serial Number" ("key")] -> w2149
                  frame 47, 63, Default {
                  }
                  frame 95 {
                  }
                }
                n857 = call <vilib>:"Open Config Data.vi"("create file if necessary (T)"=FALSE, "configuration file path"=w2145) -> ("error out"=w2143:errorcluster, "refnum"=w2144:T24)  [unwired: 1 in, 7 out]
                n858 = call-poly <vilib>:"Write Key.vi"("section"="Marvin", "error in (no error)"=w2143, "value"=w2121, "key"=w2149, "refnum"=w2144) -> ("error out"=w2132:errorcluster, "refnum out"=w2131:T24)  [unwired: 4 in, 1 out]
                n859 = call <vilib>:"Close Config Data.vi"("error in (no error)"=w2132, "refnum"=w2131) -> ("error out"=w2130:errorcluster)  [unwired: 8 in, 1 out]
                n860 = property on="SetSN" class="Bool (strict)"(error in=w2130, "Value"=w2137) -> (error out=w2136:errorcluster)  [unwired: 1 in, 1 out]
                n861 = property on="Automation" class="Bool (strict)"(error in=w2136, "Value"=w2137) -> (error out=w2135:errorcluster)  [unwired: 1 in, 1 out]
                n862 = Increment(x=w2134) -> (x+1=w2133:i32)
                n863 = property on="Next SN" class="DigNum (strict)"(error in=w2135, "Value"=w2133) -> (error out=w2129:errorcluster)  [unwired: 1 in, 1 out]
              }
            }
            n864 = case shown="True" w2079 {
              tunnel: w2080 -> [_ _]
              frame False {
              }
              frame True {
                w2116 = TRUE ("Value (Signaling)")
                n865 = property on="Report" class="Bool (strict)"("Val(Sgnl)"=w2116, "Value"=w2116) -> ()  [unwired: 2 in, 2 out]
              }
            }
          }
          event "ATR": Mouse Enter {
            n866 = event-data() -> ()  [unwired: 1 in, 4 out]
            n867 = call-poly <vilib>:"Set Cursor.vi"("error in (no error)"=w2162, "icon"=u16 1) -> ("error out"=w2163:errorcluster)  [unwired: 8 in, 1 out]
          }
          event "ATR": Mouse Leave {
            n868 = event-data() -> ()  [unwired: 1 in, 4 out]
            n869 = call-poly <vilib>:"Set Cursor.vi"("error in (no error)"=w2172, "icon"=u16 0) -> ("error out"=w2170:errorcluster)  [unwired: 8 in, 1 out]
          }
          event "ATR": Mouse Down? {
            n870 = event-data() -> ("Coords"=w2187:T28)  [unwired: 1 in, 4 out]
            n871 = invoke on="ATR" class="Tbl (strict)" method="Point To Row Column"("Point"=w2187) -> ("InBounds"=w2183:bool, "CellPosition"=w2182:T19)  [unwired: 5 in, 4 out]
            n872 = Greater Than 0?(x=w2182) -> (x > 0?=w2186:cluster{"Row":bool, "Column":bool})
            n873 = Cluster To Array(cluster=w2186) -> (array=w2185:bool[])
            n874 = Or Array Elements(Boolean array=w2185) -> (logical OR=w2184:bool)
            n875 = Or(x=w2183, y=w2184) -> (x .or. y?=w2181:bool)
            n876 = event-data("Discard?"=w2181) -> ()  [unwired: 1 in, 1 out]
          }
          event Panel Close? {
            w2189 = TRUE ("Stop Button")
            n877 = event-data() -> ("VIRef"=w2191:refnum<vi>)  [unwired: 1 in, 3 out]
            n878 = Close Reference(reference=w2191) -> ()  [unwired: 1 in, 1 out]
            n879 = property on="Stop Button" class="Bool (strict)"("Value"=w2189, "Val(Sgnl)"=w2189) -> ()  [unwired: 2 in, 2 out]
            n880 = event-data("Discard?"=TRUE) -> ()  [unwired: 1 in, 1 out]
          }
          event "Start": Value Change {
            w2199 = T16 [] items=["Auxiliary", "Temp Sens Cal", "Com Test", "Enable Test", "Speed Command", "Stop Time", "Temp Control", "Burn in", "Visual Inspec", "Empty"]
            n881 = event-data() -> ()  [unwired: 1 in, 2 out]
            n882 = property on="UUT" class="Str"(error in=w2212) -> ("Value"=w2211:string)  [unwired: 1 in, 2 out]
            n883 = while {
              tunnel: w2211 -> [w2228]
              tunnel: [w2227] -> w2206
              tunnel: [w2226] -> w2205
              shift-right: [w2219] -> _
              shift-left: enum16{"Stop", "Tests", "Bit test", "Start"}."Start" -> [w2225]
              tunnel: w2200 -> [w2224]
              tunnel: w2199 -> [w2218]
              stop <- w2217 stop-if-true
              n884 = control-ref of="Pannel User Message"() -> (w2223:refnum<vi>)
              n885 = control-ref of="Stop Button"() -> (w2222:refnum<vi>)
              n886 = control-ref of="Motor Speed RPM"() -> (w2220:refnum<vi>)
              n887 = control-ref of="Stop Burn-in"() -> (w2221:refnum<vi>)
              n888 = property on="Status" class="Bool (strict)"() -> (error out=w2214:errorcluster, "Value"=w2216:bool)  [unwired: 2 in, 1 out]
              n889 = property on="VISA Tester" class="VISAName"() -> ("Value"=w2215:refnum<visa-resource-name>)  [unwired: 2 in, 2 out]
              n890 = case shown="\"Tests\"" w2225 {
                tunnel: w2228 -> [_ w2243 w2353 _]
                tunnel: [w2233 w2242 w2388 w2491] -> w2227
                tunnel: [w2229 w2241 w2351 w2490] -> w2226
                tunnel: w2224 -> [_ _ w2369 w2496]
                tunnel: w2223 -> [_ _ _ w2495]
                tunnel: w2222 -> [_ _ _ w2494]
                tunnel: w2221 -> [_ _ _ w2493]
                tunnel: w2220 -> [_ _ _ w2492]
                tunnel: [w2232 w2240 w2356 w2486] -> w2219
                tunnel: w2218 -> [w2233 _ w2388 w2491]
                tunnel: [w2231 w2239 FALSE FALSE] -> w2217
                tunnel: w2216 -> [_ _ _ w2488]
                tunnel: w2215 -> [_ _ w2370 _]
                tunnel: w2214 -> [w2229 _ _ _]
                frame "Stop", Default {
                  n891 = property on="Start" class="Bool (strict)"(error in=w2229, "Value"=FALSE ("Start")) -> ()  [unwired: 1 in, 2 out]
                  n892 = flat-sequence {
                    tunnel: [enum16{"Stop", "Tests", "Bit test", "Start"}."Stop"] -> w2232
                    tunnel: w2229 -> [_]
                    tunnel: [TRUE] -> w2231
                    frame #0 {
                    }
                  }
                }
                frame "Tests" {
                  w2236 = FALSE ("Stop Burn-in")
                  w2238 = T18."Disabled and Grayed Out" ("Disabled")
                  n893 = case shown="\"AHU\", Default" w2243 {
                    tunnel: [w2258 w2307] -> w2242
                    tunnel: [w2257 w2306] -> w2241
                    tunnel: [w2246 w2294] -> w2237
                    frame "AHU", Default {
                      n894 = call "Load Program Process AHU.vi"() -> ("Speed Command Test"=w2251:bool, "Enable Test"=w2252:bool, "Burn-in Test"=w2249:bool, "Auxiliary"=w2247:bool, "Temperature Sensor Calibration Test"=w2254:bool, "Communication Test"=w2253:bool, "Stop Time Test"=w2250:bool, "Visual Inspection"=w2248:bool, "OK"=w2255:bool, "Automation"=w2246:bool, "error out"=w2257:errorcluster)  [unwired: 8 in, 9 out]
                      n895 = Or(x=w2255, y=w2246) -> (x .or. y?=w2256:bool)
                      n896 = case shown="True" w2256 {
                        tunnel: [w2259 w2269] -> w2258
                        tunnel: w2246 -> [_ w2268]
                        tunnel: w2254 -> [_ w2267]
                        tunnel: w2253 -> [_ w2266]
                        tunnel: w2252 -> [_ w2265]
                        tunnel: w2251 -> [_ w2264]
                        tunnel: w2250 -> [_ w2263]
                        tunnel: w2249 -> [_ w2262]
                        tunnel: w2248 -> [_ w2261]
                        tunnel: w2247 -> [_ w2260]
                        frame False {
                          w2259 = T16 [] items=["Auxiliary", "Temp Sens Cal", "Com Test", "Enable Test", "Speed Command", "Stop Time", "Temp Control", "Burn in", "Visual Inspec", "Empty"]
                        }
                        frame True {
                          n897 = case shown="False" w2268 {
                            tunnel: [w2292 w2293] -> w2269
                            tunnel: w2267 -> [w2274 _]
                            tunnel: w2266 -> [w2273 _]
                            tunnel: w2265 -> [w2275 _]
                            tunnel: w2264 -> [w2272 _]
                            tunnel: w2263 -> [w2271 _]
                            tunnel: w2262 -> [w2285 _]
                            tunnel: w2261 -> [w2270 _]
                            tunnel: w2260 -> [_ _]
                            frame False {
                              w2278 = T20."Empty" ("f")
                              n898 = Select(t=T20."Com Test" ("f"), s=w2273, f=w2278) -> (s? t:f=w2284:T20)
                              n899 = Select(t=T20."Temp Sens Cal" ("f"), s=w2274, f=w2278) -> (s? t:f=w2283:T20)
                              n900 = Select(t=T20."Stop Time" ("f"), s=w2271, f=w2278) -> (s? t:f=w2282:T20)
                              n901 = Select(t=T20."Enable Test" ("f"), s=w2275, f=w2278) -> (s? t:f=w2281:T20)
                              n902 = Select(t=T20."Speed Command" ("f"), s=w2272, f=w2278) -> (s? t:f=w2280:T20)
                              n903 = Select(t=T20."Burn in" ("f"), s=w2285, f=w2278) -> (s? t:f=w2279:T20)
                              n904 = Select(t=T20."Visual Inspec" ("f"), s=w2270, f=w2278) -> (s? t:f=w2276:T20)
                              n905 = Build Array(w2284, w2283, w2282, w2281, w2280, w2279, w2276) -> (w2292:T16)
                            }
                            frame True {
                              w2293 = T16 [enum."Com Test", enum."Temp Sens Cal", enum."Stop Time", enum."Enable Test", enum."Speed Command", enum."Burn in", enum."Visual Inspec"] items=["Auxiliary", "Temp Sens Cal", "Com Test", "Enable Test", "Speed Command", "Stop Time", "Temp Control", "Burn in", "Visual Inspec", "Empty"]
                            }
                          }
                        }
                      }
                    }
                    frame "EBAY" {
                      n906 = call "Load Program Process EBAY.vi"() -> ("Speed Command Test"=w2300:bool, "Enable Test"=w2301:bool, "Burn-in Test"=w2298:bool, "Temperature Control Algorithm Test"=w2297:bool, "Auxiliary"=w2295:bool, "Temperature Sensor Calibration Test"=w2303:bool, "Communication Test"=w2302:bool, "Stop Time Test"=w2299:bool, "Visual Inspection"=w2296:bool, "OK"=w2304:bool, "Automation"=w2294:bool, "error out"=w2306:errorcluster)  [unwired: 8 in, 8 out]
                      n907 = Or(x=w2304, y=w2294) -> (x .or. y?=w2305:bool)
                      n908 = case shown="True" w2305 {
                        tunnel: [w2308 w2319] -> w2307
                        tunnel: w2294 -> [_ w2318]
                        tunnel: w2303 -> [_ w2317]
                        tunnel: w2302 -> [_ w2316]
                        tunnel: w2301 -> [_ w2315]
                        tunnel: w2300 -> [_ w2314]
                        tunnel: w2299 -> [_ w2313]
                        tunnel: w2298 -> [_ w2312]
                        tunnel: w2297 -> [_ w2311]
                        tunnel: w2296 -> [_ w2310]
                        tunnel: w2295 -> [_ w2309]
                        frame False {
                          w2308 = T16 [] items=["Auxiliary", "Temp Sens Cal", "Com Test", "Enable Test", "Speed Command", "Stop Time", "Temp Control", "Burn in", "Visual Inspec", "Empty"]
                        }
                        frame True {
                          n909 = case shown="False" w2318 {
                            tunnel: [w2348 w2349] -> w2319
                            tunnel: w2317 -> [w2324 _]
                            tunnel: w2316 -> [w2323 _]
                            tunnel: w2315 -> [w2322 _]
                            tunnel: w2314 -> [w2321 _]
                            tunnel: w2313 -> [w2320 _]
                            tunnel: w2312 -> [w2326 _]
                            tunnel: w2311 -> [w2325 _]
                            tunnel: w2310 -> [w2339 _]
                            tunnel: w2309 -> [w2330 _]
                            frame False {
                              w2328 = T20."Empty" ("f")
                              n910 = Select(t=T20."Com Test" ("f"), s=w2323, f=w2328) -> (s? t:f=w2338:T20)
                              n911 = Select(t=T20."Temp Sens Cal" ("f"), s=w2324, f=w2328) -> (s? t:f=w2337:T20)
                              n912 = Select(t=T20."Stop Time" ("f"), s=w2320, f=w2328) -> (s? t:f=w2336:T20)
                              n913 = Select(t=T20."Enable Test" ("f"), s=w2322, f=w2328) -> (s? t:f=w2335:T20)
                              n914 = Select(t=T20."Speed Command" ("f"), s=w2321, f=w2328) -> (s? t:f=w2334:T20)
                              n915 = Select(t=T20."Temp Control" ("f"), s=w2325, f=w2328) -> (s? t:f=w2333:T20)
                              n916 = Select(t=T20."Burn in" ("f"), s=w2326, f=w2328) -> (s? t:f=w2332:T20)
                              n917 = Select(t=T20."Visual Inspec" ("f"), s=w2339, f=w2328) -> (s? t:f=w2331:T20)
                              n918 = Select(t=T20."Auxiliary" ("f"), s=w2330, f=w2328) -> (s? t:f=w2327:T20)
                              n919 = Build Array(w2338, w2337, w2336, w2335, w2334, w2333, w2332, w2327, w2331) -> (w2348:T16)
                            }
                            frame True {
                              w2349 = T16 [enum."Com Test", enum."Temp Sens Cal", enum."Stop Time", enum."Enable Test", enum."Speed Command", enum."Temp Control", enum."Burn in", enum."Auxiliary", enum."Visual Inspec"] items=["Auxiliary", "Temp Sens Cal", "Com Test", "Enable Test", "Speed Command", "Stop Time", "Temp Control", "Burn in", "Visual Inspec", "Empty"]
                            }
                          }
                        }
                      }
                    }
                  }
                  "Automation" <- w2237
                  n920 = flat-sequence {
                    tunnel: [enum16{"Stop", "Tests", "Bit test", "Start"}."Tests"] -> w2240
                    tunnel: [TRUE] -> w2239
                    frame #0 {
                    }
                  }
                  n921 = property on="Stop Button" class="Bool (strict)"("Value"=w2236) -> ()  [unwired: 2 in, 2 out]
                  n922 = property on="Stop Burn-in" class="Bool (strict)"("Value"=w2236) -> ()  [unwired: 2 in, 2 out]
                  n923 = property on="Start" class="Bool (strict)"("DisabledEnum"=w2238) -> ()  [unwired: 2 in, 2 out]
                  n924 = property on="Report" class="Bool (strict)"("DisabledEnum"=w2238) -> ()  [unwired: 2 in, 2 out]
                }
                frame "Bit test" {
                  # "Stop"
                  n925 = call "SerialMarvinSendGet.vi"("write buffer"="TA[1]\r\n", "VISA resource name"=w2369) -> ("error out"=w2382:errorcluster, "read buffer"=w2385:string)  [unwired: 8 in]
                  n926 = Fract/Exp String To Number(string=w2385) -> (number=w2384:dbl)  [unwired: 3 in, 1 out]
                  n927 = Less Or Equal?(x=w2384, y=100.0) -> (x <= y?=w2367:bool)
                  n928 = call "TesterOption (SubVI).vi"("On/Off 2"=FALSE, "Tester Option 2"=T11."Venable", "2 Options"=TRUE, "error in (no error)"=w2382, "On/Off"=TRUE, "Tester Option"=T11."25C", "VISA Refnum in"=w2370) -> ("error out"=w2372:errorcluster)  [unwired: 3 in, 1 out]
                  n929 = call "Time Delay5"("error in (no error)"=w2372) -> ("error out"=w2371:errorcluster)  [unwired: 10 in]
                  n930 = call "SerialMarvinSendGet.vi"("error in (no error)"=w2371, "write buffer"="TA[2]\r\n", "VISA resource name"=w2369) -> ("error out"=w2368:errorcluster, "read buffer"=w2374:string)  [unwired: 7 in]
                  n931 = case shown="\"AHU\"" w2353 {
                    tunnel: w2370 -> [w2418 _ w2446]
                    tunnel: w2369 -> [_ _ w2449]
                    tunnel: w2368 -> [w2419 w2437 w2448]
                    tunnel: [w2412 w2437 w2444] -> w2355
                    tunnel: [w2409 "" w2439] -> w2362
                    tunnel: [w2408 bool[] [] w2438] -> w2360
                    frame "AHU" {
                      n932 = call "TesterOption (SubVI).vi"("On/Off 2"=FALSE, "Tester Option 2"=T11."Venable", "2 Options"=TRUE, "error in (no error)"=w2419, "On/Off"=TRUE, "Tester Option"=T11."K17", "VISA Refnum in"=w2418) -> ("error out"=w2421:errorcluster)  [unwired: 3 in, 1 out]
                      n933 = call "Time Delay7"("error in (no error)"=w2421) -> ("error out"=w2420:errorcluster)  [unwired: 10 in]
                      n934 = call "GetADCTester (SubVI).vi"("error in (no error)"=w2420, "GetADCTester"=T13."Current", "TimeToGet"=5, "VISA Refnum in"=w2418) -> ("error out"=w2412:errorcluster, "ADCValOutput Single"=w2414:dbl)  [unwired: 5 in, 1 out]
                      n935 = Less Or Equal?(x=w2414, y=50.0) -> (x <= y?=w2413:bool)
                      n936 = Build Array(w2413) -> (w2408:bool[])
                      n937 = for {
                        tunnel: w2408 -> [w2434] mode=indexing
                        tunnel: string[] ["CURRENT OPERATION FAILED!"] -> [w2430] mode=indexing
                        shift-right: [w2432] -> w2409
                        shift-left: "" -> [w2431]
                        n938 = Concatenate Strings(w2430, "  TEST FAILED!" ("string"), "\r\n") -> (w2427:string)
                        n939 = Select(t=w2427, s=w2434, f=w2431) -> (s? t:f=w2433:string)
                        n940 = Concatenate Strings(w2431, w2433) -> (w2432:string)
                      }
                    }
                    frame Default {
                    }
                    frame "EBAY" {
                      w2447 = T29 [enum."Fan", enum."Current"] items=["Term1", "Term2", "Current", "Fan", "TempCPU"]
                      n941 = call "TesterOption (SubVI).vi"("On/Off 2"=FALSE, "Tester Option 2"=T11."Venable", "2 Options"=TRUE, "error in (no error)"=w2448, "On/Off"=TRUE, "Tester Option"=T11."K17", "VISA Refnum in"=w2446) -> ("error out"=w2451:errorcluster)  [unwired: 3 in, 1 out]
                      n942 = call "Time Delay6"("error in (no error)"=w2451) -> ("error out"=w2450:errorcluster)  [unwired: 10 in]
                      n943 = call "SerialMarvinSendGet.vi"("error in (no error)"=w2450, "write buffer"="TA[3]\r\n", "VISA resource name"=w2449) -> ("error out"=w2445:errorcluster, "read buffer"=w2453:string)  [unwired: 7 in]
                      n944 = Fract/Exp String To Number(string=w2453) -> (number=w2454:dbl)  [unwired: 3 in, 1 out]
                      n945 = for {
                        tunnel: w2447 -> [w2478] mode=indexing
                        tunnel: w2446 -> [w2477]
                        tunnel: w2445 -> [w2475]
                        tunnel: [w2474] -> w2444
                        tunnel: [w2471] -> w2442 mode=indexing
                        i -> [w2472]
                        n946 = call "GetADCTester (SubVI).vi"("error in (no error)"=w2475, "GetADCTester"=w2478, "TimeToGet"=0, "VISA Refnum in"=w2477) -> ("error out"=w2474:errorcluster, "ADCValOutput Single"=w2473:dbl)  [unwired: 5 in, 1 out]
                        n947 = case shown="1" w2472 {
                          tunnel: w2473 -> [w2481 w2484 _]
                          tunnel: [w2479 w2482 FALSE] -> w2471
                          frame 1 {
                            n948 = Less Or Equal?(x=w2481, y=50.0) -> (x <= y?=w2479:bool)
                          }
                          frame 0 {
                            n949 = Greater Or Equal?(x=w2484, y=2200.0) -> (x >= y?=w2482:bool)
                          }
                          frame Default {
                          }
                        }
                      }
                      n950 = Less Or Equal?(x=w2454, y=100.0) -> (x <= y?=w2443:bool)
                      n951 = Build Array (concatenate)(w2443, w2442) -> (w2438:bool[])
                      n952 = for {
                        tunnel: w2438 -> [w2461] mode=indexing
                        tunnel: string[] ["TA[3] OPERATION FAILED!", "EBAY FAN OPERATION FAILED!", "CURRENT OPERATION FAILED!"] -> [w2464] mode=indexing
                        shift-right: [w2466] -> w2439
                        shift-left: "" -> [w2465]
                        n953 = Concatenate Strings(w2464, "\r\n") -> (w2462:string)
                        n954 = case shown="False" w2461 {
                          tunnel: [w2469 w2470] -> w2466
                          tunnel: w2465 -> [w2468 w2470]
                          tunnel: w2462 -> [w2467 _]
                          frame False {
                            n955 = Concatenate Strings(w2468, w2467) -> (w2469:string)
                          }
                          frame True {
                          }
                        }
                      }
                    }
                  }
                  n956 = Fract/Exp String To Number(string=w2374) -> (number=w2375:dbl)  [unwired: 3 in, 1 out]
                  n957 = Less Or Equal?(x=w2375, y=100.0) -> (x <= y?=w2366:bool)
                  n958 = Build Array(w2367, w2366) -> (w2361:bool[])
                  n959 = for {
                    tunnel: w2361 -> [w2397] mode=indexing
                    tunnel: string[] ["TA[1] OPERATION FAILED!", "TA[2] OPERATION FAILED!"] -> [w2401] mode=indexing
                    shift-right: [w2403] -> w2363
                    shift-left: "" -> [w2402]
                    tunnel: w2355 -> [w2398]
                    tunnel: [w2398] -> w2354
                    n960 = Concatenate Strings(w2401, "\r\n") -> (w2399:string)
                    n961 = case shown="False" w2397 {
                      tunnel: [w2406 w2407] -> w2403
                      tunnel: w2402 -> [w2405 w2407]
                      tunnel: w2399 -> [w2404 _]
                      frame False {
                        n962 = Concatenate Strings(w2405, w2404) -> (w2406:string)
                      }
                      frame True {
                      }
                    }
                  }
                  n963 = Build Array (concatenate)(w2361, w2360) -> (w2359:bool[])
                  n964 = And Array Elements(Boolean array=w2359) -> (logical AND=w2350:bool)
                  n965 = case shown="False" w2350 {
                    tunnel: w2363 -> [w2395 _]
                    tunnel: w2362 -> [w2394 _]
                    tunnel: w2354 -> [w2392 w2396]
                    tunnel: [w2392 w2396] -> w2352
                    frame False {
                      n966 = Concatenate Strings(w2395, w2394) -> (w2393:string)
                      n967 = One Button Dialog(message=w2393) -> ()  [unwired: 1 in, 1 out]
                    }
                    frame True {
                    }
                  }
                  n968 = case shown="True" w2350 {
                    tunnel: w2352 -> [w2390 w2391]
                    tunnel: [w2389 w2391] -> w2351
                    frame False {
                      n969 = call "Display Message to User6"("error in (no error)"=w2390) -> ("error out"=w2389:errorcluster)  [unwired: 9 in, 1 out]
                    }
                    frame True {
                    }
                  }
                  n970 = Select(t=enum16{"Stop", "Tests", "Bit test", "Start"}."Tests", s=w2350, f=enum16{"Stop", "Tests", "Bit test", "Start"}."Tests") -> (s? t:f=w2356:enum16{"Stop", "Tests", "Bit test", "Start"})
                }
                frame "Start" {
                  n971 = case shown="True" w2488 {
                    tunnel: w2496 -> [_ w2520]
                    tunnel: w2495 -> [_ w2511]
                    tunnel: w2494 -> [_ w2507]
                    tunnel: w2493 -> [_ w2505]
                    tunnel: w2492 -> [_ w2504]
                    tunnel: [FALSE w2503] -> w2487
                    tunnel: [w2500 w2502] -> w2490
                    frame False {
                      n972 = call "Display Message to User5"() -> ("error out"=w2500:errorcluster)  [unwired: 10 in, 1 out]
                    }
                    frame True {
                      n973 = property on="VISA Tester" class="VISAName"() -> (error out=w2518:errorcluster, "Value"=w2517:refnum<visa-resource-name>)  [unwired: 2 in, 1 out]
                      n974 = call "TesterOption (SubVI).vi"("2 Options"=FALSE, "error in (no error)"=w2518, "On/Off"=FALSE, "Tester Option"=T11."Venable", "VISA Refnum in"=w2517) -> ("error out"=w2513:errorcluster)  [unwired: 5 in, 1 out]
                      n975 = call "Write panel message (SubVI).vi"("Stop BurnIn"=w2505, 4:"rpm"=w2504, 5:"rpm"=FALSE ("rpm"), "PrintTime"=FALSE, "Stop"=w2507, "error in (no error)"=w2513, "Time to wait"=3.0, "Strin"="TESTER BIT TEST OPERATION IN PROCESS", "String in"=w2511) -> ("error out"=w2512:errorcluster)  [unwired: 2 in]
                      n976 = property on="UUT SoftwareVer" class="Str"() -> ("Value"=w2501:string)  [unwired: 2 in, 2 out]
                      n977 = call "SerialMarvinSendGet.vi"("error in (no error)"=w2512, "write buffer"="VR\r\n", "VISA resource name"=w2520) -> ("error out"=w2502:errorcluster, "read buffer"=w2519:string)  [unwired: 7 in]
                      n978 = Equal?(x=w2519, y=w2501) -> (x = y?=w2503:bool)
                    }
                  }
                  n979 = case shown="True" w2487 {
                    tunnel: [enum16{"Stop", "Tests", "Bit test", "Start"}."Stop" enum16{"Stop", "Tests", "Bit test", "Start"}."Bit test"] -> w2486
                    frame False {
                      n980 = call "Display Message to User4"() -> ()  [unwired: 10 in, 2 out]
                    }
                    frame True {
                    }
                  }
                }
              }
            }
            n981 = Bundle By Name(cluster=T8 {"VISA"="COM1", "Array Test"=[]}, "VISA"=w2200, "Array Test"=w2206) -> (w2202:T8)
            n982 = Enqueue Element(queue=w2208, element=w2202, error in (no error)=w2205) -> (queue out=w2203:refnum<queue>, error out=w2204:errorcluster)  [unwired: 2 out]
          }
          event "Report", "Stop Button": Value Change {
            w2550 = "Marvin" ("section")
            n983 = event-data() -> ("CtlRef"=w2535:refnum<vi>)  [unwired: 1 in]
            n984 = local read "UUT"() -> (w2546:string)
            n985 = call <vilib>:"Application Directory.vi"() -> ("Application Directory"=w2578:path)
            n986 = Build Path(base path=w2578, name or relative path="Reports") -> (appended path=w2581:path)
            n987 = property on="Status" class="Bool (strict)"() -> ("Value"=w2540:bool)  [unwired: 2 in, 2 out]
            n988 = case shown="\"EBAY\", Default" w2546 {
              tunnel: ["REV EBAY" ("key") "REV AHU" ("key")] -> w2548
              frame "EBAY", Default {
              }
              frame "AHU" {
              }
            }
            n989 = call <vilib>:"Check if File or Folder Exists.vi"("path"=w2581) -> ("error out"=w2579:errorcluster, "file or folder exists?"=w2582:bool, "dup path"=w2580:path)  [unwired: 8 in]
            n990 = case shown="False" w2582 {
              tunnel: w2579 -> [w2637 w2638]
              tunnel: w2580 -> [w2636 w2639]
              tunnel: [w2635 w2639] -> w2587
              tunnel: [w2634 w2638] -> w2584
              frame False {
                n991 = Create Folder(path (use dialog)=w2636, error in=w2637) -> (created path=w2635:path, error out=w2634:errorcluster)  [unwired: 1 in, 1 out]
              }
              frame True {
              }
            }
            n992 = case shown="True" w2540 {
              tunnel: [w2594 w2603] -> w2567
              tunnel: [w2594 w2602] -> w2545
              tunnel: w2539 -> [_ w2596]
              tunnel: [w2594 w2595] -> w2536
              tunnel: [w2594 w2598] -> w2538
              tunnel: [w2594 w2597] -> w2529
              frame False {
                w2594 = "N_A" ("read buffer")
                n993 = disable-structure shown="Disabled" {
                  frame Disabled {
                    n994 = call "Display Message to User7"() -> ()  [unwired: 10 in, 2 out]
                  }
                  frame Enabled {
                  }
                }
              }
              frame True {
                n995 = property on="UUT SN Report" class="Str"() -> ("Value"=w2595:string)  [unwired: 2 in, 2 out]
                n996 = call "SerialMarvinSendGet.vi"("write buffer"="VR\r\n", "VISA resource name"=w2596) -> ("error out"=w2599:errorcluster, "read buffer"=w2598:string)  [unwired: 8 in]
                n997 = property on="UUT" class="DigNum (strict)"(error in=w2599) -> ("Value"=w2601:u8)  [unwired: 1 in, 2 out]
                n998 = case shown="95, Default" w2601 {
                  tunnel: ["414-8005_95_EBAY_" " 413-8005_47_AHU" " 413-8005_63_AHU"] -> w2603
                  tunnel: ["EBAY 414-8005           " "AHU-L (47) 413-8005-1" "AHU-R (63) 413-8005-2"] -> w2602
                  tunnel: ["414-8005-95" " 413-8005-1-47" " 413-8005-2-63"] -> w2597
                  frame 95, Default {
                  }
                  frame 47 {
                  }
                  frame 63 {
                  }
                }
              }
            }
            n999 = Get Date/Time String(want seconds? (F)=TRUE) -> (date string=w2583:string)  [unwired: 2 in, 1 out]
            n1000 = call <vilib>:"Open Config Data.vi"("create file if necessary (T)"=FALSE, "configuration file path"=w2542) -> ("refnum"=w2557:T24)  [unwired: 1 in, 8 out]
            n1001 = property on="Logger Path" class="Path"(error in=w2584, "Value"=w2587, "StartPath"=w2587) -> (error out=w2585:errorcluster)  [unwired: 1 in, 1 out]
            n1002 = Search and Replace String(replace all?=TRUE ("replace all? (F)"), input string=w2583, search string="/") -> (result string=w2564:string)  [unwired: 5 in, 3 out]
            n1003 = call-poly <vilib>:"Read Key.vi"("section"=w2550, "key"=w2548, "refnum"=w2557) -> ("error out"=w2552:errorcluster, "value"=w2555:string, "refnum out"=w2554:T24)  [unwired: 5 in, 1 out]
            n1004 = property on="Logger Path" class="Path"(error in=w2585) -> (error out=w2560:errorcluster, "StartPath"=w2563:path)  [unwired: 1 in, 1 out]
            n1005 = call-poly <vilib>:"Read Key.vi"("section"=w2550, "error in (no error)"=w2552, "key"="Tester Software Ver", "refnum"=w2554) -> ("error out"=w2549:errorcluster, "value"=w2547:string, "refnum out"=w2553:T24)  [unwired: 4 in, 1 out]
            n1006 = Concatenate Strings("ATR" ("string"), w2567, w2536, "_", w2564, ".docx" ("string")) -> (w2561:string)
            n1007 = call <vilib>:"Close Config Data.vi"("error in (no error)"=w2549, "refnum"=w2553) -> ()  [unwired: 8 in, 2 out]
            n1008 = Build Path(base path=w2563, name or relative path=w2561) -> (appended path=w2562:path)
            n1009 = call "HeaderuRayon.vi"("Tester Software Ver"=w2547, "UUTHeader"=w2546, "UUT"=w2545, "S/N"=w2536, "VR"=w2538, "Oper."=w2537) -> ("HEADER1"=w2588:string)
            n1010 = Concatenate Strings("  Rev-" ("string"), w2555) -> (w2541:string)
            n1011 = while {
              tunnel: w2561 -> [w2619]
              tunnel: w2563 -> [w2616]
              shift-right: [w2618] -> w2559
              shift-left: w2562 -> [w2617]
              shift-right: [w2614] -> w2543
              shift-left: w2544 -> [w2615]
              tunnel: w2560 -> [w2620]
              tunnel: [w2621] -> _
              stop <- w2613 continue-if-true
              n1012 = call <vilib>:"Check if File or Folder Exists.vi"("error in (no error)"=w2620, "path"=w2617) -> ("error out"=w2621:errorcluster, "file or folder exists?"=w2613:bool)  [unwired: 7 in, 1 out]
              n1013 = case shown="True" w2613 {
                tunnel: w2619 -> [_ w2633]
                tunnel: w2615 -> [_ w2625]
                tunnel: [w2623 w2630] -> w2618
                tunnel: w2617 -> [w2623 _]
                tunnel: w2616 -> [_ w2631]
                tunnel: [1 w2624] -> w2614
                frame False {
                }
                frame True {
                  w2626 = ".docx" ("search string")
                  n1014 = Search and Replace String(input string=w2633, search string=w2626) -> (result string=w2632:string)  [unwired: 6 in, 3 out]
                  n1015 = Number To Decimal String(number=w2625) -> (decimal integer string=w2628:string)  [unwired: 1 in]
                  n1016 = call <vilib>:"Space Constant.vi"() -> ("String"=w2627:string)
                  n1017 = Concatenate Strings(w2632, w2627, w2628, w2626) -> (w2629:string)
                  n1018 = Build Path(base path=w2631, name or relative path=w2629) -> (appended path=w2630:path)
                  n1019 = Increment(x=w2625) -> (x+1=w2624:i32)
                }
              }
            }
            n1020 = Open/Create/Replace File(file path (use dialog)=w2559, operation (0:open)=T22."create") -> (error out=w2573:errorcluster)  [unwired: 4 in, 2 out]
            n1021 = control-ref of="ATR"() -> (w2589:refnum<vi>)
            n1022 = property class="Tbl (strict)"(reference=w2589, error in=w2573) -> ("Value"=w2590:string[][])  [unwired: 2 out]
            n1023 = call "MarvinReport.vi"("HEADER1"=w2588, "ATR Or"=w2589, "Steps   pfull"=w2590, "Footer UUT"=w2529, "pageNum"=3, "FILE NAME"=w2561, "Report Folder"=w2559, "REV"=w2541, "Test-Conductor"=w2537) -> ("error out"=w2524:errorcluster)  [unwired: 5 in, 1 out]
            n1024 = call <vilib>:"Clear Errors.vi"("error in (no error)"=w2524) -> ("error out"=w2523:errorcluster)  [unwired: 5 in, 1 out]
            n1025 = property class="Bool (strict)"(reference=w2535, error in=w2523) -> ("BoolText.Text"=w2534:string)  [unwired: 2 out]
            n1026 = Equal?(x=w2534, y="Report") -> (x = y?=w2528:bool)
            n1027 = Select(t=T10."MainProgram", s=w2528, f=T10."Stop") -> (s? t:f=w2531:T10)
            n1028 = Select(t="Save Report...", s=w2528, f="Program Stopped...\r\nPlease turn OFF All Power sinks") -> (s? t:f=w2526:string)
            n1029 = property on="Report" class="Bool (strict)"(error in=w2523, "Value"=FALSE ("Report")) -> ()  [unwired: 1 in, 2 out]
            n1030 = property on="Pannel User Message" class="Str"("Value"=w2526) -> ()  [unwired: 2 in, 2 out]
          }
          event "Help Button": Value Change {
            n1031 = event-data() -> ()  [unwired: 1 in, 6 out]
            n1032 = vi-ref "Help.vi"() -> (w2649:refnum<vi>)
            n1033 = invoke class="VI" method="FP.Open"(reference=w2649, error in=w2647, "Activate"=TRUE ("Activate?"), "State"=T23."Standard") -> (error out=w2648:errorcluster)  [unwired: 1 in, 4 out]
            n1034 = call "Help.vi"("error in"=w2648) -> ("error out"=w2646:errorcluster)  [unwired: 7 in]
          }
          event "Serial Com": Value Change {
            n1035 = event-data() -> ()  [unwired: 1 in, 6 out]
            n1036 = property on="Serial Com" class="Bool"(error in=w2658, "Visible"=FALSE) -> (error out=w2662:errorcluster)  [unwired: 1 in, 1 out]
            n1037 = property on="VISA Marvin" class="VISAName"(error in=w2662, "Visible"=TRUE) -> (error out=w2659:errorcluster)  [unwired: 1 in, 1 out]
          }
          event "VISA Marvin": Value Change {
            n1038 = event-data() -> ()  [unwired: 1 in, 6 out]
            n1039 = control-ref of="This VI"() -> (w2674:refnum<vi>)
            n1040 = property on="Pannel User Message" class="Str"(error in=w2666, "Value"="Serial connection in process" ("Pannel User Message")) -> ()  [unwired: 1 in, 2 out]
            n1041 = call "Serial InitMarvin.vi"("error in (no error)"=w2666, "VI reference (current VI)"=w2674, "VISA Refnum in"="VISA Marvin") -> ("error out"=w2665:errorcluster, "Boolean"=w2663:bool)  [unwired: 7 in]
            n1042 = property on="VISA Marvin" class="VISAName"(error in=w2665, "Visible"=FALSE) -> (error out=w2677:errorcluster)  [unwired: 1 in, 1 out]
            n1043 = property on="Serial Com" class="Bool"(error in=w2677, "Visible"=TRUE) -> (error out=w2673:errorcluster)  [unwired: 1 in, 1 out]
            n1044 = case shown="True" w2663 {
              tunnel: w2673 -> [w2680 w2692]
              tunnel: "VISA Marvin" -> [w2681 w2689]
              tunnel: [w2681 w2688] -> w2668
              tunnel: [w2680 w2687] -> w2667
              frame False {
              }
              frame True {
                n1045 = call "SerialMarvinSendGet.vi"("error in (no error)"=w2692, "Clear Log"=FALSE, "write buffer"="VC\r\n", "VISA resource name"=w2689) -> ("error out"=w2691:errorcluster, "read buffer"=w2685:string)  [unwired: 6 in]
                n1046 = Decimal String To Number(string=w2685) -> (number=w2684:i32)  [unwired: 2 in, 1 out]
                n1047 = Less Or Equal?(x=w2684, y=50) -> (x <= y?=w2682:bool)
                n1048 = property on="Status" class="Bool (strict)"("Value"=w2682) -> ()  [unwired: 2 in, 2 out]
                n1049 = case shown="True" w2682 {
                  tunnel: w2691 -> [w2693 w2716]
                  tunnel: w2689 -> [w2694 w2715]
                  tunnel: [w2694 w2706] -> w2688
                  tunnel: [w2693 w2700] -> w2687
                  frame False {
                  }
                  frame True {
                    n1050 = call <vilib>:"Clear Errors.vi"("error in (no error)"=w2716) -> ("error out"=w2717:errorcluster)  [unwired: 5 in, 1 out]
                    n1051 = control-ref of="ATR"() -> (w2703:refnum<vi>)
                    n1052 = VISA Flush I/O Buffer(VISA resource name=w2715, error in (no error)=w2717) -> (VISA resource name out=w2706:refnum<visa-resource-name>, error out=w2714:errorcluster)  [unwired: 1 in]
                    n1053 = call "Display Message to User2"("error in (no error)"=w2714) -> ("error out"=w2713:errorcluster, "Yes"=w2712:bool)  [unwired: 9 in]
                    n1054 = case shown="True" w2712 {
                      tunnel: w2713 -> [w2718 w2740]
                      tunnel: [w2718 w2719] -> w2711
                      tunnel: w2706 -> [_ w2737]
                      frame False {
                      }
                      frame True {
                        w2725 = FALSE ("2 Options")
                        n1055 = property on="UUT" class="DigNum (strict)"() -> ("Value"=w2739:u8)  [unwired: 2 in, 2 out]
                        n1056 = call "SetParam.vi"("RS"=TRUE, "error in (no error)"=w2740, "Param to Set in"=w2739, "Visa"=w2737) -> ("error out"=w2720:errorcluster)  [unwired: 7 in]
                        n1057 = control-ref of="Pannel User Message"() -> (w2736:refnum<vi>)
                        n1058 = control-ref of="Stop Burn-in"() -> (w2734:refnum<vi>)
                        n1059 = control-ref of="Stop Button"() -> (w2735:refnum<vi>)
                        n1060 = control-ref of="Motor Speed RPM"() -> (w2733:refnum<vi>)
                        n1061 = property on="VISA Tester" class="VISAName"() -> ("Value"=w2729:refnum<visa-resource-name>)  [unwired: 2 in, 2 out]
                        n1062 = call "TesterOption (SubVI).vi"("2 Options"=w2725, "error in (no error)"=w2720, "On/Off"=FALSE, "Tester Option"=T11."Power", "VISA Refnum in"=w2729) -> ("error out"=w2730:errorcluster, "VISA Refnum out"=w2732:refnum<visa-resource-name>)  [unwired: 5 in]
                        n1063 = call "Write panel message (SubVI).vi"("Stop BurnIn"=w2734, "rpm"=w2733, "PrintTime"=TRUE, "Stop"=w2735, "error in (no error)"=w2730, "Time to wait"=20.0, "Strin"="Restart the UUT\nPlease wait...", "String in"=w2736) -> ("error out"=w2731:errorcluster)  [unwired: 3 in]
                        n1064 = call "TesterOption (SubVI).vi"("2 Options"=w2725, "error in (no error)"=w2731, "On/Off"=FALSE, "Tester Option"=T11."Venable", "VISA Refnum in"=w2732) -> ("error out"=w2719:errorcluster)  [unwired: 5 in, 1 out]
                      }
                    }
                    n1065 = call "Find_Number_LineMARVIN.vi"("Test Paragraph"="7.5.5.1", "TableIn"=w2703) -> ("Line number"=w2704:i32)  [unwired: 3 in, 3 out]
                    n1066 = call "SerialMarvinSendGet.vi"("error in (no error)"=w2711, "write buffer"="SN\r\n", "VISA resource name"=w2706) -> ("error out"=w2707:errorcluster, "read buffer"=w2695:string)  [unwired: 7 in]
                    n1067 = call "SerialMarvinSendGet.vi"("error in (no error)"=w2707, "write buffer"="AO[1]\r\n", "VISA resource name"=w2706) -> ("error out"=w2701:errorcluster, "read buffer"=w2702:string)  [unwired: 7 in]
                    n1068 = Fract/Exp String To Number(string=w2702) -> (number=w2697:dbl)  [unwired: 3 in, 1 out]
                    n1069 = In Range and Coerce(upper limit=0.1 ("x"), x=w2697, lower limit=-0.1) -> (In Range?=w2696:bool)  [unwired: 1 out]
                    n1070 = call "PassOrFail (SubVI).vi"("index (row)"=w2704, "error in (no error)"=w2701, "Data in"=w2697, "Pass?Fail"=w2696, "Table in"=w2703) -> ("error out"=w2700:errorcluster)  [unwired: 6 in]
                    n1071 = property on="UUT SN Report" class="Str"("Value"=w2695) -> ()  [unwired: 2 in, 2 out]
                    n1072 = Decimal String To Number(string=w2695) -> (number=→"Current SN":i32)  [unwired: 2 in, 1 out]
                  }
                }
              }
            }
          }
          event "Refresh Button": Value Change {
            n1073 = event-data() -> ()  [unwired: 1 in, 6 out]
          }
          event "Settings": Value Change {
            n1074 = event-data() -> ()  [unwired: 1 in, 6 out]
            n1075 = control-ref of="VISA Tester"() -> (w2750:refnum<vi>)
            n1076 = control-ref of="UUT"() -> (w2748:refnum<vi>)
            n1077 = property on="Status" class="Bool (strict)"() -> ("Value"=w2752:bool)  [unwired: 2 in, 2 out]
            n1078 = case shown="True" w2752 {
              tunnel: w2758 -> [_ w2770]
              tunnel: [w2759 w2765] -> w2753
              tunnel: w2751 -> [_ w2764]
              tunnel: w2750 -> [_ w2763]
              tunnel: w2749 -> [_ w2762]
              tunnel: w2748 -> [_ w2761]
              frame False {
                n1079 = call "Display Message to User8"() -> ("error out"=w2759:errorcluster)  [unwired: 10 in, 1 out]
              }
              frame True {
                n1080 = vi-ref "Calibration (SubVI).vi"() -> (w2769:refnum<vi>)
                n1081 = invoke class="VI" method="FP.Open"(reference=w2769, error in=w2770, "Activate"=TRUE ("Activate?"), "State"=T23."Standard") -> (error out=w2766:errorcluster)  [unwired: 1 in, 4 out]
                n1082 = call "Calibration (SubVI).vi"("VISA UUT"=w2764, "error constant"=w2766, "UUT"=w2761, "CAN Cluster in"=w2762, "Visa Tester"=w2763) -> ("error constant 2"=w2765:errorcluster, "AO[1]Meas"=→"Cal":dbl)  [unwired: 5 in]
              }
            }
          }
        }
      }
      frame "Initialize" {
        w2774 = FALSE ("Visible")
        w2775 = FALSE ("Visible")
        w2776 = FALSE ("Visible")
        w2777 = FALSE ("Visible")
        w2789 = refnum<visa-resource-name> "COM1" ("VISA resource name")
        w2779 = FALSE ("Visible")
        w2771 = FALSE ("Serial Status")
        n1083 = disable-structure shown="Disabled" {
          frame Disabled {
            n1084 = local write "UUT"("" ("UUT")) -> ()
          }
          frame Enabled {
          }
        }
        n1085 = property on="ComTestResult" class="Bool (strict)"("Value"=w2777) -> ()  [unwired: 2 in, 2 out]
        n1086 = property on="VenableResult" class="Bool (strict)"("Value"=w2777) -> ()  [unwired: 2 in, 2 out]
        n1087 = property on="VenableDirectionResult" class="Bool (strict)"("Value"=w2777) -> ()  [unwired: 2 in, 2 out]
        n1088 = property on="SpeedResult" class="Bool (strict)"("Value"=w2777) -> ()  [unwired: 2 in, 2 out]
        n1089 = property on="Serial Com" class="Bool"(error in=errorcluster {"status"=FALSE, "code"=0, "source"=""} ("error out"), "Visible"=TRUE) -> (error out=w2791:errorcluster)  [unwired: 1 in, 1 out]
        n1090 = property on="AuxiOFFResult" class="Bool (strict)"("Value"=w2776) -> ()  [unwired: 2 in, 2 out]
        n1091 = property on="AuxiONResult" class="Bool (strict)"("Value"=w2776) -> ()  [unwired: 2 in, 2 out]
        n1092 = property on="VisualInspectionResult" class="Bool (strict)"("Value"=w2776) -> ()  [unwired: 2 in, 2 out]
        n1093 = property on="SensCalResult" class="Bool (strict)"("Value"=w2776) -> ()  [unwired: 2 in, 2 out]
        n1094 = property on="VISA Marvin" class="VISAName"(error in=w2791, "Visible"=w2779, "Value"=w2789) -> (error out=w2780:errorcluster)  [unwired: 1 in, 1 out]
        n1095 = property on="Stop Burn-in" class="Bool (strict)"(error in=w2780, "Visible"=w2779) -> (error out=w2772:errorcluster)  [unwired: 1 in, 1 out]
        n1096 = property on="BurnDC" class="Bool (strict)"("Value"=w2775) -> ()  [unwired: 2 in, 2 out]
        n1097 = property on="BurnTemp" class="Bool (strict)"("Value"=w2775) -> ()  [unwired: 2 in, 2 out]
        n1098 = property on="BurnSpeed" class="Bool (strict)"("Value"=w2775) -> ()  [unwired: 2 in, 2 out]
        n1099 = property on="BurnResult" class="Bool (strict)"("Value"=w2775) -> ()  [unwired: 2 in, 2 out]
        n1100 = property on="Refresh Button" class="Bool (strict)"(error in=w2772, "Value"=FALSE ("Refresh Button")) -> ()  [unwired: 1 in, 2 out]
        n1101 = property on="StopTimeResult" class="Bool (strict)"("Value"=w2774) -> ()  [unwired: 2 in, 2 out]
        n1102 = property on="MotorTempResult" class="Bool (strict)"("Value"=w2774) -> ()  [unwired: 2 in, 2 out]
        n1103 = property on="TempControlResult" class="Bool (strict)"("Value"=w2774) -> ()  [unwired: 2 in, 2 out]
        n1104 = property on="Automation" class="Bool (strict)"("Value"=w2774) -> ()  [unwired: 2 in, 2 out]
        n1105 = flat-sequence {
          tunnel: w2772 -> [w2794]
          tunnel: [w2793] -> w2787
          tunnel: [w2796] -> w2786
          tunnel: w2787 -> [w2796]
          tunnel: [w2809] -> w2785
          tunnel: w2786 -> [w2810]
          tunnel: [w2810] -> w2784
          frame #0 {
            n1106 = control-ref of="This VI"() -> (w2795:refnum<vi>)
            n1107 = invoke class="VI" method="Default Vals.Reinit All"(reference=w2795, error in=w2794) -> (error out=w2793:errorcluster)  [unwired: 1 in, 2 out]
          }
          frame #1 {
            w2800 = u32 4294967295  # AccMask
            w2799 = T4 0 items=["使用Flash参数", "使用界面设置参数"] ("InitFlag")
            w2797 = T6 0 items=["normal operation", "Listen-only mode", "test mode"]  # Mode
            w2798 = T5 3 items=["接收所有类型"=1, "只接收标准帧"=2, "只接收扩展帧"=3] ("Fliter")
            w2804 = u8 10 items=["5k bps"=1, "10k bps"=2, "20k bps"=3, "40k bps"=4, "50k bps"=5, "80k bps"=6, "100k bps"=7, "125k bps"=8, "200k bps"=9, "250k bps"=10, "400k bps"=11, "500k bps"=12, "666k bps"=13, "800k bps"=14, "1000k bps"=15, "33.33k bps"=16, "66.66k bps"=17, "83.33k bps"=18]  # kBaudRate
            w2801 = u32 0  # AccCode
            w2802 = T2 4 items=["USB-CAN"=3, "USB-CAN2"=4] ("DevType")
            w2803 = T7 {"DevType"=3, "DevIndex"=0, "CanIndex"=0, "VCI_INIT_CONFIG"={"AccCode"=0, "AccMask"=0, "InitFlag"=1, "Fliter"=7, "Timing0"=0, "Timing1"=0, "Mode"=0}}  # Config
            # "CANalystII"
            n1108 = call "Demo_GetT0T1.vi"("kBaudRate"=w2804) -> ("Timing0"=w2806:u8, "Timing1"=w2807:u8)
            n1109 = Bundle By Name(cluster=w2803, "DevType"=w2802, "CanIndex"="Channel 2", "VCI_INIT_CONFIG.AccCode"=w2801, "VCI_INIT_CONFIG.AccMask"=w2800, "VCI_INIT_CONFIG.InitFlag"=w2799, "VCI_INIT_CONFIG.Fliter"=w2798, "VCI_INIT_CONFIG.Timing0"=w2806, "VCI_INIT_CONFIG.Timing1"=w2807, "VCI_INIT_CONFIG.Mode"=w2797) -> (→"Config_CANAT":T7)
          }
          frame #2 {
            w2811 = u16 284 items=["1M"=20, "500K"=28, "250K"=284, "125K"=796, "100K"=17199, "50K"=18223, "20K"=21295, "10K"=26415, "5K"=32639] ("baud in")
            n1110 = control-ref of="Config_CANAT"() -> (w2809:refnum<vi>)
            n1111 = call "InitCAN_ATII.vi"("Config"=w2809) -> ("Sts"=→"CAN Status":bool)
            n1112 = call "ChangeCANBaud.vi"("baud in"=w2811, "reference"=w2809) -> ()
          }
        }
        "Status" <- w2771
        "Test Failed" <- w2771
      }
    }
  }
  n1113 = property on="Settings" class="Bool (strict)"("Visible"=w3) -> ()  [unwired: 2 in, 2 out]
  n1114 = property on="Cal" class="DigNum (strict)"("Visible"=w3) -> ()  [unwired: 2 in, 2 out]
  n1115 = disable-structure shown="Disabled" {
    frame Disabled {
      w2814 = T18."Disabled and Grayed Out" ("Disabled")
      w2815 = FALSE ("Start")
      n1116 = property on="VISA Tester" class="VISAName" props=["Value"]() -> ()  [unwired: 2 in, 3 out]
      n1117 = property on="Current SN" class="DigNum (strict)" props=["Value"]() -> ()  [unwired: 2 in, 3 out]
      n1118 = property on="UUT" class="DigNum (strict)" props=["Value"]() -> ()  [unwired: 2 in, 3 out]
      n1119 = property on="Status" class="Bool (strict)" props=["Value"]() -> ()  [unwired: 2 in, 3 out]
      n1120 = property on="UUT SoftwareVer" class="Str" props=["Value"]() -> ()  [unwired: 2 in, 3 out]
      n1121 = property on="Next SN" class="DigNum (strict)" props=["Value"]() -> ()  [unwired: 3 in, 2 out]
      n1122 = property on="Start" class="Bool (strict)"("Value"=w2815, "DisabledEnum"=w2814) -> ()  [unwired: 2 in, 2 out]
      n1123 = property on="Report" class="Bool (strict)"("Value"=w2815, "DisabledEnum"=w2814) -> ()  [unwired: 2 in, 2 out]
    }
    frame Enabled {
    }
  }
  n1124 = disable-structure shown="Disabled" {
    frame Disabled {
      (unwired) 0.02003173828125 ("x")
      n1125 = control-ref of="Stop Burn-in"() -> ()  [unwired: 1 out]
      n1126 = control-ref of="Stop Button"() -> ()  [unwired: 1 out]
      n1127 = control-ref of="Motor Speed RPM"() -> ()  [unwired: 1 out]
      n1128 = control-ref of="Config_CANAT"() -> ()  [unwired: 1 out]
      n1129 = control-ref of="UUT"() -> ()  [unwired: 1 out]
      n1130 = call "GetADCTester (SubVI).vi"() -> ()  [unwired: 9 in, 3 out]
      n1131 = call "CANSendMotorSpeed.vi"() -> ()  [unwired: 11 in, 1 out]
      n1132 = control-ref of="Config_CANAT"() -> ()  [unwired: 1 out]
      n1133 = call "Find_Number_LineMARVIN.vi"() -> ()  [unwired: 5 in, 4 out]
      n1134 = property on="UUT" class="DigNum (strict)" props=["Value"]() -> ()  [unwired: 2 in, 3 out]
      n1135 = control-ref of="UUT"() -> ()  [unwired: 1 out]
      n1136 = call "DegToDAC (SubVI).vi"() -> ()  [unwired: 10 in, 2 out]
      n1137 = call "Write panel message (SubVI).vi"() -> ()  [unwired: 11 in, 1 out]
      n1138 = property on="VISA Tester" class="VISAName" props=["Value"]() -> ()  [unwired: 2 in, 3 out]
      n1139 = control-ref of="ATR"() -> ()  [unwired: 1 out]
      n1140 = call "TesterOption (SubVI).vi"() -> ()  [unwired: 10 in, 2 out]
      n1141 = call "TesterOption (SubVI).vi"() -> ()  [unwired: 10 in, 2 out]
      n1142 = call "PassOrFail (SubVI).vi"() -> ()  [unwired: 11 in, 1 out]
    }
    frame Enabled {
    }
  }
  n1143 = disable-structure shown="Disabled" {
    frame Disabled {
      n1144 = flat-sequence {
        frame #0 {
          n1145 = call "CANSendMotorSpeed.vi"("Remote"=TRUE, "Motor Speed RPM"=u16 0) -> ("error out"=w2817:errorcluster, "UUT"=w2820:refnum<vi>)  [unwired: 8 in]
          n1146 = property on="VISA Tester" class="VISAName"() -> ("Value"=w2816:refnum<visa-resource-name>)  [unwired: 2 in, 2 out]
          n1147 = call "TesterOption (SubVI).vi"("error in (no error)"=w2817, "On/Off"=FALSE, "Tester Option"=T11."Power", "VISA Refnum in"=w2816) -> ()  [unwired: 6 in, 2 out]
        }
      }
    }
    frame Enabled {
    }
  }
  "Pannel User Message" <- w1
